vi "Telemetry2022.vi"() -> ()   [LabVIEW 2017]
uses:
  <vilib>/xnet/xnet.llb/XNET Frame CAN.ctl
  <vilib>/xnet/xnet.llb/XNET Frame Type CAN.ctl
  <vilib>/Instr/_visa.llb/VISA Configure Serial Port (Instr).vi
  <vilib>/xnet/xnet.llb/XNET Read (Frame CAN).vi
  <resource>/objmgr/xnet.rc
panel:
  out "x-y":u8
  out "serial in 2":u8[][](array[numeric]) format="%x"
  out "deleted portion 2":u8[](array[numeric]) format="%x"
  out "buffer":string
  out "Car orient":dbl
  out "Car pos":dbl[](array[numeric])
  out "Temp inv FL":dbl
  in  "ID":i32
  in  "Volt id":i32
  out "HV Volt Alert":bool
  out "HV Temp Alert":bool
  in  "Temp":dbl=45.0
  in  "Voltage [mV]":dbl=4200.0
  in  "Temp Id":i32
  out "Temp inv RR":dbl
  out "Temp inv RL":dbl
  out "Temp inv FR":dbl
  out "signal names":string[](array[string])
  in  "Signal indexes":T1
  in  "?":T2(tab)
  in  "Start Telemetry":bool
  in  "Data source":u16(ring) items=["WiFi-UDP", "XNET-USB", "CAN-USB", "Log Replay", "Serial"]
  in  "Main timestep":u32=2
  out "Is running":bool
  out "CAN2 Frame to signal":errorcluster
  out "CAN1 Frame to signal":errorcluster
  out "XNET error (Intf 2)":errorcluster
  out "XNET error (Intf 1)":errorcluster
  out "NI-CAN1 error":errorcluster {"code" format="%.0x"}
  out "NI-CAN0 error":errorcluster {"code" format="%.0x"}
  out "UDP Read error":errorcluster
  in  "Port":u16=8998
  out "Discarding":bool
  out "Discard count":i32
  out "Key Navigation error":errorcluster
  in  "Reset Keyboard":bool
  out "Key":T3(ring)
  out "Actual Timestep":u32(graph)
  out "Frames read":i32(graph)
  out "serial error":errorcluster
  in  "timeout ms":u32=1000
  in  "baud":u32=230400
  in  "Port":refnum<visa-resource-name>
  in  "Enable Termination\nChar":bool
  in  "termination char\n(0xA = '\\n' = LF)":u8=10 format="%.0x"
  in  "stop bits":u16(ring)=10 items=["1.0"=10, "1.5"=15, "2.0"=20]
  in  "data bits":u16=8 min=5 max=8 step=1
  in  "max buffer size":u32=200
  in  "parity":u16(ring) items=["None", "Odd", "Even", "Mark", "Space"]
  in  "flow control":T4(ring)
  out "RSSI [dBm]":i16
  out "Intf2":refnum<k21>
  out "Intf1":refnum<k21>
  out "Active intfs":i32
  out "APPS 1":dbl
  out "APPS 2":dbl
  out "BPS Rear":dbl
  out "BPS Front":dbl
  out "STA 2":dbl
  out "STA 1":dbl
  out "PPS 2":dbl
  out "PPS 1":dbl
  out "Dial4":i8(knob) scale=1.0..12.0
  out "Dial3":i8(knob) scale=1.0..12.0
  out "Dial2":i8(knob) scale=1.0..12.0
  out "Dial1":i8(knob) scale=1.0..12.0
  out "Dial5":i8(knob) scale=1.0..12.0
  out "Steering display":string
  out "Boolean 4":bool
  out "Boolean 3":bool
  out "Boolean 2":bool
  out "Boolean":bool
  out "Drv Torque Mult":dbl
  out "Brk Torque Mult":dbl
  out "Yaw Ctrl P":dbl
  out "Power Max":dbl
  out "Yaw Ctrl Balance":dbl
  out "Torque Demand":dbl
  out "FL Torque Limit":dbl
  out "FR Torque Limit":dbl
  out "RL Torque Limit":dbl
  out "RR Torque Limit":dbl
  out "FlashSubzoneError":bool=TRUE
  out "CSR2OtpError":bool=TRUE
  out "CSR1OtpError":bool=TRUE
  out "Output2OvpError":bool=TRUE
  out "Output1OvpError":bool=TRUE
  out "LVUvpInError":bool=TRUE
  out "LVUvpAlimAuxError":bool=TRUE
  out "LVOvpInError":bool=TRUE
  out "HVOcpError":bool=TRUE
  out "HVError":bool=TRUE
  out "CANError":bool=TRUE
  out "BB3OtpError":bool=TRUE
  out "BB2OtpError":bool=TRUE
  out "BB1OtpError":bool=TRUE
  out "STA2_OV":u8(slide) scale=0.0..180.0
  out "STA1_OV":u8(slide) scale=0.0..180.0
  out "PPS2_OV":u8(slide) scale=0.0..10.0
  out "PPS1_OV":u8(slide) scale=0.0..10.0
  out "APPS2_OV":u8(slide) scale=0.0..100.0
  out "APPS1_OV":u8(slide) scale=0.0..100.0
  out "BPS_rear_OV":u8(slide) scale=0.0..700.0
  out "BPS_front_OV":u8(slide) scale=0.0..700.0
  out "SC ENDLINE":dbl
  out "BFS [N]":dbl
  out "Place Opened":string
  out "BPSR_bool_OV":bool
  out "BPSF_bool_OV":bool
  out "BFS_bool_OV":bool
  out "STA_plaus":bool
  out "APPS_plaus":bool
  out "APPS1_bool":bool
  out "APPS2_bool":bool
  out "STA1_bool":bool
  out "STA2_bool":bool
  out "Speed [km/h]":dbl(knob) scale=0.0..110.0
  out "ASMS":bool
  out "RES GO":bool
  out "ASSI State":string
  out "AS State":string
  out "Car State":string
  out "RR":dbl[](array[numeric])
  out "FL":dbl[](array[numeric])
  out "FR":dbl[](array[numeric])
  out "RL":dbl[](array[numeric])
  out "Actual_vel_FL_OV":dbl
  out "Actual_vel_FR_OV":dbl
  out "Actual_vel_RL_OV":dbl
  out "Actual_vel_RR_OV":dbl
  out "Accel X":dbl
  out "Accel Y":dbl
  out "Yaw rate":dbl
  out "g-g Graph":cluster{dbl[], dbl[]}[](graph)
  out "HV":u32(colorbox)=9868950
  out "IMD":u32(colorbox)=9868950
  out "AMS":u32(colorbox)=9868950
  out "ASB":u32(colorbox)=9868950
  out "MCU1":u32(colorbox)=9868950
  out "MCU3":u32(colorbox)=9868950
  out "MCU4":u32(colorbox)=9868950
  out "MCU2":u32(colorbox)=9868950
  out "TCU":u32(colorbox)=9868950
  out "TS OFF":u32(colorbox)=9868950
  out "SoC":dbl
  out "HV Power out":dbl
  out "Max Temp":dbl
  out "Min Voltage":dbl
  out "VDC DV mode":bool
  out "RSSI [dBm]":i16
  out "EPOS Status":dbl
  out "EPOS Torque":dbl
  out "EPOS Position":dbl
  out "MCU State":string
  out "EPOS State":string
  out "RR Target Velocity":dbl
  out "FR Target Velocity":dbl
  out "RL Target Velocity":dbl
  out "FL Target Velocity":dbl
  out "Slip Ctrl I":dbl
  out "Optimal Slip":dbl
  out "Slip Ctrl D":dbl
  out "Slip Ctrl P":dbl
  out "Track Length":dbl
  out "Laps":dbl
  out "Target Soc":dbl
  out "Velocity X [km/h]":dbl
  out "Powlim Efficiency":bool
  out "Powlim Torque":bool
  out "Powlim Throttle":bool
  out "Powlim Hardcore":bool
  out "Traction Ctrl On":bool
  out "Slip Ctrl On":bool
  out "RR Torque Limit -":dbl
  out "RR Torque Limit +":dbl
  out "RL Torque Limit -":dbl
  out "RL Torque Limit +":dbl
  out "FR Torque Limit +":dbl
  out "FR Torque Limit -":dbl
  out "FL Torque Limit -":dbl
  out "FL Torque Limit +":dbl
  out "Target Steer":dbl(graph)
  out "Torque":T5(graph)
  out "Torque Demand":dbl(graph)
  out "Fz FL":dbl
  out "Fz FR":dbl
  out "Fz RL":dbl
  out "Fz RR":dbl
  out "Safety mode":bool
  out "M Yaw Limit":dbl
  out "M Yaw":dbl
  out "Yaw Ctrl Weight":dbl
  out "Drv Torque Mult":dbl
  out "Brk Torque Mult":dbl
  out "Yaw Ctrl P":dbl
  out "Yaw Ctrl Balance":dbl
  out "Efficiency Tune":dbl
  out "Launch Ctrl Mu":dbl
  out "Drop Param":dbl
  out "Drop Param New":dbl
  out "TC Threshold":dbl
  out "Powlim Approx":dbl
  out "Power Max":dbl
  out "RPM Max":dbl
  out "Max Motor Torque":dbl
  out "Lateral Balance":dbl
  out "Brake Force Max":dbl
  out "Throttle Breakpoint":dbl
  out "Static Weight Dist":dbl
  out "TCU CPU Usage":dbl
  out "Temp Inv RR":dbl
  out "Temp Inv RL":dbl
  out "Temp Inv FR":dbl
  out "Temp Inv FL":dbl
  out "Temp Motor RR":dbl
  out "Temp IGBT RR":dbl
  out "Error info RR":dbl
  out "Im RR":dbl
  out "It RR":dbl
  out "Temp Motor RL":dbl
  out "Temp IGBT RL":dbl
  out "Error info RL":dbl
  out "Im RL":dbl
  out "It RL":dbl
  out "Temp Motor FR":dbl
  out "Temp IGBT FR":dbl
  out "Error info FR":dbl
  out "Im FR":dbl
  out "It FR":dbl
  out "Temp Motor FL":dbl
  out "Temp IGBT FL":dbl
  out "Error info FL":dbl
  out "Im FL":dbl
  out "It FL":dbl
  out "RR Status":bool[](array[boolean])
  out "RR Inverter On":bool
  out "RR Error Reset":bool
  out "RR Enable":bool
  out "RR DC On":bool
  out "RL Status":bool[](array[boolean])
  out "RL Inverter On":bool
  out "RL Error Reset":bool
  out "RL Enable":bool
  out "RL DC On":bool
  out "FR Status":bool[](array[boolean])
  out "FR Inverter On":bool
  out "FR Error Reset":bool
  out "FR Enable":bool
  out "FR DC On":bool
  out "FL Status":bool[](array[boolean])
  out "FL Inverter On":bool
  out "FL Error Reset":bool
  out "FL Enable":bool
  out "FL DC On":bool
  out "Temp Inverter °C":T5(graph)
  out "MCU Actual Velocity 1/min":T5(graph)
  out "SC ENDLINE":dbl
  out "BSPD Actual":bool=TRUE
  out "DV Actual":bool=TRUE
  out "DV RELAY Actual":bool=TRUE
  out "EBS Actual":bool=TRUE
  out "FRONT Actual":bool=TRUE
  out "HOOP Actual":bool=TRUE
  out "MCU Actual":bool=TRUE
  out "BSPD Stored":bool
  in  "Ack BPSD":bool
  out "DV Stored":bool
  in  "Ack DV":bool
  out "DV RELAY Stored":bool
  in  "Ack DV RELAY":bool
  out "EBS Stored":bool
  in  "Ack EBS":bool
  out "FRONT Stored":bool
  in  "Ack FRONT":bool
  out "HOOP Stored":bool
  in  "Ack HOOP":bool
  out "MCU Stored":bool
  in  "Ack MCU":bool
  out "Temp SR2":dbl
  out "Temp SR1":dbl
  out "Temp BB3":dbl
  out "Temp BB2":dbl
  out "Temp BB1":dbl
  out "LV mAh":dbl
  out "Current IO Unbalance":dbl
  out "Output Overload Count":dbl
  out "HV Current In":dbl
  out "HV Voltage In":dbl
  out "CH1 Requested":bool
  out "CH2 Requested":bool
  out "Regen On":bool
  out "Umbilical On":bool
  out "CH1 Current Limit":dbl
  out "CH2 Current Limit":dbl
  out "HV Current Limit":dbl
  out "HV Voltage Setpoint":dbl
  out "CH2 Voltage Setpoint":dbl
  out "CH1 Voltage Setpoint":dbl
  out "Current Out Min 1":dbl
  out "Current Out Max 1":dbl
  out "Voltage Out Min 1":dbl
  out "Voltage Out Max 1":dbl
  out "Current Out Min 2":dbl
  out "Current Out Max 2":dbl
  out "Voltage Out Min 2":dbl
  out "Voltage Out Max 2":dbl
  out "Channel powers":cluster{dbl, dbl}(graph)={-0.16021728515625, 0.50628662109375}
  out "Channel voltages":cluster{dbl, dbl}(graph)={-0.16021728515625, 0.50628662109375}
  out "Channel currents":cluster{dbl, dbl}(graph)={-0.16021728515625, 0.50628662109375}
  out "HVDET2":bool
  out "PC Error":bool=TRUE
  out "TS-OV":bool
  out "IMD Relay":bool
  out "AMS Relay":bool
  out "AIR-":bool
  out "TSAL":bool
  out "TS-OC":bool
  out "AIR+":bool
  out "HVDET":bool
  out "AMS Error":bool=TRUE
  out "IMD Error":bool=TRUE
  out "TSAL Error":bool=TRUE
  out "OT":bool
  out "UV":bool
  out "OV":bool
  in  "HV T Alert":bool
  in  "Alert Max [xC]":dbl=450.0
  in  "HV V Alert":bool
  in  "Alert Max [xV]":dbl=4200.0
  in  "Alert Min [xV]":dbl
  out "Temp 8":dbl[](array[numeric])
  out "Temp 7":dbl[](array[numeric])
  out "Cell 6":cluster{"V-Value":dbl, dbl}[](array[cluster]) {"V-Slide" scale=0.0..6000.0}
  out "Temp 6":dbl[](array[numeric])
  out "Cell 5":cluster{"V-Value":dbl, dbl}[](array[cluster]) {"V-Slide" scale=0.0..6000.0}
  out "Temp 5":dbl[](array[numeric])
  out "Cell 4":cluster{"V-Value":dbl, dbl}[](array[cluster]) {"V-Slide" scale=0.0..6000.0}
  out "Temp 4":dbl[](array[numeric])
  out "Temp 3":dbl[](array[numeric])
  out "Cell 3":cluster{"V-Value":dbl, dbl}[](array[cluster]) {"V-Slide" scale=0.0..6000.0}
  out "Temp 2":dbl[](array[numeric])
  out "Cell 2":cluster{"V-Value":dbl, dbl}[](array[cluster]) {"V-Slide" scale=0.0..6000.0}
  out "Temp":dbl[](array[numeric])
  out "Cell":cluster{"V-Value":dbl, dbl}[](array[cluster]) {"V-Slide" scale=0.0..6000.0}
  out "Min Voltage Calc":dbl
  out "Max Temp Calc":dbl
  out "Min Voltage":dbl
  out "Max Temp":dbl
  out "Max Voltage":dbl
  out "SoC [mAh]":dbl
  out "Before":dbl
  out "After":dbl
  out "HV Current":dbl
  out "Charging State":string
  out "Heatmap":u32[][](array[colorbox])
  in  "Colors":u32[](array[colorbox])=[16448250, 16860, 711680, 16776960, 16025344, 16711680, 16189919, 0]
  in  "Ranges":i32[](array[numeric])=[1, 20, 30, 35, 40, 45, 50]
  in  "OK Button":bool
  out "Yaw Rear Vectornav":dbl
  out "AccY Rear":dbl
  out "AccX Rear":dbl
  out "BPS_Graph":cluster{dbl, dbl}(graph)={-0.16021728515625, 0.50628662109375}
  out "Target vs Actual steer\nSteer":cluster{dbl, dbl}(graph)={-0.16021728515625, 0.50628662109375}
  out "Target vs Actual Velocity":cluster{dbl, dbl}(graph)={-0.16021728515625, 0.50628662109375}
  out "HV Power out [W]":dbl(graph)
  out "Plausability":bool
  out "Validity":bool=TRUE
  out "APPS Avg":u8(slide) scale=0.0..100.0
  out "BFS_graph [N]":dbl(graph)
  out "STA Avg":u8(slide) scale=0.0..210.0
  out "Plausability":bool
  out "Validity":bool=TRUE
  out "g-g Graph 3":cluster{dbl[], dbl[]}[](graph)
  out "AccX Front":dbl
  out "AccY Front":dbl
  out "Roll Front":dbl
  out "Yaw Front":dbl
  out "Yaw Rear":dbl
  out "HV Current graph":dbl(graph)
  out "BFS Offset":dbl
  out "BPS Rear":dbl
  out "STA2":dbl
  out "APPS2":dbl
  out "PPS2":dbl
  out "BPS Front":dbl
  out "STA1":dbl
  out "APPS1":dbl
  out "PPS1":dbl
  out "STA2 Validity":bool
  out "APPS1 Validity":bool
  out "APPS2 Validity":bool
  out "STA1 Validity":bool
  out "BFS Validity":bool
  out "BPS Front Validity":bool
  out "BPS Rear Validity":bool
  out "XLAT":bool
  out "MODE":bool
  out "BLANK":bool
  out "START":bool
  out "ON":bool
  out "OFF":bool
  out "MCU Rear":bool
  out "MCU Front":bool
  out "MCU RF":bool
  out "MCU EF":bool
  out "TCU Heartbeat Error":bool=TRUE
  out "Steering Heartbeat Error":bool=TRUE
  out "Pedal Node Heartbeat Error":bool=TRUE
  out "MCU Heartbeat Error":bool=TRUE
  out "HVECU Heartbeat Error":bool=TRUE
  out "Dash Heartbeat Error":bool=TRUE
  out "HV":u32(colorbox)=9868950
  out "IMD":u32(colorbox)=9868950
  out "AMS":u32(colorbox)=9868950
  out "ASB":u32(colorbox)=9868950
  out "MCU1":u32(colorbox)=9868950
  out "MCU3":u32(colorbox)=9868950
  out "MCU4":u32(colorbox)=9868950
  out "MCU2":u32(colorbox)=9868950
  out "TCU":u32(colorbox)=9868950
  out "TS OFF":u32(colorbox)=9868950
  out "Brake Light":bool
  out "STA1 Max":dbl
  out "STA1 Min":dbl
  out "STA2 Max":dbl
  out "STA2 Min":dbl
  out "APPS1 Max":dbl
  out "APPS1 Min":dbl
  out "APPS2 Max":dbl
  out "APPS2 Min":dbl
  out "SC ENDLINE":dbl
  out "Rotary5 Timeout":bool=TRUE
  out "Rotary4 Timeout":bool=TRUE
  out "Rotary1 Timeout":bool=TRUE
  out "Rotary2 Timeout":bool=TRUE
  out "Rotary3 Timeout":bool=TRUE
  out "Rotary5 Validity":bool=TRUE
  out "Rotary4 Validity":bool=TRUE
  out "Rotary3 Validity":bool=TRUE
  out "Rotary2 Validity":bool=TRUE
  out "Rotary1 Validity":bool=TRUE
  out "Button4 Validity":bool=TRUE
  out "Button3 Validity":bool=TRUE
  out "Button2 Validity":bool=TRUE
  out "Button1 Validity":bool=TRUE
  out "BFS Timeout":bool=TRUE
  out "APPS2 Timeout":bool=TRUE
  out "APPS1 Timeout":bool=TRUE
  out "BPS Rear Timeout":bool=TRUE
  out "AccY Rear Timeout":bool=TRUE
  out "AccY FrontTimeout":bool=TRUE
  out "BPS Front Timeout":bool=TRUE
  out "AccX Rear Timeout":bool=TRUE
  out "AccX Front Timeout":bool=TRUE
  out "SC Endline Timeout":bool=TRUE
  out "ASB Error":bool=TRUE
  out "SC Endline Validity":bool=TRUE
  out "HV Current Timeout":bool=TRUE
  out "HV Cell Temp Timeout":bool=TRUE
  out "SC Endline":bool=TRUE
  out "OT":bool=TRUE
  out "OV":bool=TRUE
  out "UV":bool=TRUE
  out "HV Cell Temp Validity":bool=TRUE
  out "HV Cell Voltage Validity":bool=TRUE
  out "IMD Error":bool=TRUE
  out "AMS Error":bool=TRUE
  out "PC Error":bool=TRUE
  out "TSAL Error":bool=TRUE
  out "HV Current Validity":bool=TRUE
  out "HV Voltage Validity":bool=TRUE
  out "AccY Rear Validity":bool=TRUE
  out "Accy Front Validity":bool=TRUE
  out "APPS1 Validity":bool=TRUE
  out "STA1 Validity":bool=TRUE
  out "BPS Front Validity":bool=TRUE
  out "AccX Rear Validity":bool=TRUE
  out "AccX Front Validity":bool=TRUE
  out "STA Plausability":bool
  out "APPS Plausability":bool
  out "BFS Validity":bool=TRUE
  out "APPS2 Validity":bool=TRUE
  out "STA2 Validity":bool=TRUE
  out "Yaw Front Validity":bool=TRUE
  out "Yaw Rear Validity":bool=TRUE
  out "BPS Rear Validity":bool=TRUE
  out "FL Error info":dbl
  out "FR Error info":dbl
  out "RL Error info":dbl
  out "RR Error info":dbl
  out "FlashSubzoneError":bool=TRUE
  out "CSR2OtpError":bool=TRUE
  out "CSR1OtpError":bool=TRUE
  out "Output2OvpError":bool=TRUE
  out "Output1OvpError":bool=TRUE
  out "LVUvpInError":bool=TRUE
  out "LVUvpAlimAuxError":bool=TRUE
  out "LVOvpInError":bool=TRUE
  out "HVOcpError":bool=TRUE
  out "HVError":bool=TRUE
  out "CANError":bool=TRUE
  out "BB3OtpError":bool=TRUE
  out "BB2OtpError":bool=TRUE
  out "BB1OtpError":bool=TRUE
  out "DV Target Angle Validity":bool=TRUE
  out "SSG Status1 Timeout":bool=TRUE
  out "DV Target Speed Validity":bool=TRUE
  out "Xavier Timeout":bool=TRUE
  out "Bag Start":bool
  out "Loop Closed":bool
  out "Mission Finished":bool
  out "Eff n Particles":dbl
  out "Updates last resample":dbl
  out "Runtime":dbl
  out "HeadingSS-Yaw":cluster{"Data":dbl, "Data":dbl}(graph)
  out "Heading-Steering-Crosstrack":cluster{"Data":dbl, "Data":dbl, "Data":dbl}(graph)
  out "Target laps":dbl
  out "Current laps":dbl
  out "Xavier Power [W]":dbl
  out "Xavier Max Temp [°C]":dbl
  out "CPU8":u8(slide) scale=0.0..100.0
  out "CPU7":u8(slide) scale=0.0..100.0
  out "CPU6":u8(slide) scale=0.0..100.0
  out "CPU5":u8(slide) scale=0.0..100.0
  out "CPU4":u8(slide) scale=0.0..100.0
  out "CPU3":u8(slide) scale=0.0..100.0
  out "CPU2":u8(slide) scale=0.0..100.0
  out "CPU1":u8(slide) scale=0.0..100.0
  out "RAM":u8(slide) scale=0.0..31.0
  out "Initial Checkup":string
  out "Mission selected":string
  out "Car State":string
  out "ASSI State":string
  out "AS State":string
  out "Driving State Active":bool
  out "nEBS Acitve":bool
  out "EBS Active":bool
  out "Finish State":bool
  out "Target Steer 2":dbl(graph)
  out "Target Speed":dbl(graph)
  out "ASMS":bool
  out "ASB":u32(colorbox)=9868950
  out "Inspection":u32(colorbox)=9868950
  out "Skidpad":u32(colorbox)=9868950
  out "Trackdrive":u32(colorbox)=9868950
  out "Red count":dbl
  out "Orange count":dbl
  out "Blue count":dbl
  out "Yellow count":dbl
  out "Current landmarks":dbl
  out "All landmarks":dbl
  out "Map":cluster{dbl[], dbl[]}[](graph)
  in  "Arrow thickness":dbl=0.15 format="%#_13g"
  in  "Arrow size":dbl=5.0 format="%#_13g"
  in  "Export":bool
  out "Lap                    Laptime                        SoC                 Current Avg |                             Motor Temperatures                            |                            Inverter Temperatures":T6(array[cluster]) {"Laptime" format="%<%M:%S%2u>T"}
  in  "Laptrigger":bool
  in  "Reset":bool
  in  "Lapdata disp":bool=TRUE
  out "Inverter Temp":cluster{i32[], dbl[]}[](graph)
  out "Motor Temp":cluster{i32[], dbl[]}[](graph)
  # "STA1"
  # "STA2"
  # "PPS\n1      2"
  # "APPS\n1      2"
  # "BPS\nF      R"
  # "APPS1"
  # "APPS2"
  # "STA1"
  # "STA2"
  # "BFS"
  # "BPS F"
  # "BPS R"
  # "Error Info"
  # "Temp IGBT °C"
  # "Temp Inverter °C"
  # "Temp Motor °C"
  # "Actual Velocity [rpm]"
  # "SysReady"
  # "Error"
  # "Warn"
  # "QuitDcOn"
  # "DcOn"
  # "QuitInvOn"
  # "InverterOn"
  # "Derating"
  # "SysReady"
  # "Error"
  # "Warn"
  # "QuitDcOn"
  # "DcOn"
  # "QuitInvOn"
  # "InverterOn"
  # "Derating"
  # "SysReady"
  # "Error"
  # "Warn"
  # "QuitDcOn"
  # "DcOn"
  # "QuitInvOn"
  # "InverterOn"
  # "Derating"
  # "SysReady"
  # "Error"
  # "Warn"
  # "QuitDcOn"
  # "DcOn"
  # "QuitInvOn"
  # "InverterOn"
  # "Derating"
  # "-inf"
  # "inf"
  # "-"
  # "+"
  # "-"
  # "-"
  # "+"
  # "+"
  # "-"
  # "-"
  # "+"
  # "+"
  # "-"
  # "-"
  # "+"
  # "+"
  # "-"
  # "-"
  # "+"
  # "+"
  # "-"
  # "-"
  # "+"
  # "+"
  # "-"
  # "-"
  # "+"
  # "ADCs"
  # "Sensors"
  # "Dashboard"
  # "MCU"
  # "Heartbeats"
  # "System"
  # "EEPROMS"
  # "Brightloop"
  # "Sensor validity"
  # "HV Errors"
  # "Steering wheel"
  # "Sensor Timeout"
  # "System"
  # "AMK Errors"
  # "1         CPU Usage         8"
  # "RAM"
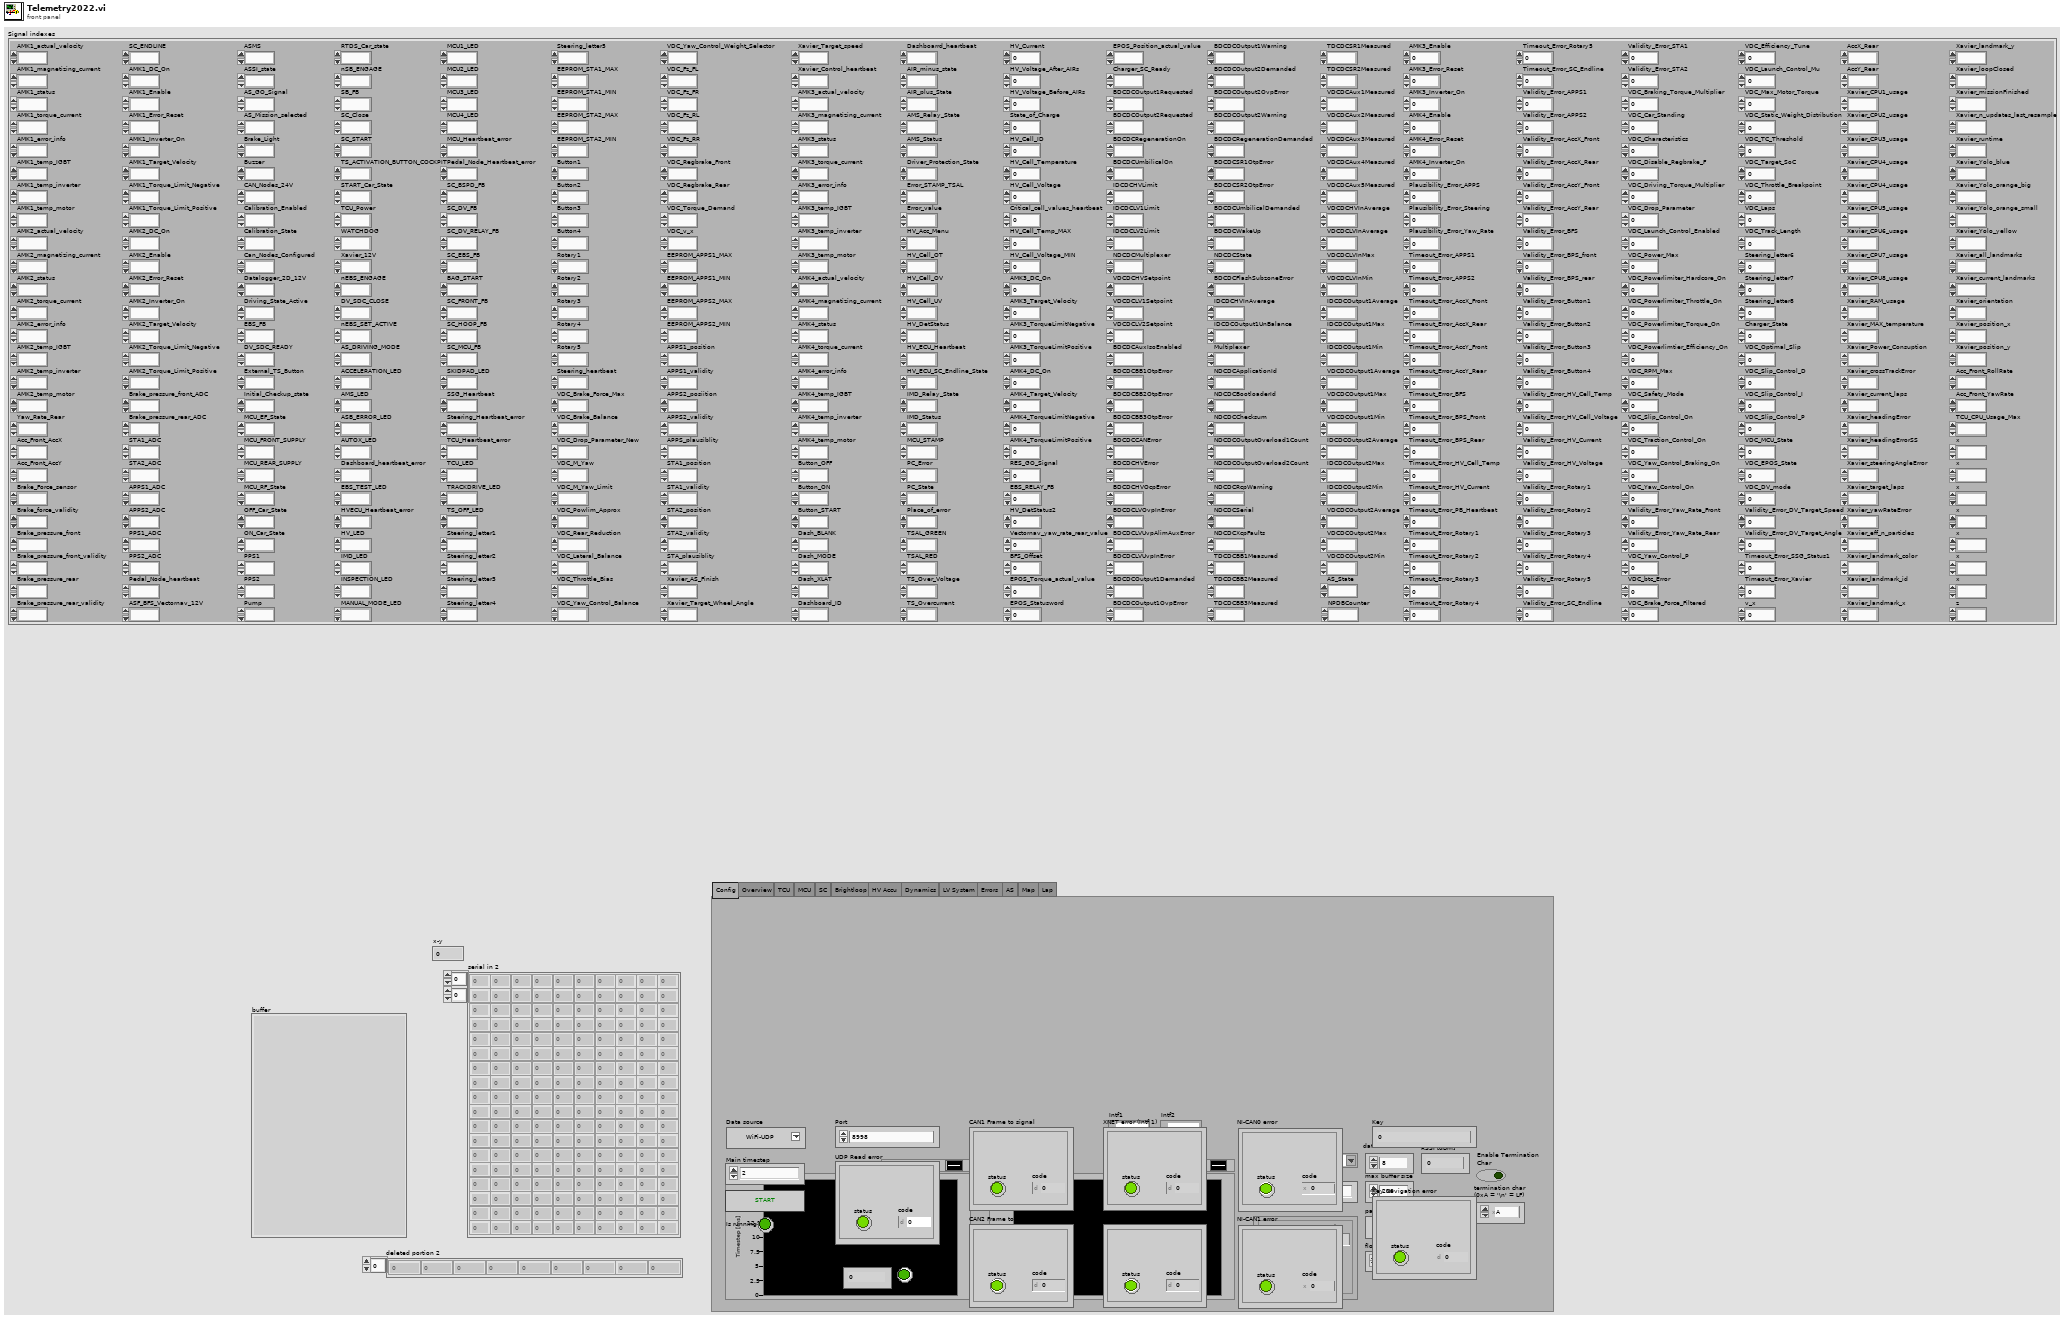
[diagram p1: front panel]
types:
  T1 = cluster{"AMK1_actual_velocity":dbl, "AMK1_magnetizing_current":dbl, "AMK1_status":dbl, "AMK1_torque_current":dbl, "AMK1_error_info":dbl, "AMK1_temp_IGBT":dbl, "AMK1_temp_inverter":dbl, "AMK1_temp_motor":dbl, "AMK2_temp_motor":dbl, "AMK2_actual_velocity":dbl, "AMK2_magnetizing_current":dbl, "AMK2_status":dbl, "AMK2_torque_current":dbl, "AMK2_error_info":dbl, "AMK2_temp_IGBT":dbl, "AMK2_temp_inverter":dbl, "Yaw_Rate_Rear":dbl, "Brake_pressure_rear_validity":dbl, "Acc_Front_AccX":dbl, "Acc_Front_AccY":dbl, "Brake_Force_sensor":dbl, "Brake_force_validity":dbl, "Brake_pressure_front":dbl, "Brake_pressure_front_validity":dbl, "Brake_pressure_rear":dbl, "SC_ENDLINE":dbl, "AMK1_DC_On":dbl, "AMK1_Enable":dbl, "AMK1_Error_Reset":dbl, "AMK1_Inverter_On":dbl, "AMK1_Target_Velocity":dbl, "AMK1_Torque_Limit_Negative":dbl, "AMK1_Torque_Limit_Positive":dbl, "Brake_pressure_front_ADC":dbl, "AMK2_DC_On":dbl, "AMK2_Enable":dbl, "AMK2_Error_Reset":dbl, "AMK2_Inverter_On":dbl, "AMK2_Target_Velocity":dbl, "AMK2_Torque_Limit_Negative":dbl, "AMK2_Torque_Limit_Positive":dbl, "Brake_pressure_rear_ADC":dbl, "ASF_BFS_Vectornav_12V":dbl, "STA1_ADC":dbl, "STA2_ADC":dbl, "APPS1_ADC":dbl, "APPS2_ADC":dbl, "PPS1_ADC":dbl, "PPS2_ADC":dbl, "Pedal_Node_heartbeat":dbl, "PPS2":dbl, "PPS1":dbl, "ON_Car_State":dbl, "OFF_Car_State":dbl, "MCU_RF_State":dbl, "MCU_REAR_SUPPLY":dbl, "MCU_FRONT_SUPPLY":dbl, "Pump":dbl, "MCU_EF_State":dbl, "External_TS_Button":dbl, "DV_SDC_READY":dbl, "EBS_FB":dbl, "Driving_State_Active":dbl, "Datalogger_2D_12V":dbl, "Can_Nodes_Configured":dbl, "Calibration_State":dbl, "Initial_Checkup_state":dbl, "Calibration_Enabled":dbl, "CAN_Nodes_24V":dbl, "Buzzer":dbl, "Brake_Light":dbl, "AS_Mission_selected":dbl, "AS_GO_Signal":dbl, "ASSI_state":dbl, "ASMS":dbl, "Dash_XLAT":dbl, "Dash_MODE":dbl, "Dash_BLANK":dbl, "Button_START":dbl, "Button_ON":dbl, "Button_OFF":dbl, "AMK4_temp_motor":dbl, "Dashboard_ID":dbl, "AMK4_temp_inverter":dbl, "AMK4_error_info":dbl, "AMK4_torque_current":dbl, "AMK4_status":dbl, "AMK4_magnetizing_current":dbl, "AMK4_actual_velocity":dbl, "AMK3_temp_motor":dbl, "AMK3_temp_inverter":dbl, "AMK4_temp_IGBT":dbl, "AMK3_temp_IGBT":dbl, "AMK3_error_info":dbl, "AMK3_torque_current":dbl, "AMK3_status":dbl, "AMK3_magnetizing_current":dbl, "AMK3_actual_velocity":dbl, "Xavier_Control_heartbeat":dbl, "Xavier_Target_speed":dbl, "INSPECTION_LED":dbl, "IMD_LED":dbl, "HV_LED":dbl, "HVECU_Heartbeat_error":dbl, "EBS_TEST_LED":dbl, "Dashboard_heartbeat_error":dbl, "AUTOX_LED":dbl, "MANUAL_MODE_LED":dbl, "ASB_ERROR_LED":dbl, "ACCELERATION_LED":dbl, "AS_DRIVING_MODE":dbl, "nEBS_SET_ACTIVE":dbl, "DV_SDC_CLOSE":dbl, "nEBS_ENGAGE":dbl, "Xavier_12V":dbl, "WATCHDOG":dbl, "AMS_LED":dbl, "TCU_Power":dbl, "START_Car_State":dbl, "TS_ACTIVATION_BUTTON_COCKPIT":dbl, "SC_START":dbl, "SC_Close":dbl, "SB_FB":dbl, "nSB_ENGAGE":dbl, "RTDS_Car_state":dbl, "Steering_letter3":dbl, "Steering_letter2":dbl, "Steering_letter1":dbl, "TS_OFF_LED":dbl, "TRACKDRIVE_LED":dbl, "TCU_LED":dbl, "TCU_Heartbeat_error":dbl, "Steering_letter4":dbl, "Steering_Heartbeat_error":dbl, "SKIDPAD_LED":dbl, "SC_MCU_FB":dbl, "SC_HOOP_FB":dbl, "SC_FRONT_FB":dbl, "BAG_START":dbl, "SC_EBS_FB":dbl, "SC_DV_RELAY_FB":dbl, "SSG_Heartbeat":dbl, "SC_DV_FB":dbl, "SC_BSPD_FB":dbl, "Pedal_Node_Heartbeat_error":dbl, "MCU_Heartbeat_error":dbl, "MCU4_LED":dbl, "MCU3_LED":dbl, "MCU2_LED":dbl, "MCU1_LED":dbl, "VDC_Throttle_Bias":dbl, "VDC_Lateral_Balance":dbl, "VDC_Rear_Reduction":dbl, "VDC_Powlim_Approx":dbl, "VDC_M_Yaw_Limit":dbl, "VDC_M_Yaw":dbl, "VDC_Drop_Parameter_New":dbl, "VDC_Yaw_Control_Balance":dbl, "VDC_Brake_Balance":dbl, "Steering_heartbeat":dbl, "Rotary5":dbl, "Rotary4":dbl, "Rotary3":dbl, "Rotary2":dbl, "Rotary1":dbl, "Button4":dbl, "VDC_Brake_Force_Max":dbl, "Button3":dbl, "Button2":dbl, "Button1":dbl, "EEPROM_STA2_MIN":dbl, "EEPROM_STA2_MAX":dbl, "EEPROM_STA1_MIN":dbl, "EEPROM_STA1_MAX":dbl, "Steering_letter5":dbl, "Xavier_AS_Finish":dbl, "STA_plausiblity":dbl, "STA2_validity":dbl, "STA2_position":dbl, "STA1_validity":dbl, "STA1_position":dbl, "APPS_plausiblity":dbl, "Xavier_Target_Wheel_Angle":dbl, "APPS2_validity":dbl, "APPS1_validity":dbl, "APPS1_position":dbl, "EEPROM_APPS2_MIN":dbl, "EEPROM_APPS2_MAX":dbl, "EEPROM_APPS1_MIN":dbl, "EEPROM_APPS1_MAX":dbl, "VDC_v_x":dbl, "APPS2_posiition":dbl, "VDC_Torque_Demand":dbl, "VDC_Regbrake_Rear":dbl, "VDC_Regbrake_Front":dbl, "VDC_Fz_RR":dbl, "VDC_Fz_RL":dbl, "VDC_Fz_FR":dbl, "VDC_Fz_FL":dbl, "VDC_Yaw_Control_Weight_Selector":dbl, "RES_GO_Signal":dbl, "AMK4_TorqueLimitPositive":dbl, "AMK4_TorqueLimitNegative":dbl, "AMK4_DC_On":dbl, "AMK3_TorqueLimitPositive":dbl, "AMK3_TorqueLimitNegative":dbl, "AMK3_Target_Velocity":dbl, "AMK3_DC_On":dbl, "HV_Cell_Voltage_MIN":dbl, "HV_Cell_Temp_MAX":dbl, "AMK4_Target_Velocity":dbl, "Critical_cell_values_heartbeat":dbl, "HV_Cell_Voltage":dbl, "HV_Cell_Temperature":dbl, "HV_Cell_ID":dbl, "State_of_Charge":dbl, "HV_Voltage_Before_AIRs":dbl, "HV_Voltage_After_AIRs":dbl, "HV_Current":dbl, "TS_Over_Voltage":dbl, "TSAL_RED":dbl, "TSAL_GREEN":dbl, "Place_of_error":dbl, "PC_State":dbl, "PC_Error":dbl, "MCU_STAMP":dbl, "TS_Overcurrent":dbl, "IMD_Status":dbl, "HV_ECU_SC_Endline_State":dbl, "HV_ECU_Heartbeat":dbl, "HV_DetStatus":dbl, "HV_Cell_UV":dbl, "HV_Cell_OV":dbl, "HV_Cell_OT":dbl, "HV_Acc_Menu":dbl, "IMD_Relay_State":dbl, "Error_value":dbl, "Error_STAMP_TSAL":dbl, "Driver_Protection_State":dbl, "AMS_Status":dbl, "AMS_Relay_State":dbl, "AIR_plus_State":dbl, "AIR_minus_state":dbl, "Dashboarrd_heartbeat":dbl, "BDCDCOutput1Demanded":dbl, "BDCDCLVUvpInError":dbl, "BDCDCLVUvpAlimAuxError":dbl, "BDCDCLVOvpInError":dbl, "BDCDCHVOcpError":dbl, "BDCDCHVError":dbl, "BDCDCCANError":dbl, "BDCDCOutput1OvpError":dbl, "BDCDCBB3OtpError":dbl, "BDCDCBB1OtpError":dbl, "BDCDCAuxIsoEnabled":dbl, "VDCDCLV2Setpoint":dbl, "VDCDCLV1Setpoint":dbl, "VDCDCHVSetpoint":dbl, "NDCDCMultiplexer":dbl, "IDCDCLV2Limit":dbl, "BDCDCBB2OtpError":dbl, "IDCDCLV1Limit":dbl, "IDCDCHVLimit":dbl, "BDCDCUmbilicalOn":dbl, "BDCDCRegenerationOn":dbl, "BDCDCOutput2Requested":dbl, "BDCDCOutput1Requested":dbl, "Charger_SC_Ready":dbl, "EPOS_Position_actual_value":dbl, "Vectornav_yaw_rate_rear_value":dbl, "EBS_RELAY_FB":dbl, "HV_DetStatus2":dbl, "BFS_Offset":dbl, "EPOS_Torque_actual_value":dbl, "EPOS_Statusword":dbl, "TDCDCBB2Measured":dbl, "TDCDCBB1Measured":dbl, "NDCDCXcpFaults":dbl, "NDCDCSerial":dbl, "NDCDCRcpWarning":dbl, "NDCDCOutputOverload2Count":dbl, "NDCDCOutputOverload1Count":dbl, "TDCDCBB3Measured":dbl, "NDCDCChecksum":dbl, "NDCDCApplicationId":dbl, "Multiplexer":dbl, "IDCDCOutput1UnBalance":dbl, "IDCDCHVInAverage":dbl, "BDCDCFlashSubzoneError":dbl, "NDCDCState":dbl, "BDCDCWakeUp":dbl, "NDCDCBootloaderId":dbl, "BDCDCUmbilicalDemanded":dbl, "BDCDCSR2OtpError":dbl, "BDCDCSR1OtpError":dbl, "BDCDCRegenerationDemanded":dbl, "BDCDCOutput2Warning":dbl, "BDCDCOutput2OvpError":dbl, "BDCDCOutput2Demanded":dbl, "BDCDCOutput1Warning":dbl, "VDCDCOutput2Min":dbl, "VDCDCOutput2Max":dbl, "VDCDCOutput2Average":dbl, "IDCDCOutput2Min":dbl, "IDCDCOutput2Max":dbl, "IDCDCOutput2Average":dbl, "VDCDCOutput1Min":dbl, "VDCDCOutput1Average":dbl, "IDCDCOutput1Min":dbl, "IDCDCOutput1Max":dbl, "IDCDCOutput1Average":dbl, "VDCDCLVInMin":dbl, "VDCDCLVInMax":dbl, "VDCDCLVInAverage":dbl, "VDCDCOutput1Max":dbl, "VDCDCHVInAverage":dbl, "VDCDCAux5Measured":dbl, "VDCDCAux4Measured":dbl, "VDCDCAux3Measured":dbl, "VDCDCAux2Measured":dbl, "VDCDCAux1Measured":dbl, "TDCDCSR2Measured":dbl, "TDCDCSR1Measured":dbl, "AS_State":dbl, "NPDBCounter":dbl, "Timeout_Error_Rotary3":dbl, "Timeout_Error_Rotary2":dbl, "Timeout_Error_Rotary1":dbl, "Timeout_Error_PB_Heartbeat":dbl, "Timeout_Error_HV_Current":dbl, "Timeout_Error_HV_Cell_Temp":dbl, "Timeout_Error_BPS_Rear":dbl, "Timeout_Error_Rotary4":dbl, "Timeout_Error_BPS_Front":dbl, "Timeout_Error_AccY_Rear":dbl, "Timeout_Error_AccY_Front":dbl, "Timeout_Error_AccX_Rear":dbl, "Timeout_Error_AccX_Front":dbl, "Timeout_Error_APPS2":dbl, "Timeout_Error_APPS1":dbl, "Plausibility_Error_Yaw_Rate":dbl, "Timeout_Error_BFS":dbl, "Plausibility_Error_Steering":dbl, "Plausibility_Error_APPS":dbl, "AMK4_Inverter_On":dbl, "AMK4_Error_Reset":dbl, "AMK4_Enable":dbl, "AMK3_Inverter_On":dbl, "AMK3_Error_Reset":dbl, "AMK3_Enable":dbl, "Timeout_Error_Rotary5":dbl, "Timeout_Error_SC_Endline":dbl, "Validity_Error_APPS1":dbl, "Validity_Error_APPS2":dbl, "Validity_Error_AccX_Front":dbl, "Validity_Error_AccX_Rear":dbl, "Validity_Error_AccY_Front":dbl, "Validity_Error_AccY_Rear":dbl, "Validity_Error_HV_Cell_Temp":dbl, "Validity_Error_BFS":dbl, "Validity_Error_BPS_front":dbl, "Validity_Error_BPS_rear":dbl, "Validity_Error_Button1":dbl, "Validity_Error_Button2":dbl, "Validity_Error_Button3":dbl, "Validity_Error_Button4":dbl, "Validity_Error_HV_Cell_Voltage":dbl, "Validity_Error_SC_Endline":dbl, "Validity_Error_HV_Current":dbl, "Validity_Error_HV_Voltage":dbl, "Validity_Error_Rotary1":dbl, "Validity_Error_Rotary2":dbl, "Validity_Error_Rotary3":dbl, "Validity_Error_Rotary4":dbl, "Validity_Error_Rotary5":dbl, "Validity_Error_STA1":dbl, "Validity_Error_STA2":dbl, "VDC_Braking_Torque_Multiplier":dbl, "VDC_Car_Standing":dbl, "VDC_Characteristics":dbl, "VDC_Disable_Regbrake_F":dbl, "VDC_Driving_Torque_Multiplier":dbl, "VDC_Drop_Parameter":dbl, "VDC_Safety_Mode":dbl, "VDC_Launch_Control_Enabled":dbl, "VDC_Power_Max":dbl, "VDC_Powerlimiter_Hardcore_On":dbl, "VDC_Powerlimiter_Throttle_On":dbl, "VDC_Powerlimiter_Torque_On":dbl, "VDC_Powerlimtier_Efficiency_On":dbl, "VDC_RPM_Max":dbl, "VDC_Slip_Control_On":dbl, "VDC_Brake_Force_Filtered":dbl, "VDC_Traction_Control_On":dbl, "VDC_Yaw_Control_Braking_On":dbl, "VDC_Yaw_Control_On":dbl, "Validity_Error_Yaw_Rate_Front":dbl, "Validity_Error_Yaw_Rate_Rear":dbl, "VDC_Yaw_Control_P":dbl, "VDC_btc_Error":dbl, "VDC_Efficiency_Tune":dbl, "VDC_Launch_Control_Mu":dbl, "VDC_Max_Motor_Torque":dbl, "VDC_Static_Weight_Distribution":dbl, "VDC_TC_Threshold":dbl, "VDC_Target_SoC":dbl, "VDC_Throttle_Breakpoint":dbl, "VDC_Laps":dbl, "VDC_Slip_Control_I":dbl, "VDC_Track_Length":dbl, "Steering_letter6":dbl, "Steering_letter7":dbl, "Steering_letter8":dbl, "Charger_State":dbl, "VDC_Optimal_Slip":dbl, "VDC_Slip_Control_D":dbl, "VDC_Slip_Control_P":dbl, "v_x":dbl, "VDC_MCU_State":dbl, "VDC_EPOS_State":dbl, "VDC_DV_mode":dbl, "Validity_Error_DV_Target_Speed":dbl, "Validity_Error_DV_Target_Angle":dbl, "Timeout_Error_SSG_Status1":dbl, "Timeout_Error_Xavier":dbl, "AccX_Rear":dbl, "AccY_Rear":dbl, "Xavier_CPU1_usage":dbl, "Xavier_CPU2_usage":dbl, "Xavier_CPU3_usage":dbl, "Xavier_CPU4_usage":dbl, "Xavier_CPU4_usage":dbl, "Xavier_CPU5_usage":dbl, "Xavier_current_laps":dbl, "Xavier_CPU6_usage":dbl, "Xavier_CPU7_usage":dbl, "Xavier_CPU8_usage":dbl, "Xavier_RAM_usage":dbl, "Xavier_MAX_temperature":dbl, "Xavier_Power_Consuption":dbl, "Xavier_crossTrackError":dbl, "Xavier_headingError":dbl, "Xavier_landmark_x":dbl, "Xavier_headingErrorSS":dbl, "Xavier_steeringAngleError":dbl, "Xavier_target_laps":dbl, "Xavier_yawRateError":dbl, "Xavier_eff_n_particles":dbl, "Xavier_landmark_color":dbl, "Xavier_landmark_id":dbl, "x":dbl, "x":dbl, "x":dbl, "x":dbl, "x":dbl, "x":dbl, "x":dbl, "z":dbl, "TCU_CPU_Usage_Max":dbl, "Acc_Front_RollRate":dbl, "Xavier_position_y":dbl, "Xavier_position_x":dbl, "Xavier_orientation":dbl, "Xavier_current_landmarks":dbl, "Xavier_all_landmarks":dbl, "Xavier_Yolo_yellow":dbl, "Acc_Front_YawRate":dbl, "Xavier_Yolo_orange_small":dbl, "Xavier_Yolo_orange_big":dbl, "Xavier_Yolo_blue":dbl, "Xavier_runtime":dbl, "Xavier_n_updates_last_resample":dbl, "Xavier_missionFinished":dbl, "Xavier_loopClosed":dbl, "Xavier_landmark_y":dbl}
  T2 = enum32{"Config", "Overview", "TCU", "MCU", "SC", "Brightloop", "HV Accu", "Dynamics", "LV System", "Errors", "AS", "Map", "Lap"}
  T3 = enum16{"0", "1", "2", "3", "4", "5", "6", "7", "8", "9", "A", "B", "C", "D", "E", "F", "G", "H", "I", "J", "K", "L", "M", "N", "O", "P", "Q", "R", "S", "T", "U", "V", "W", "X", "Y", "Z", "F1", "F2", "F3", "F4", "F5", "F6", "F7", "F8", "F9", "F10", "F11", "F12", "F13", "F14", "F15", "ADD", "BACK", "BACKSLASH", "CAPITAL", "COMMA", "DECIMAL", "DELETE", "DIVIDE", "DOWN", "END", "EQUALS", "ESCAPE", "GRAVE (`)", "HOME", "INSERT", "LBRACKET", "LCONTROL", "LEFT", "L ALT", "LSHIFT", "LWIN", "MINUS", "MULTIPLY", "NEXT", "NUMLOCK", "NUMPAD_0", "NUMPAD_1", "NUMPAD_2", "NUMPAD_3", "NUMPAD_4", "NUMPAD_5", "NUMPAD_6", "NUMPAD_7", "NUMPAD_8", "NUMPAD_9", "PAUSE", "PERIOD", "PRIOR (PG UP)", "RBRACKET", "RCONTROL", "RETURN", "RIGHT", "R ALT", "RSHIFT", "RWIN", "SCROLL", "SEMICOLON", "SLASH", "SPACE", "SUBTRACT", "TAB", "UP", "ENTER (num pad)", "' (quote)"}
  T4 = enum16{"None", "XON/XOFF", "RTS/CTS", "XON/XOFF & RTS/CTS", "DTR/DSR", "XON/XOFF & DTR/DSR"}
  T5 = cluster{"Data":dbl, "Actual_vel_FR_OV":dbl, "Actual_vel_RL_OV":dbl, "Actual_vel_RR_OV":dbl}
  T6 = cluster{"SoC":i32, "MotorTemp_FL":dbl, "MotorTemp_FR":dbl, "MotorTemp_RL":dbl, "MotorTemp_RR":dbl, "InverterTemp_FL":dbl, "InverterTemp_FR":dbl, "InverterTemp_RL":dbl, "InverterTemp_RR":dbl, "Laptime":timestamp, "Lap":i32, "Curr Abs Avg":dbl}[]
  T7 = typedef "XNET Frame CAN.ctl" = cluster{"timestamp":timestamp, "payload":u8[], "identifier":u32, "type":T8, "extended?":bool, "echo?":bool}
  T8 = typedef "XNET Frame Type CAN.ctl" = u8
  T9 = cluster{"Signal count":i32, "Conversion session":refnum<k21>, "Conversion error":errorcluster}
  T10 = cluster{"XNET session A":refnum<k21>, "Error out A ":errorcluster, "XNET session B":refnum<k21>, "Error out B":errorcluster}
  T11 = typedef "xobjhandle.ctl" = u32
  T12 = cluster{"ObjHandle A":T11, "Error out A":errorcluster, "ObjHandle B":T11, "Error out B":errorcluster}
  T13 = cluster{"Data":dbl, "Temp inv FR":dbl, "Temp inv RL":dbl, "Temp inv RR":dbl}
  T14 = cluster{"Data":dbl, "FR Torque Limit":dbl, "RL Torque Limit":dbl, "RR Torque Limit":dbl}
  T15 = cluster{"Color":i32, "Id":i32, "PosX":dbl, "PosY":dbl}
  T16 = cluster{"Color":i32, "Id":i32, "PosX":dbl, "PosY":dbl}[]
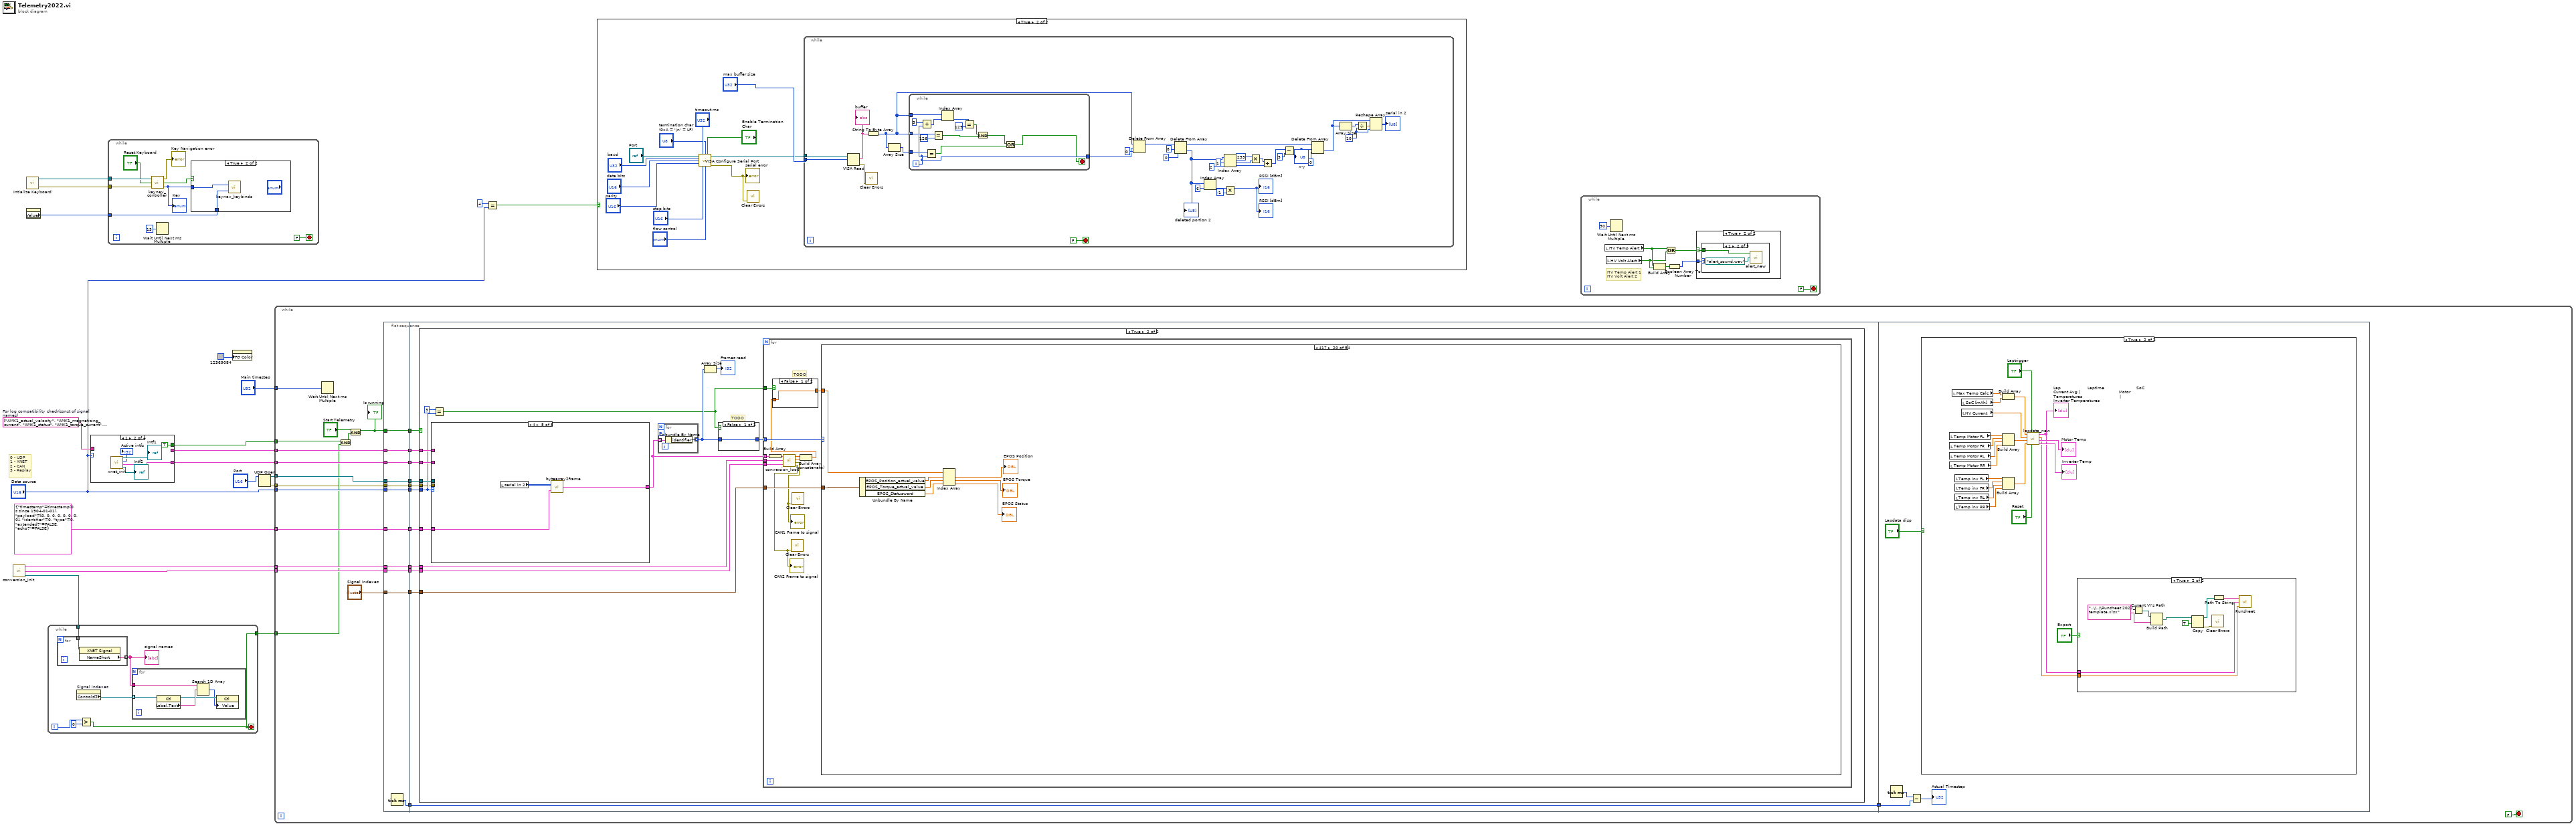
[diagram p0: block diagram]
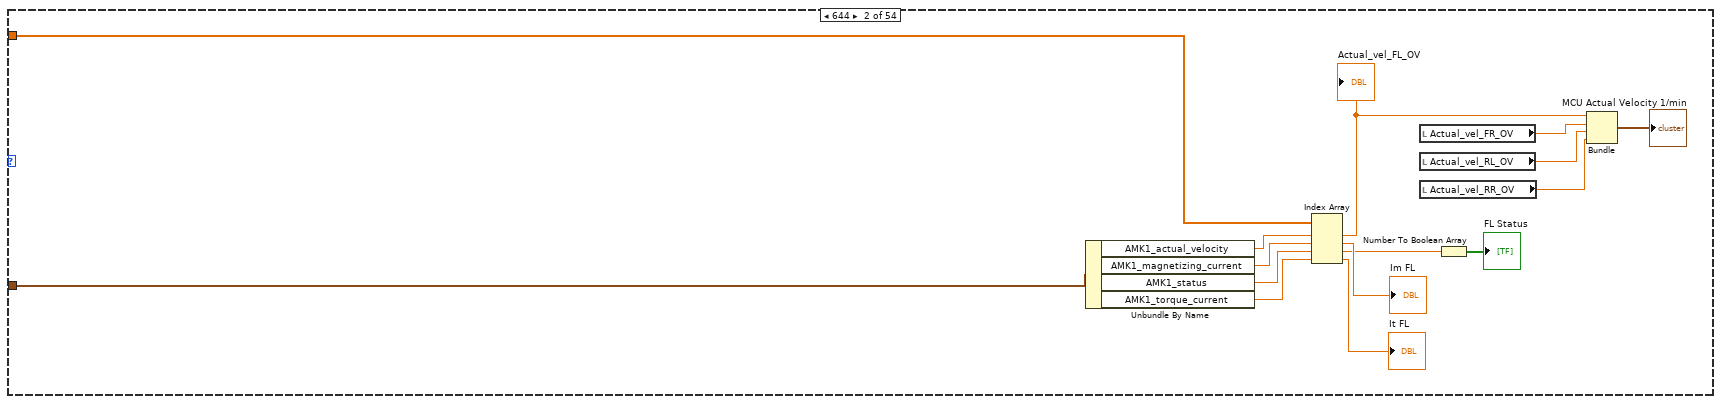
[diagram p7: hidden frame]
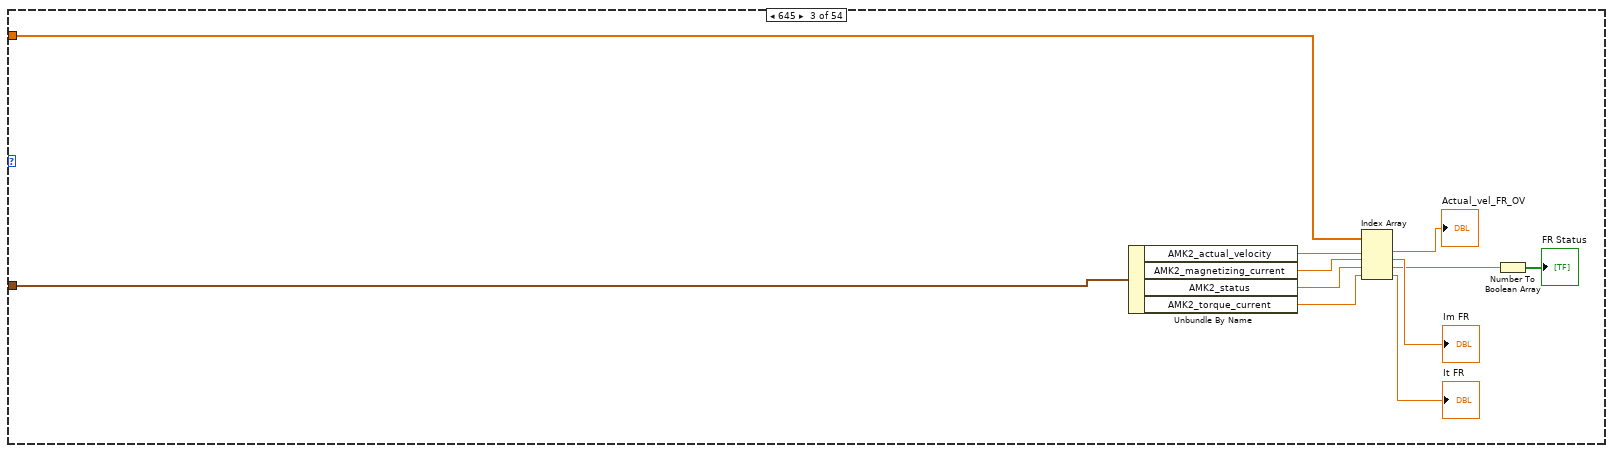
[diagram p8: hidden frame]
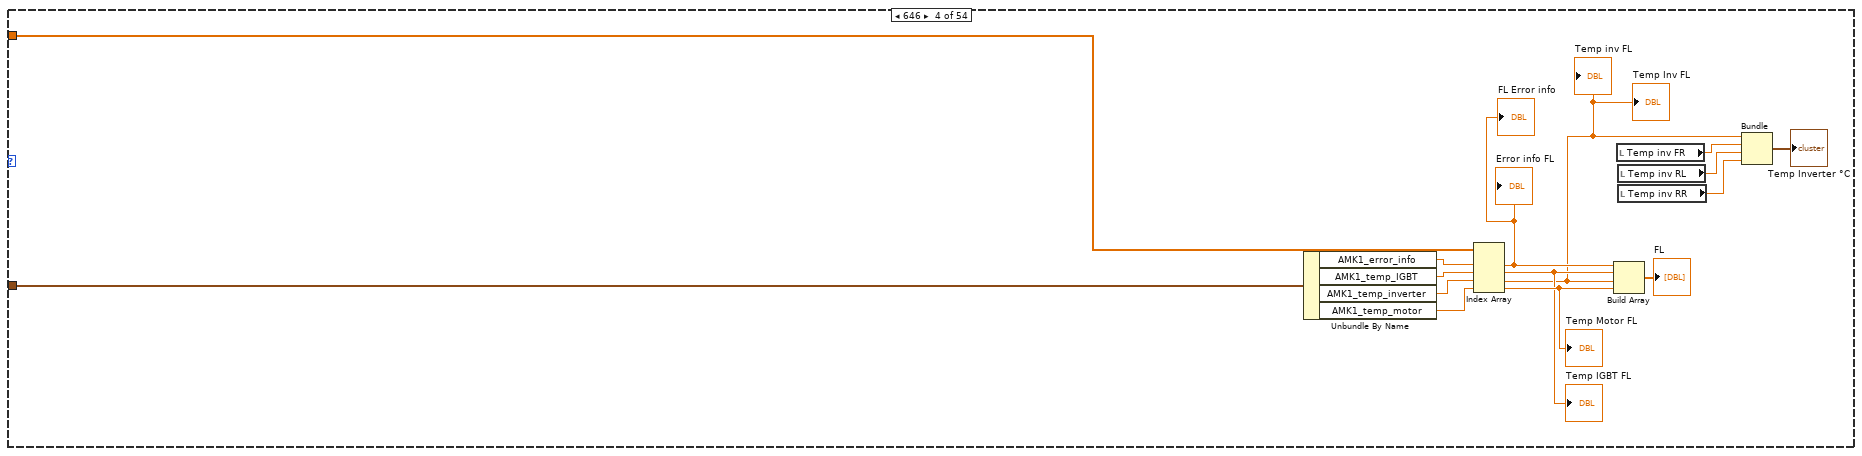
[diagram p9: hidden frame]
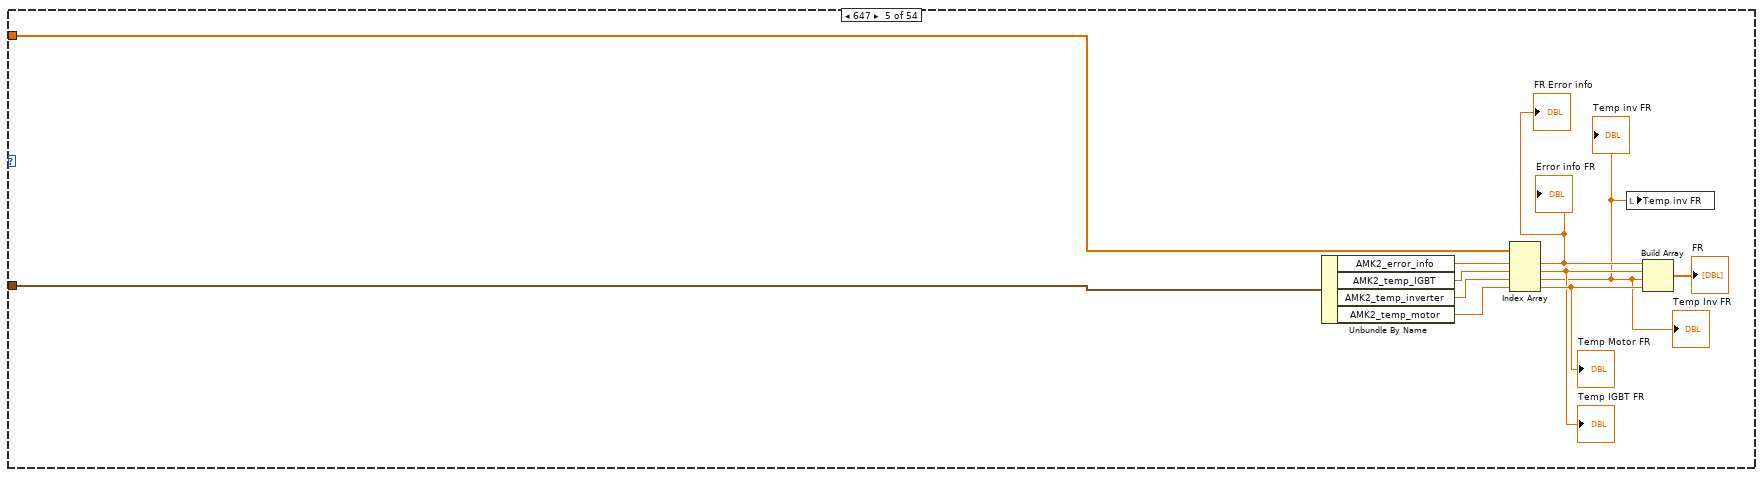
[diagram p10: hidden frame]
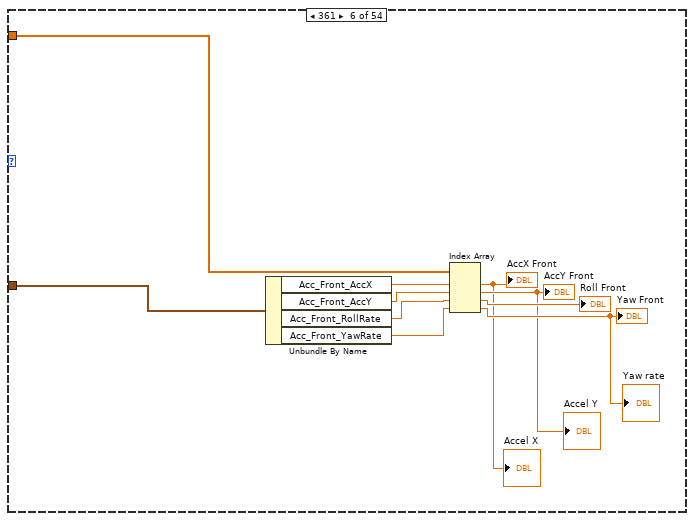
[diagram p11: hidden frame]
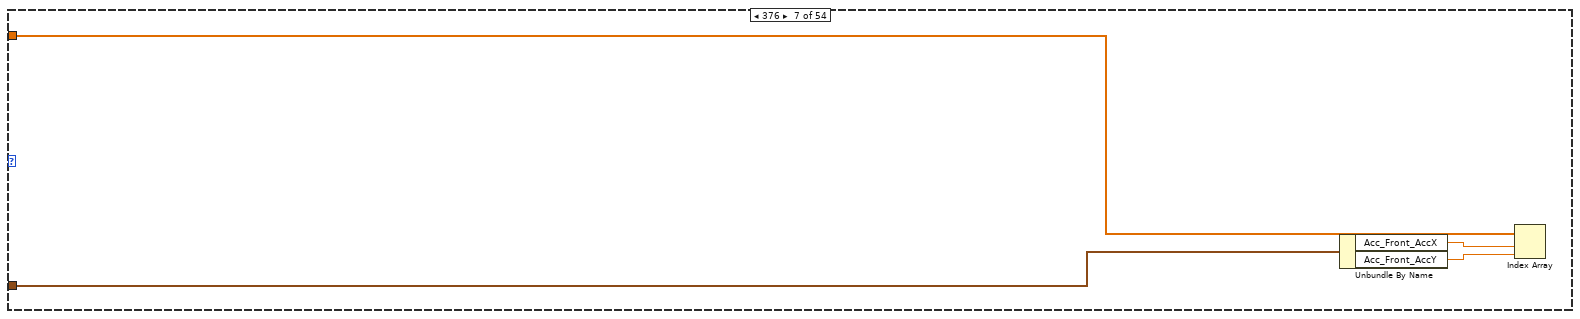
[diagram p12: hidden frame]
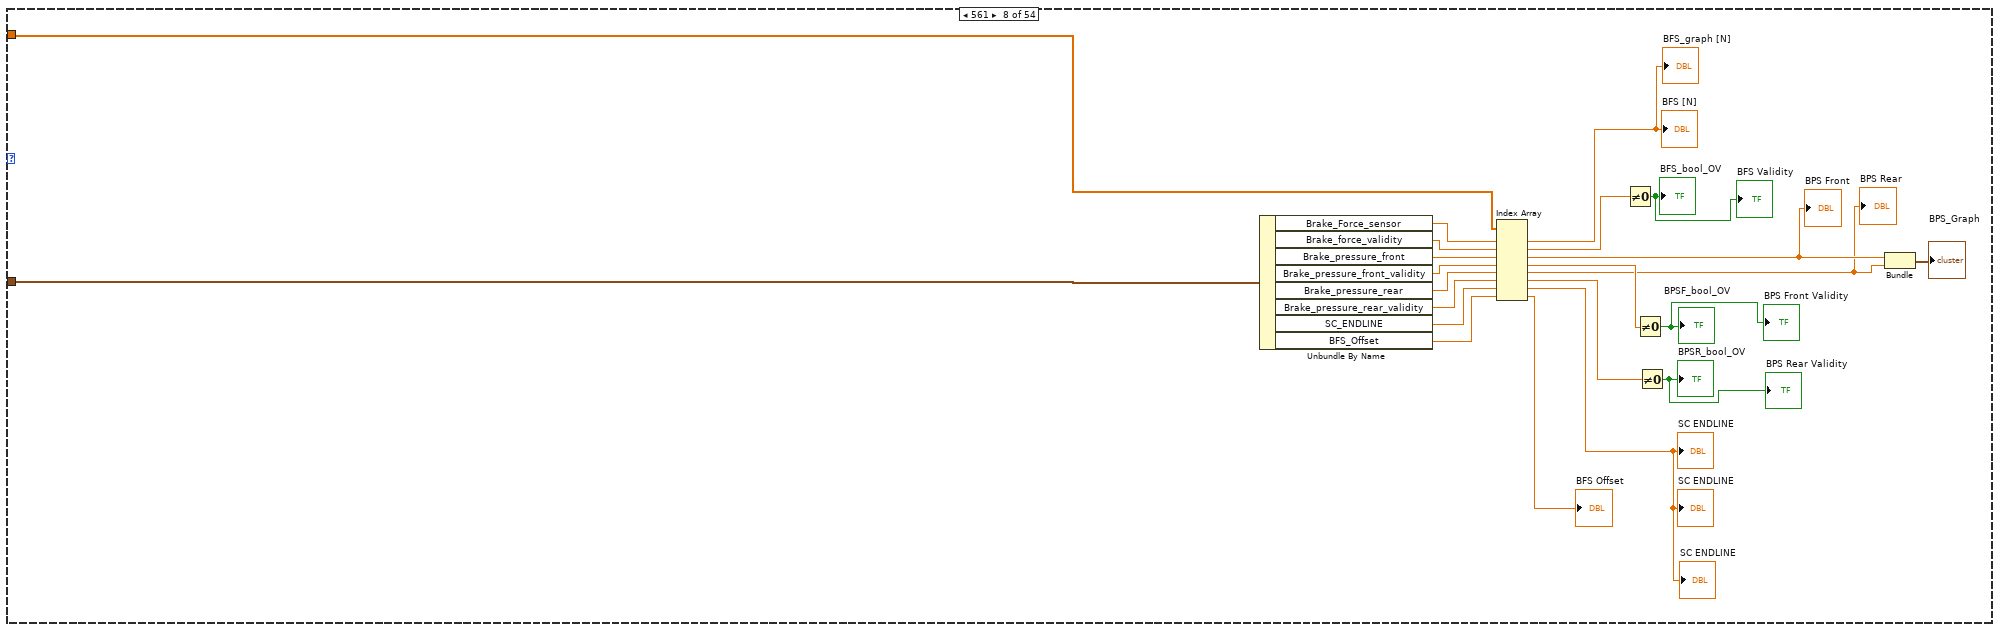
[diagram p13: hidden frame]
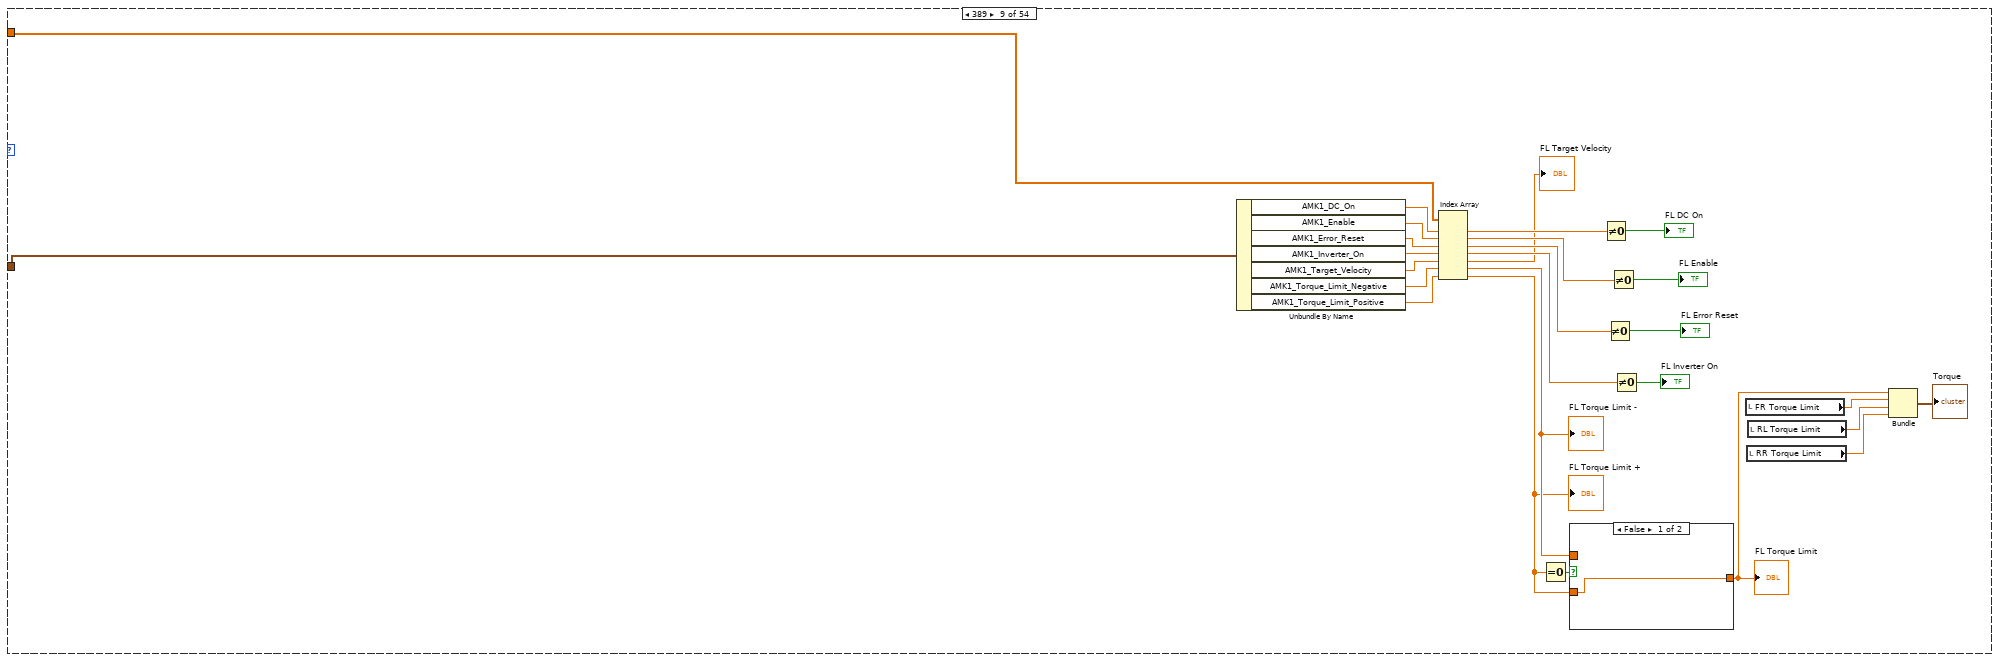
[diagram p14: hidden frame]
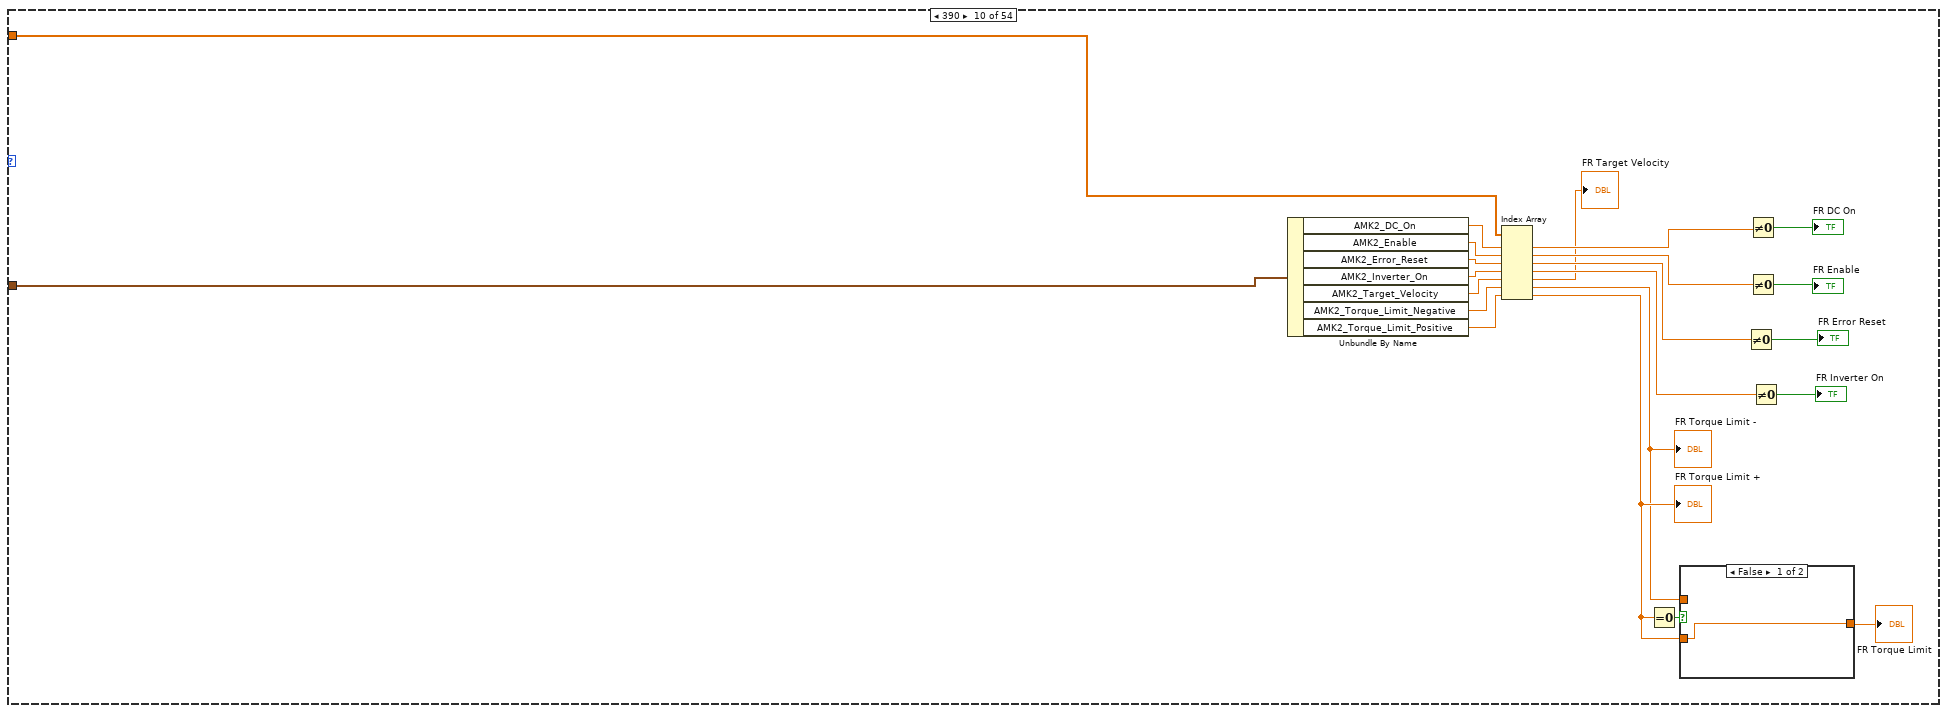
[diagram p16: hidden frame]
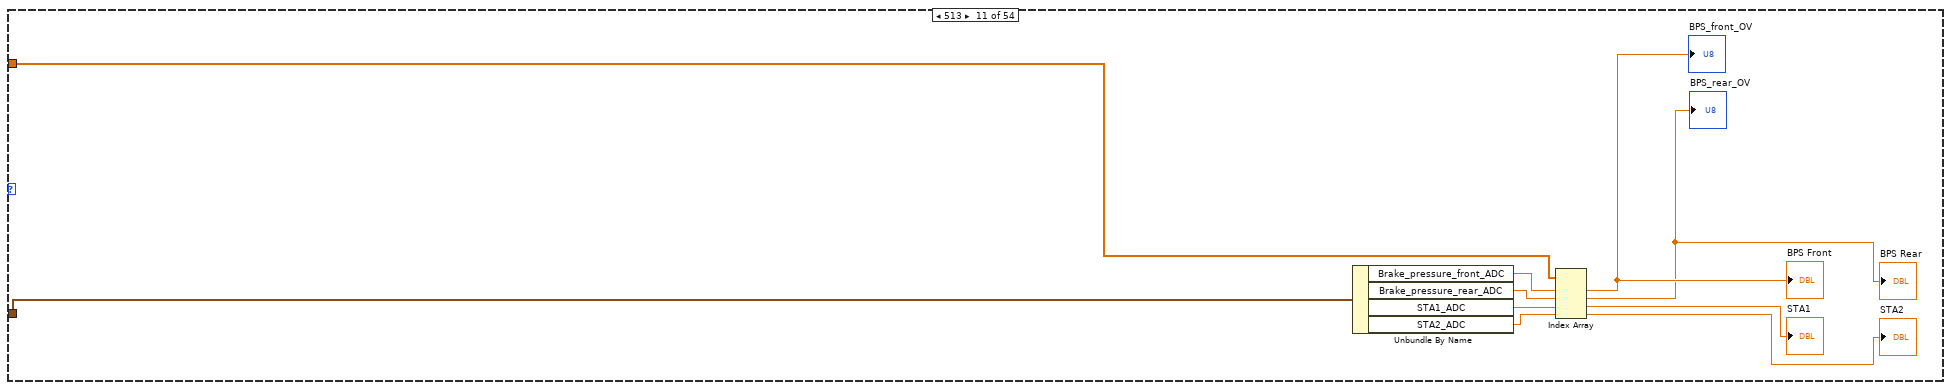
[diagram p18: hidden frame]
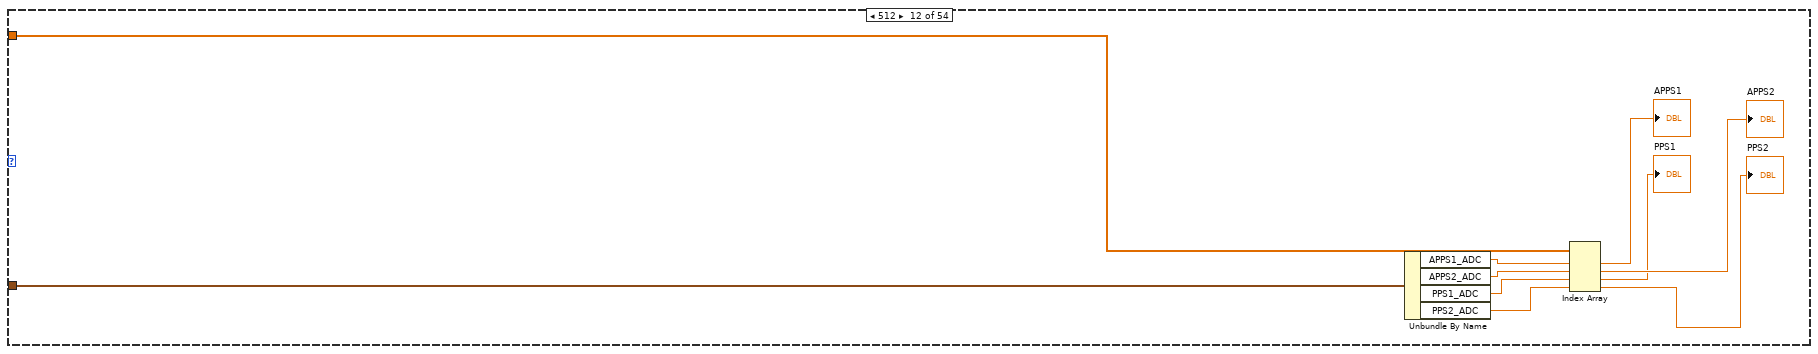
[diagram p19: hidden frame]
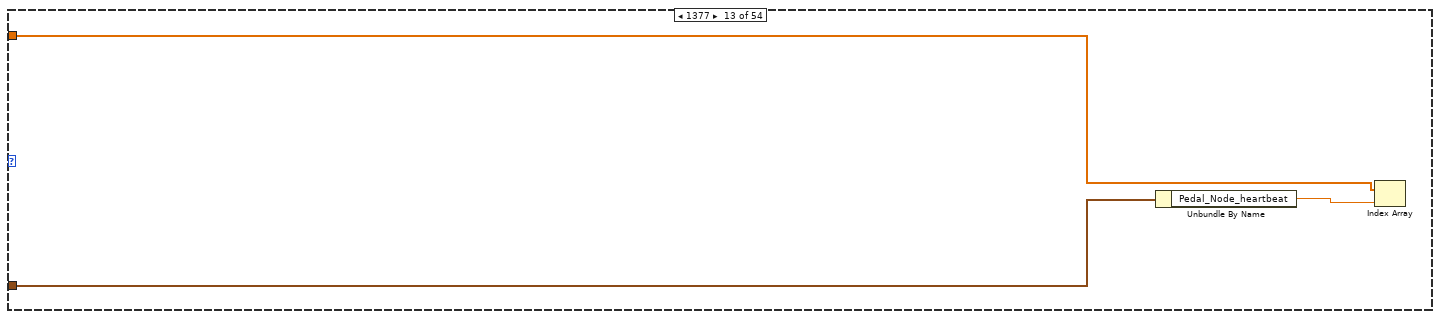
[diagram p20: hidden frame]
diagram:
  w7 = string[] ["AMK1_actual_velocity", "AMK1_magnetizing_current", "AMK1_status", "AMK1_torque_current", "AMK1_error_info", "AMK1_temp_IGBT", "AMK1_temp_inverter", "AMK1_temp_motor", "AMK2_actual_velocity", "AMK2_magnetizing_current", "AMK2_status", "AMK2_torque_current", "AMK2_error_info", "AMK2_temp_IGBT", "AMK2_temp_inverter", "AMK2_temp_motor", "ASF_X_Acceleration", "ASF_Y_Acceleration", "ASF_Yaw_rate", "Brake_Force_sensor", "Brake_force_validity", "Brake_pressure_front", "Brake_pressure_front_validity", "Brake_pressure_rear", "Brake_pressure_rear_validity", "SC_ENDLINE", "AMK1_DC_On", "AMK1_Enable", "AMK1_Error_Reset", "AMK1_Inverter_On", "AMK1_Target_Velocity", "AMK1_Torque_Limit_Negative", "AMK1_Torque_Limit_Positive", "AMK2_DC_On", "AMK2_Enable", "AMK2_Error_Reset", "AMK2_Inverter_On", "AMK2_Target_Velocity", "AMK2_Torque_Limit_Negative", "AMK2_Torque_Limit_Positive", "Brake_pressure_front_ADC", "Brake_pressure_rear_ADC", "STA1_ADC", "STA2_ADC", "APPS1_ADC", "APPS2_ADC", "PPS1_ADC", "PPS2_ADC", "Pedal_Node_heartbeat", "ASF_BFS_Vectornav_12V", "ASMS", "ASSI_state", "AS_GO_Signal", "AS_Mission_selected", "Brake_Light", "Buzzer", "CAN_Nodes_24V", "Calibration_Enabled", "Calibration_State", "Can_Nodes_Configured", "Datalogger_2D_12V", "Driving_State_Active", "EBS_FB", "EBS_IS_ACTIVE", "External_TS_Button", "Initial_Checkup_state", "MCU_EF_State", "MCU_FRONT_SUPPLY", "MCU_REAR_SUPPLY", "MCU_RF_State", "OFF_Car_State", "ON_Car_State", "PPS1", "PPS2", "Pump", "RTDS", "SB_ENGAGE", "SB_FB", "SC_Close", "SC_START", "SET_FINISH_STATE", "START_Car_State", "TCU_Power", "WATCHDOG", "Xavier_12V", "nEBS_ENGAGE", "nEBS_IS_TRIGGERED", "nEBS_SET_ACTIVE", "nSet_Driving_State", "ACCELERATION_LED", "AMS_LED", "ASB_ERROR_LED", "AUTOX_LED", "Dashboard_heartbeat_error", "EBS_TEST_LED", "HVECU_Heartbeat_error", "HV_LED", "IMD_LED", "INSPECTION_LED", "MANUAL_MODE_LED", "MCU1_LED", "MCU2_LED", "MCU3_LED", "MCU4_LED", "MCU_Heartbeat_error", "Pedal_Node_Heartbeat_error", "SC_BSPD_FB", "SC_DV_FB", "SC_DV_RELAY_FB", "SC_EBS_FB", "SC_ENDLINE_ADC", "SC_FRONT_FB", "SC_HOOP_FB", "SC_MCU_FB", "SKIDPAD_LED", "SSG_Heartbeat", "Steering_Heartbeat_error", "TCU_Heartbeat_error", "TCU_LED", "TRACKDRIVE_LED", "TS_OFF_LED", "Steering_letter1", "Steering_letter2", "Steering_letter3", "Steering_letter4", "Steering_number", "EEPROM_STA1_MAX", "EEPROM_STA1_MIN", "EEPROM_STA2_MAX", "EEPROM_STA2_MIN", "Button1", "Button2", "Button3", "Button4", "Rotary1", "Rotary2", "Rotary3", "Rotary4", "Rotary5", "Steering_heartbeat", "VDC_Brake_Force_Max", "VDC_Brake_Force_Threshold", "VDC_Drop_Parameter_New", "VDC_M_Yaw", "VDC_M_Yaw_Limit", "VDC_Powlim_Approx", "VDC_Rear_Reduction", "VDC_TC_Normalizer", "VDC_Throttle_Bias", "VDC_Yaw_Control_Balance", "VDC_Yaw_Control_Weight_Selector", "VDC_Fz_FL", "VDC_Fz_FR", "VDC_Fz_RL", "VDC_Fz_RR", "VDC_Regbrake_Front", "VDC_Regbrake_Rear", "VDC_Torque_Demand", "VDC_v_x", "EEPROM_APPS1_MAX", "EEPROM_APPS1_MIN", "EEPROM_APPS2_MAX", "EEPROM_APPS2_MIN", "APPS1_position", "APPS1_validity", "APPS2_posiition", "APPS2_validity", "APPS_plausiblity", "STA1_position", "STA1_validity", "STA2_position", "STA2_validity", "STA_plausiblity", "Xavier_AS_Finish", "Xavier_Target_Steering_Angle", "Xavier_Target_speed", "Xavier_heartbeat", "AMK3_actual_velocity", "AMK3_magnetizing_current", "AMK3_status", "AMK3_torque_current", "AMK3_error_info", "AMK3_temp_IGBT", "AMK3_temp_inverter", "AMK3_temp_motor", "AMK4_actual_velocity", "AMK4_magnetizing_current", "AMK4_status", "AMK4_torque_current", "AMK4_error_info", "AMK4_temp_IGBT", "AMK4_temp_inverter", "AMK4_temp_motor", "Button_OFF", "Button_ON", "Button_START", "Dash_BLANK", "Dash_MODE", "Dash_XLAT", "Dashboard_ID", "Dashboarrd_heartbeat", "AIR_minus_state", "AIR_plus_State", "AMS_Relay_State", "AMS_Status", "Driver_Protection_State", "Error_STAMP_TSAL", "Error_value", "HV_Acc_Menu", "HV_Cell_OT", "HV_Cell_OV", "HV_Cell_UV", "HV_DetStatus", "HV_ECU_Heartbeat", "HV_ECU_SC_Endline_State", "IMD_Relay_State", "IMD_Status", "MCU_STAMP", "PC_Error", "PC_State", "Place_of_error", "TSAL_GREEN", "TSAL_RED", "TS_Over_Voltage", "TS_Overcurrent", "HV_Current", "HV_Voltage_After_AIRs", "HV_Voltage_Before_AIRs", "State_of_Charge", "HV_Cell_ID", "HV_Cell_Temperature", "HV_Cell_Voltage", "Critical_cell_values_heartbeat", "HV_Cell_Temp_MAX", "HV_Cell_Voltage_MIN", "AMK3_Control", "AMK3_Target_Velocity", "AMK3_TorqueLimitNegative", "AMK3_TorqueLimitPositive", "AMK4_Control", "AMK4_Target_Velocity", "AMK4_TorqueLimitNegative", "AMK4_TorqueLimitPositive", "RES_GO_Signal"]  # For log compatibility check(const of signal names)
  # "0 - UDP\n1 - XNET\n2 - CAN\n3 - Replay"
  n1 = call "conversion_init.vi"() -> ("Signal list"=w8:refnum<k21>[], "CAN2 conversion session"=w12:T9, "CAN1 conversion session"=w11:T9)
  n2 = call <vilib>:"Intialize Keyboard.vi"() -> ("error out"=w19:errorcluster, "device ID"=w20:refnum<k1>)  [unwired: 10 in]
  n3 = property class="TabCtl (strict)"() -> ("Value"=w18:T2)  [unwired: 2 in, 2 out]
  n4 = while {
    tunnel: w8 -> [w25]
    tunnel: [w21] -> w10
    i -> [w24]
    stop <- w21 stop-if-true
    n5 = for {
      tunnel: [w28] -> w22 mode=indexing
      tunnel: w25 -> [w27] mode=indexing
      n6 = property class="XNET Signal"(reference=w27) -> ("NameShort"=w28:string)  [unwired: 1 in, 2 out]
    }
    "signal names" <- w22
    n7 = property on="Signal indexes" class="Clust (strict)"() -> ("Controls[]"=w26:refnum<vi>[])  [unwired: 2 in, 2 out]
    n8 = Greater?(x=w24, y=0) -> (0:w21:bool)
    n9 = for {
      tunnel: w26 -> [w33] mode=indexing
      tunnel: w22 -> [w32]
      n10 = property class="Ctl"(reference=w33) -> (reference out=w30:refnum<vi>, "Label.Text"=w31:string)  [unwired: 1 in, 1 out]
      n11 = Search 1D Array(1D array=w32, element=w31) -> (index of element=w29:i32)  [unwired: 1 in]
      n12 = property class="Ctl"(reference=w30, "Value"=w29) -> ()  [unwired: 1 in, 2 out]
    }
  }
  n13 = case shown="1" "Data source" {
    tunnel: [_ _ w41 _] -> w15
    tunnel: [_ w39 _ _] -> w14
    tunnel: [TRUE TRUE TRUE _] -> w13
    tunnel: w7 -> [_ _ _ _]
    frame 0, Default {
    }
    frame 1 {
      n14 = call "xnet_init.vi"() -> ("Intf2"=→"Intf2":refnum<k21>, "XNET Init"=w39:T10, "Active intfs"=→"Active intfs":i32, "Intf1"=→"Intf1":refnum<k21>)  [unwired: 5 in]
    }
    frame 2 {
      n15 = call "nican_init.vi"() -> ("CAN Init"=w41:T12)  [unwired: 2 in]
    }
    frame 3 {
      # "Tax: elsõ sorban beolvassa a log timestepet, ezzel felülírja a vi timestepjét, utólag vmi modifierrel lehet szabályozni, második sorban beolvassa a log signal listjét és összematcheli a mostanival, ha nem matchel, akkor felülírja a startot"
    }
  }
  n16 = while {
    tunnel: w20 -> [w49]
    tunnel: w19 -> [w48]
    tunnel: w18 -> [w42]
    stop <- FALSE stop-if-true
    n17 = call "keynav_controller.vi"("Error in"=w48, "Reset Keyboard"="Reset Keyboard", "Keyboard id"=w49) -> ("Key"=w43:T3, "Enable"=w46:bool, "Keynav error"=→"Key Navigation error":errorcluster)
    "Key" <- w43
    n18 = Wait Until Next ms Multiple(millisecond multiple=u32 15) -> ()  [unwired: 1 out]
    n19 = case shown="True" w46 {
      tunnel: w43 -> [_ w52]
      tunnel: w42 -> [_ w51]
      frame False {
      }
      frame True {
        n20 = call "keynav_keybinds.vi"("Tab at start"=w51, "Key"=w52) -> ()  [unwired: 1 out]
      }
    }
  }
  n21 = property class="TabCtl (strict)"("FG Color"=u32 12369084 ("Tab Color")) -> ()  [unwired: 2 in, 2 out]
  n22 = UDP Open(11:"Port") -> (port=w5:refnum<k16>, 0:w4:errorcluster)  [unwired: 4 in, 1 out]
  n23 = while {
    tunnel: w5 -> [w80]
    tunnel: "Data source" -> [w79]
    tunnel: T7 {"timestamp"=timestamp(0 s since 1904-01-01), "payload"=[0, 0, 0, 0, 0, 0, 0, 0], "identifier"=0, "type"=0, "extended?"=FALSE, "echo?"=FALSE} ("CAN frame") -> [w78]
    tunnel: "Main timestep" -> [w77]
    tunnel: w15 -> [w63]
    tunnel: w14 -> [w62]
    tunnel: w13 -> [w58]
    tunnel: w12 -> [w61]
    tunnel: w11 -> [w60]
    tunnel: w10 -> [w56]
    tunnel: w4 -> [w54]
    stop <- FALSE stop-if-true
    n24 = Wait Until Next ms Multiple(millisecond multiple=w77) -> ()  [unwired: 1 out]
    n25 = And(x=w58, y=w56) -> (x .and. y?=w57:bool)
    n26 = And(x="Start Telemetry", y=w57) -> (x .and. y?=w64:bool)
    "Is running" <- w64
    n27 = flat-sequence {
      tunnel: w64 -> [w88]
      tunnel: w78 -> [w89]
      tunnel: w79 -> [w90]
      tunnel: w80 -> [w91]
      tunnel: [w91] -> w75
      tunnel: [w90] -> w74
      tunnel: [w89] -> w73
      tunnel: [w88] -> w72
      tunnel: [w87] -> w71
      tunnel: w63 -> [w86]
      tunnel: [w86] -> w69
      tunnel: [w85] -> w68
      tunnel: w62 -> [w85]
      tunnel: [w84] -> w67
      tunnel: w61 -> [w84]
      tunnel: [w83] -> w66
      tunnel: w60 -> [w83]
      tunnel: [w82] -> w65
      tunnel: "Signal indexes" -> [w82]
      tunnel: w54 -> [w81]
      tunnel: [w81] -> w53
      tunnel: w75 -> [w102]
      tunnel: w74 -> [w101]
      tunnel: w73 -> [w100]
      tunnel: w72 -> [w99]
      tunnel: w71 -> [w98]
      tunnel: [w98] -> w70
      tunnel: w69 -> [w97]
      tunnel: w68 -> [w96]
      tunnel: w67 -> [w94]
      tunnel: w66 -> [w95]
      tunnel: w65 -> [w93]
      tunnel: w53 -> [w92]
      tunnel: w70 -> [w1673]
      frame #0 {
        n28 = Tick Count (ms)() -> (millisecond timer value=w87:u32)
      }
      frame #1 {
        n29 = case shown="True" w99 {
          tunnel: w102 -> [_ w117]
          tunnel: w101 -> [_ w108]
          tunnel: w100 -> [_ w116]
          tunnel: w97 -> [_ w115]
          tunnel: w96 -> [_ w114]
          tunnel: w95 -> [_ w111]
          tunnel: w94 -> [_ w110]
          tunnel: w93 -> [_ w113]
          tunnel: w92 -> [_ w106]
          frame False {
          }
          frame True {
            # "TODO"
            n30 = case shown="4" w108 {
              tunnel: w117 -> [w1639 _ _ _ _]
              tunnel: w116 -> [w1640 _ w1659 w1667 w1670]
              tunnel: [w1642 w1648 w1658 w1668 w1671] -> w112
              tunnel: w115 -> [_ _ w1664 _ _]
              tunnel: w114 -> [_ w1653 _ _ _]
              tunnel: w106 -> [w1638 _ _ _ _]
              frame 0, Default {
                n31 = call "ReadUDP.vi"("error in (no error)"=w1638, "connection ID"=w1639, "Message length"=u16 10) -> ("error out"=→"UDP Read error":errorcluster, "Discarding"=w1634:bool, "Array"=w1641:u8[][])
                "Discarding" <- w1634
                n32 = call "bytearray2frame.vi"("CAN template"=w1640, "2D Array"=w1641) -> ("CAN frame array"=w1642:T7[])
                n33 = feedback #1(0) -> (w1636:i32)
                n34 = case shown="True" w1634 {
                  tunnel: w1636 -> [w1645 w1647]
                  tunnel: [w1645 w1646] -> w1635
                  frame False {
                  }
                  frame True {
                    n35 = Increment(x=w1647) -> (x+1=w1646:i32)
                  }
                }
                "Discard count" <- w1635
                n36 = feedback-in #1(w1635) -> ()
              }
              frame 1 {
                n37 = Unbundle(w1653) -> ("XNET session A"=w1652:refnum<k21>, "Error out A"=w1651:errorcluster, "XNET session B"=w1650:refnum<k21>, "Error out B"=w1649:errorcluster)
                n38 = call-poly <vilib>:"XNET Read.vi"("session in"=w1650, "error in (no error)"=w1649) -> ("data"=w1655:T7[], "error out"=w1656:errorcluster)  [unwired: 10 in, 2 out]
                "XNET error (Intf 2)" <- w1656
                n39 = call-poly <vilib>:"XNET Read.vi"("session in"=w1652, "error in (no error)"=w1651) -> ("data"=w1654:T7[], "error out"=w1657:errorcluster)  [unwired: 10 in, 2 out]
                "XNET error (Intf 1)" <- w1657
                n40 = call <vilib>:"Clear Errors.vi"("error in (no error)"=w1656) -> ()  [unwired: 5 in, 2 out]
                n41 = Build Array (concatenate)(w1654, w1655) -> (w1648:T7[])
                n42 = call <vilib>:"Clear Errors.vi"("error in (no error)"=w1657) -> ()  [unwired: 5 in, 2 out]
              }
              frame 2 {
                n43 = Unbundle(w1664) -> ("ObjHandle A"=w1663:T11, "Error out A"=w1662:errorcluster, "ObjHandle B"=w1661:T11, "Error out B"=w1660:errorcluster)
                n44 = call "nican_loop.vi"("ObjHandle A"=w1663, "Error in A"=w1662, "ObjHandle B"=w1661, "CAN template"=w1659, "Error in B"=w1660) -> ("Error out A"=w1666:errorcluster, "Frames read"=w1658:T7[], "Error out B"=w1665:errorcluster)  [unwired: 1 in]
                "NI-CAN0 error" <- w1666
                "NI-CAN1 error" <- w1665
                n45 = call <vilib>:"Clear Errors.vi"("error in (no error)"=w1665) -> ()  [unwired: 5 in, 2 out]
                n46 = call <vilib>:"Clear Errors.vi"("error in (no error)"=w1666) -> ()  [unwired: 5 in, 2 out]
              }
              frame 3 {
                # "Tax: Timestepenként a frames to update és a signal data elmentõdik, ezeket kell visszaolvasni és felülírni"
                n47 = Build Array(w1667) -> (w1668:T7[])
              }
              frame 4 {
                n48 = local read "serial in 2"() -> (w1669:u8[][])
                n49 = call "bytearray2frame.vi"("CAN template"=w1670, "2D Array"=w1669) -> ("CAN frame array"=w1671:T7[])
              }
            }
            n50 = Equal?(x=u16 3, y=w108) -> (x = y?=w103:bool)
            n51 = for {
              tunnel: w112 -> [w1633] mode=indexing
              tunnel: [w1632] -> w105 mode=indexing
              workers-P: _ -> [_]
              n52 = Unbundle By Name(w1633) -> ("identifier"=w1632:u32)
            }
            n53 = Array Size(array=w105) -> (size(s)=→"Frames read":i32)
            n54 = case shown="False" w103 {
              tunnel: w105 -> [w118 _]
              tunnel: [w118 _] -> w109
              frame False {
              }
              frame True {
              }
            }
            n55 = for {
              tunnel: w109 -> [w131] mode=indexing
              tunnel: w113 -> [w130]
              tunnel: w112 -> [w127] mode=indexing
              tunnel: w111 -> [w125]
              tunnel: w110 -> [w122]
              tunnel: w103 -> [w119]
              # "TODO"
              n56 = Build Array(w127) -> (w126:T7[])
              n57 = call "conversion_loop.vi"("CAN frame array"=w126, "CAN1 conversion session"=w125, "CAN2 conversion session"=w122) -> ("CAN1 signal data"=w129:dbl[], "CAN2 signal data"=w128:dbl[], "CAN1 error out"=w124:errorcluster, "CAN2 error out"=w123:errorcluster)  [unwired: 2 in]
              "CAN1 Frame to signal" <- w124
              "CAN2 Frame to signal" <- w123
              n58 = call <vilib>:"Clear Errors.vi"("error in (no error)"=w123) -> ()  [unwired: 5 in, 2 out]
              n59 = call <vilib>:"Clear Errors.vi"("error in (no error)"=w124) -> ()  [unwired: 5 in, 2 out]
              n60 = Build Array (concatenate)(w129, w128) -> (w120:dbl[])
              n61 = case shown="False" w119 {
                tunnel: [w132 _] -> w121
                tunnel: w120 -> [w132 _]
                frame False {
                }
                frame True {
                }
              }
              n62 = case shown="417" w131 {
                tunnel: w121 -> [_ w146 w158 w169 w180 w192 w196 w212 w238 w262 w278 w288 w294 w377 w462 w523 w534 w563 w580 w597 w637 w651 w665 w675 w702 w850 w857 w893 w920 w952 w970 w1022 w1135 w1143 w1154 w1165 w1176 w1198 w1238 w1269 w1370 w1381 w1402 w1426 w1435 w1446 w1449 w1462 w1475 w1511 w1573 w1604 w1620 w1630]
                tunnel: w130 -> [_ w147 w153 w168 w179 w193 w195 w213 w239 w263 w277 w287 w293 w354 w461 w522 w533 w552 w579 w598 w636 w652 w666 w674 w703 w851 w856 w892 w919 w953 w971 w1023 w1136 w1142 w1153 w1164 w1175 w1197 w1237 w1268 w1369 w1380 w1401 w1425 w1436 w1447 w1451 w1468 w1483 w1533 w1574 w1611 w1627 w1631]
                frame 0, Default {
                }
                frame 644 {
                  n63 = Unbundle By Name(w147) -> ("AMK1_actual_velocity"=w145:dbl, "AMK1_magnetizing_current"=w144:dbl, "AMK1_status"=w143:dbl, "AMK1_torque_current"=w142:dbl)
                  n64 = Index Array(array=w146, index #1=w145, index #2=w144, index #3=w143, index #4=w142) -> (element #1=w135:dbl, element #2=→"Im FL":dbl, element #3=w134:dbl, element #4=→"It FL":dbl)
                  "Actual_vel_FL_OV" <- w135
                  n65 = local read "Actual_vel_FR_OV"() -> (w136:dbl)
                  n66 = local read "Actual_vel_RL_OV"() -> (w137:dbl)
                  n67 = local read "Actual_vel_RR_OV"() -> (w138:dbl)
                  n68 = Number To Boolean Array(number=w134) -> (Boolean array=→"FL Status":bool[])
                  n69 = Bundle("Data"=w135, "Actual_vel_FR_OV"=w136, "Actual_vel_RL_OV"=w137, "Actual_vel_RR_OV"=w138) -> (→"MCU Actual Velocity 1/min":T5)  [unwired: 1 in]
                }
                frame 645 {
                  n70 = Unbundle By Name(w153) -> ("AMK2_actual_velocity"=w157:dbl, "AMK2_magnetizing_current"=w156:dbl, "AMK2_status"=w155:dbl, "AMK2_torque_current"=w154:dbl)
                  n71 = Index Array(array=w158, index #1=w157, index #2=w156, index #3=w155, index #4=w154) -> (element #1=→"Actual_vel_FR_OV":dbl, element #2=→"Im FR":dbl, element #3=w148:dbl, element #4=→"It FR":dbl)
                  n72 = Number To Boolean Array(number=w148) -> (Boolean array=→"FR Status":bool[])
                }
                frame 646 {
                  n73 = Unbundle By Name(w168) -> ("AMK1_error_info"=w173:dbl, "AMK1_temp_IGBT"=w172:dbl, "AMK1_temp_inverter"=w171:dbl, "AMK1_temp_motor"=w170:dbl)
                  n74 = Index Array(array=w169, index #1=w173, index #2=w172, index #3=w171, index #4=w170) -> (element #1=w160:dbl, element #2=w165:dbl, element #3=w159:dbl, element #4=w166:dbl)
                  "Error info FL" <- w160
                  "Temp IGBT FL" <- w165
                  "Temp Motor FL" <- w166
                  "FL Error info" <- w160
                  "Temp inv FL" <- w159
                  "Temp Inv FL" <- w159
                  n75 = Build Array(w160, w165, w159, w166) -> (→"FL":dbl[])
                  n76 = local read "Temp inv FR"() -> (w163:dbl)
                  n77 = local read "Temp inv RL"() -> (w162:dbl)
                  n78 = local read "Temp inv RR"() -> (w161:dbl)
                  n79 = Bundle("Data"=w159, "Temp inv FR"=w163, "Temp inv RL"=w162, "Temp inv RR"=w161) -> (→"Temp Inverter °C":T13)  [unwired: 1 in]
                }
                frame 647 {
                  n80 = Unbundle By Name(w179) -> ("AMK2_error_info"=w184:dbl, "AMK2_temp_IGBT"=w183:dbl, "AMK2_temp_inverter"=w182:dbl, "AMK2_temp_motor"=w181:dbl)
                  n81 = Index Array(array=w180, index #1=w184, index #2=w183, index #3=w182, index #4=w181) -> (element #1=w175:dbl, element #2=w176:dbl, element #3=w174:dbl, element #4=w177:dbl)
                  "Error info FR" <- w175
                  "Temp IGBT FR" <- w176
                  "Temp Motor FR" <- w177
                  "Temp inv FR" <- w174
                  "FR Error info" <- w175
                  "Temp Inv FR" <- w174
                  n82 = local write "Temp inv FR"(w174) -> ()
                  n83 = Build Array(w175, w176, w174, w177) -> (→"FR":dbl[])
                }
                frame 361 {
                  n84 = Unbundle By Name(w193) -> ("Acc_Front_AccX"=w194:dbl, "Acc_Front_AccY"=w191:dbl, "Acc_Front_RollRate"=w190:dbl, "Acc_Front_YawRate"=w189:dbl)
                  n85 = Index Array(array=w192, index #1=w194, index #2=w191, index #3=w190, index #4=w189) -> (element #1=→"AccX Front" →"Accel X":dbl, element #2=→"AccY Front" →"Accel Y":dbl, element #3=→"Roll Front":dbl, element #4=→"Yaw Front" →"Yaw rate":dbl)
                }
                frame 376 {
                  n86 = Unbundle By Name(w195) -> ("Acc_Front_AccX"=w198:dbl, "Acc_Front_AccY"=w197:dbl)
                  n87 = Index Array(array=w196, index #1=w198, index #2=w197) -> ()  [unwired: 2 out]
                }
                frame 561 {
                  n88 = Unbundle By Name(w213) -> ("Brake_Force_sensor"=w220:dbl, "Brake_force_validity"=w219:dbl, "Brake_pressure_front"=w218:dbl, "Brake_pressure_front_validity"=w217:dbl, "Brake_pressure_rear"=w216:dbl, "Brake_pressure_rear_validity"=w215:dbl, "SC_ENDLINE"=w214:dbl, "BFS_Offset"=w200:dbl)
                  n89 = Index Array(array=w212, index #1=w220, index #2=w219, index #3=w218, index #4=w217, index #5=w216, index #6=w215, index #7=w214, index #8=w200) -> (element #1=→"BFS [N]" →"BFS_graph [N]":dbl, element #2=w209:dbl, element #3=w202:dbl, element #4=w210:dbl, element #5=w201:dbl, element #6=w211:dbl, element #7=→"SC ENDLINE" →"SC ENDLINE" →"SC ENDLINE":dbl, element #8=→"BFS Offset":dbl)
                  "BPS Rear" <- w201
                  "BPS Front" <- w202
                  n90 = Not Equal To 0?(x=w209) -> (x != 0?=→"BFS_bool_OV" →"BFS Validity":bool)
                  n91 = Not Equal To 0?(x=w210) -> (x != 0?=→"BPSF_bool_OV" →"BPS Front Validity":bool)
                  n92 = Not Equal To 0?(x=w211) -> (x != 0?=→"BPSR_bool_OV" →"BPS Rear Validity":bool)
                  n93 = Bundle("Data"=w202, "Data"=w201) -> (→"BPS_Graph":cluster{"Data":dbl, "Data":dbl})  [unwired: 1 in]
                }
                frame 389 {
                  n94 = Unbundle By Name(w239) -> ("AMK1_DC_On"=w246:dbl, "AMK1_Enable"=w245:dbl, "AMK1_Error_Reset"=w244:dbl, "AMK1_Inverter_On"=w243:dbl, "AMK1_Target_Velocity"=w242:dbl, "AMK1_Torque_Limit_Negative"=w240:dbl, "AMK1_Torque_Limit_Positive"=w241:dbl)
                  n95 = Index Array(array=w238, index #1=w246, index #2=w245, index #3=w244, index #4=w243, index #5=w242, index #6=w240, index #7=w241) -> (element #1=w237:dbl, element #2=w235:dbl, element #3=w234:dbl, element #4=w233:dbl, element #5=→"FL Target Velocity":dbl, element #6=w227:dbl, element #7=w226:dbl)
                  "FL Torque Limit +" <- w226
                  "FL Torque Limit -" <- w227
                  n96 = Equal To 0?(x=w226) -> (x = 0?=w228:bool)
                  n97 = case shown="False" w228 {
                    tunnel: w227 -> [_ w248]
                    tunnel: [w247 w248] -> w221
                    tunnel: w226 -> [w247 _]
                    frame False {
                    }
                    frame True {
                    }
                  }
                  "FL Torque Limit" <- w221
                  n98 = Not Equal To 0?(x=w237) -> (x != 0?=→"FL DC On":bool)
                  n99 = Not Equal To 0?(x=w234) -> (x != 0?=→"FL Error Reset":bool)
                  n100 = Not Equal To 0?(x=w235) -> (x != 0?=→"FL Enable":bool)
                  n101 = Not Equal To 0?(x=w233) -> (x != 0?=→"FL Inverter On":bool)
                  n102 = local read "FR Torque Limit"() -> (w222:dbl)
                  n103 = local read "RR Torque Limit"() -> (w224:dbl)
                  n104 = local read "RL Torque Limit"() -> (w225:dbl)
                  n105 = Bundle("Data"=w221, "FR Torque Limit"=w222, "RL Torque Limit"=w225, "RR Torque Limit"=w224) -> (→"Torque":T14)  [unwired: 1 in]
                }
                frame 390 {
                  n106 = Unbundle By Name(w263) -> ("AMK2_DC_On"=w270:dbl, "AMK2_Enable"=w269:dbl, "AMK2_Error_Reset"=w268:dbl, "AMK2_Inverter_On"=w267:dbl, "AMK2_Target_Velocity"=w266:dbl, "AMK2_Torque_Limit_Negative"=w265:dbl, "AMK2_Torque_Limit_Positive"=w264:dbl)
                  n107 = Index Array(array=w262, index #1=w270, index #2=w269, index #3=w268, index #4=w267, index #5=w266, index #6=w265, index #7=w264) -> (element #1=w254:dbl, element #2=w255:dbl, element #3=w256:dbl, element #4=w257:dbl, element #5=→"FR Target Velocity":dbl, element #6=w250:dbl, element #7=w251:dbl)
                  "FR Torque Limit +" <- w251
                  "FR Torque Limit -" <- w250
                  n108 = Equal To 0?(x=w251) -> (x = 0?=w252:bool)
                  n109 = case shown="False" w252 {
                    tunnel: w250 -> [_ w272]
                    tunnel: [w271 w272] -> w249
                    tunnel: w251 -> [w271 _]
                    frame False {
                    }
                    frame True {
                    }
                  }
                  "FR Torque Limit" <- w249
                  n110 = Not Equal To 0?(x=w256) -> (x != 0?=→"FR Error Reset":bool)
                  n111 = Not Equal To 0?(x=w254) -> (x != 0?=→"FR DC On":bool)
                  n112 = Not Equal To 0?(x=w255) -> (x != 0?=→"FR Enable":bool)
                  n113 = Not Equal To 0?(x=w257) -> (x != 0?=→"FR Inverter On":bool)
                }
                frame 513 {
                  n114 = Unbundle By Name(w277) -> ("Brake_pressure_front_ADC"=w282:dbl, "Brake_pressure_rear_ADC"=w281:dbl, "STA1_ADC"=w280:dbl, "STA2_ADC"=w279:dbl)
                  n115 = Index Array(array=w278, index #1=w282, index #2=w281, index #3=w280, index #4=w279) -> (element #1=→"BPS_front_OV" →"BPS Front":dbl, element #2=→"BPS_rear_OV" →"BPS Rear":dbl, element #3=→"STA1":dbl, element #4=→"STA2":dbl)
                }
                frame 512 {
                  n116 = Unbundle By Name(w287) -> ("APPS1_ADC"=w292:dbl, "APPS2_ADC"=w291:dbl, "PPS1_ADC"=w290:dbl, "PPS2_ADC"=w289:dbl)
                  n117 = Index Array(array=w288, index #1=w292, index #2=w291, index #3=w290, index #4=w289) -> (element #1=→"APPS1":dbl, element #2=→"APPS2":dbl, element #3=→"PPS1":dbl, element #4=→"PPS2":dbl)
                }
                frame 1377 {
                  n118 = Unbundle By Name(w293) -> ("Pedal_Node_heartbeat"=w295:dbl)
                  n119 = Index Array(array=w294, index=w295) -> ()  [unwired: 1 out]
                }
                frame 819 {
                  n120 = Unbundle By Name(w354) -> ("ASF_BFS_Vectornav_12V"=w393:dbl, "ASMS"=w392:dbl, "ASSI_state"=w391:dbl, "AS_GO_Signal"=w390:dbl, "AS_Mission_selected"=w389:dbl, "Brake_Light"=w388:dbl, "Buzzer"=w387:dbl, "CAN_Nodes_24V"=w386:dbl, "Calibration_Enabled"=w385:dbl, "Calibration_State"=w384:dbl, "Can_Nodes_Configured"=w383:dbl, "Datalogger_2D_12V"=w382:dbl, "Driving_State_Active"=w381:dbl, "EBS_FB"=w380:dbl, "DV_SDC_READY"=w379:dbl, "External_TS_Button"=w378:dbl, "Initial_Checkup_state"=w300:dbl, "MCU_EF_State"=w376:dbl, "MCU_FRONT_SUPPLY"=w375:dbl, "MCU_REAR_SUPPLY"=w374:dbl, "MCU_RF_State"=w373:dbl, "OFF_Car_State"=w372:dbl, "ON_Car_State"=w371:dbl, "PPS1"=w370:dbl, "PPS2"=w369:dbl, "Pump"=w368:dbl, "RTDS_Car_state"=w309:dbl, "nSB_ENGAGE"=w367:dbl, "SB_FB"=w366:dbl, "SC_Close"=w365:dbl, "SC_START"=w364:dbl, "TS_ACTIVATION_BUTTON_COCKPIT"=w363:dbl, "START_Car_State"=w362:dbl, "TCU_Power"=w361:dbl, "WATCHDOG"=w360:dbl, "Xavier_12V"=w359:dbl, "nEBS_ENGAGE"=w358:dbl, "DV_SDC_CLOSE"=w357:dbl, "nEBS_SET_ACTIVE"=w356:dbl, "AS_DRIVING_MODE"=w355:dbl, "AS_State"=w353:dbl, "Dashboard_heartbeat_error"=w335:dbl, "HVECU_Heartbeat_error"=w334:dbl, "MCU_Heartbeat_error"=w333:dbl, "Pedal_Node_Heartbeat_error"=w332:dbl, "Steering_Heartbeat_error"=w331:dbl, "TCU_Heartbeat_error"=w330:dbl, "BAG_START"=w298:dbl)
                  n121 = Index Array(array=w377, index #1=w393, index #2=w392, index #3=w391, index #4=w390, index #5=w389, index #6=w388, index #7=w387, index #8=w386, index #9=w385, index #10=w384, index #11=w383, index #12=w382, index #13=w381, index #14=w380, index #15=w379, index #16=w378, index #17=w300, index #18=w376, index #19=w375, index #20=w374, index #21=w373, index #22=w372, index #23=w371, index #24=w370, index #25=w369, index #26=w368, index #27=w309, index #28=w367, index #29=w366, index #30=w365, index #31=w364, index #32=w363, index #33=w362, index #34=w361, index #35=w360, index #36=w359, index #37=w358, index #38=w357, index #39=w356, index #40=w355, index #41=w353, index #42=w335, index #43=w334, index #44=w333, index #45=w332, index #46=w331, index #47=w330, index #48=w298) -> (element #2=w350:dbl, element #3=w351:dbl, element #5=w304:dbl, element #6=w344:dbl, element #13=w313:dbl, element #15=w311:dbl, element #17=w301:dbl, element #18=w336:dbl, element #19=w337:dbl, element #20=w338:dbl, element #21=w339:dbl, element #22=w346:dbl, element #23=w349:dbl, element #24=→"PPS1_OV" →"PPS 1":dbl, element #27=w348:dbl, element #32=w307:dbl, element #33=w347:dbl, element #39=w306:dbl, element #41=w352:dbl, element #42=w318:dbl, element #43=w319:dbl, element #44=w320:dbl, element #45=w321:dbl, element #46=w322:dbl, element #47=w323:dbl, element #48=w296:dbl)  [unwired: 22 out]
                  n122 = Not Equal To 0?(x=w350) -> (x != 0?=→"ASMS" →"ASMS":bool)
                  n123 = call "assi_state_driver.vi"("ASSI Signal"=w351) -> ("ASSI State"=→"ASSI State" →"ASSI State":string)
                  n124 = call "mission_select.vi"("Data"=w304) -> ("String"=→"Mission selected":string)
                  n125 = Not Equal To 0?(x=w313) -> (x != 0?=→"Driving State Active":bool)
                  n126 = Not Equal To 0?(x=w311) -> (x != 0?=→"EBS Active":bool)
                  n127 = Not Equal To 0?(x=w306) -> (x != 0?=→"nEBS Acitve":bool)
                  n128 = Not Equal To 0?(x=w307) -> (x != 0?=→"Finish State":bool)
                  n129 = Not Equal To 0?(x=w318) -> (x != 0?=→"Dash Heartbeat Error":bool)
                  n130 = Not Equal To 0?(x=w319) -> (x != 0?=→"HVECU Heartbeat Error":bool)
                  n131 = Not Equal To 0?(x=w320) -> (x != 0?=→"MCU Heartbeat Error":bool)
                  n132 = Not Equal To 0?(x=w321) -> (x != 0?=→"Pedal Node Heartbeat Error":bool)
                  n133 = Not Equal To 0?(x=w322) -> (x != 0?=→"Steering Heartbeat Error":bool)
                  n134 = Not Equal To 0?(x=w323) -> (x != 0?=→"TCU Heartbeat Error":bool)
                  n135 = Not Equal To 0?(x=w296) -> (x != 0?=→"Bag Start":bool)
                  n136 = call "as_state_driver.vi"("AS_State"=w352) -> ("Name of state"=→"AS State" →"AS State":string)
                  n137 = Not Equal To 0?(x=w344) -> (x != 0?=→"Brake Light":bool)
                  n138 = Not Equal To 0?(x=w336) -> (x != 0?=→"MCU EF":bool)
                  n139 = Not Equal To 0?(x=w337) -> (x != 0?=→"MCU Front":bool)
                  n140 = Not Equal To 0?(x=w338) -> (x != 0?=→"MCU Rear":bool)
                  n141 = Not Equal To 0?(x=w339) -> (x != 0?=→"MCU RF":bool)
                  n142 = call "car_state_driver.vi"("START"=w347, "RTDS"=w348, "ON"=w349, "OFF"=w346) -> ("Car State"=→"Car State" →"Car State":string)
                  n143 = call "initial_check.vi"("Data"=w301) -> ("String"=→"Initial Checkup":string)
                }
                frame 820 {
                  n144 = Unbundle By Name(w461) -> ("ACCELERATION_LED"=w493:dbl, "AMS_LED"=w492:dbl, "ASB_ERROR_LED"=w491:dbl, "AUTOX_LED"=w490:dbl, "Dashboard_heartbeat_error"=w489:dbl, "EBS_TEST_LED"=w488:dbl, "HVECU_Heartbeat_error"=w487:dbl, "HV_LED"=w486:dbl, "IMD_LED"=w485:dbl, "INSPECTION_LED"=w484:dbl, "MANUAL_MODE_LED"=w483:dbl, "MCU1_LED"=w482:dbl, "MCU2_LED"=w481:dbl, "MCU3_LED"=w480:dbl, "MCU4_LED"=w479:dbl, "MCU_Heartbeat_error"=w478:dbl, "Pedal_Node_Heartbeat_error"=w477:dbl, "SC_BSPD_FB"=w476:dbl, "SC_DV_FB"=w475:dbl, "SC_DV_RELAY_FB"=w474:dbl, "SC_EBS_FB"=w473:dbl, "PPS2"=w395:dbl, "SC_FRONT_FB"=w472:dbl, "SC_HOOP_FB"=w471:dbl, "SC_MCU_FB"=w470:dbl, "SKIDPAD_LED"=w469:dbl, "SSG_Heartbeat"=w468:dbl, "Steering_Heartbeat_error"=w467:dbl, "TCU_Heartbeat_error"=w466:dbl, "TCU_LED"=w465:dbl, "TRACKDRIVE_LED"=w464:dbl, "TS_OFF_LED"=w463:dbl)
                  n145 = Index Array(array=w462, index #1=w493, index #2=w492, index #3=w491, index #4=w490, index #5=w489, index #6=w488, index #7=w487, index #8=w486, index #9=w485, index #10=w484, index #11=w483, index #12=w482, index #13=w481, index #14=w480, index #15=w479, index #16=w478, index #17=w477, index #18=w476, index #19=w475, index #20=w474, index #21=w473, index #22=w395, index #23=w472, index #24=w471, index #25=w470, index #26=w469, index #27=w468, index #28=w467, index #29=w466, index #30=w465, index #31=w464, index #32=w463) -> (element #2=w458:dbl, element #3=w405:dbl, element #8=w457:dbl, element #9=w456:dbl, element #10=w401:dbl, element #12=w455:dbl, element #13=w454:dbl, element #14=w453:dbl, element #15=w452:dbl, element #18=w415:dbl, element #19=w442:dbl, element #20=w441:dbl, element #21=w440:dbl, element #22=→"PPS2_OV" →"PPS 2":dbl, element #23=w439:dbl, element #24=w438:dbl, element #25=w437:dbl, element #26=w400:dbl, element #30=w451:dbl, element #31=w399:dbl, element #32=w450:dbl)  [unwired: 11 out]
                  n146 = Build Array(w415, w442, w441, w440, w439, w438, w437) -> (w460:dbl[])
                  n147 = Equal To 0?(x=w415) -> (x = 0?=→"BSPD Actual":bool)
                  n148 = Equal To 0?(x=w442) -> (x = 0?=→"DV Actual":bool)
                  n149 = Equal To 0?(x=w441) -> (x = 0?=→"DV RELAY Actual":bool)
                  n150 = Equal To 0?(x=w440) -> (x = 0?=→"EBS Actual":bool)
                  n151 = Equal To 0?(x=w439) -> (x = 0?=→"FRONT Actual":bool)
                  n152 = Equal To 0?(x=w438) -> (x = 0?=→"HOOP Actual":bool)
                  n153 = Equal To 0?(x=w437) -> (x = 0?=→"MCU Actual":bool)
                  n154 = call "sc_decode.vi"("SC_bits"=w460) -> ("Place opened"=→"Place Opened":string)
                  n155 = Equal?(x=1.0, y=w405) -> (x = y?=→"ASB Error":bool)
                  n156 = call "4led_driver.vi"("4led signal"=w458) -> ("colorbox"=→"AMS" →"AMS":u32)
                  n157 = call "4led_driver.vi"("4led signal"=w405) -> ("colorbox"=→"ASB" →"ASB" →"ASB":u32)
                  n158 = call "4led_driver.vi"("4led signal"=w457) -> ("colorbox"=→"HV" →"HV":u32)
                  n159 = call "4led_driver.vi"("4led signal"=w456) -> ("colorbox"=→"IMD" →"IMD":u32)
                  n160 = call "4led_driver.vi"("4led signal"=w455) -> ("colorbox"=→"MCU1" →"MCU1":u32)
                  n161 = call "4led_driver.vi"("4led signal"=w454) -> ("colorbox"=→"MCU2" →"MCU2":u32)
                  n162 = call "4led_driver.vi"("4led signal"=w453) -> ("colorbox"=→"MCU3" →"MCU3":u32)
                  n163 = call "4led_driver.vi"("4led signal"=w452) -> ("colorbox"=→"MCU4" →"MCU4":u32)
                  n164 = call "4led_driver.vi"("4led signal"=w451) -> ("colorbox"=→"TCU" →"TCU":u32)
                  n165 = call "4led_driver.vi"("4led signal"=w450) -> ("colorbox"=→"TS OFF" →"TS OFF":u32)
                  n166 = call "4led_driver.vi"("4led signal"=w401) -> ("colorbox"=→"Inspection":u32)
                  n167 = call "4led_driver.vi"("4led signal"=w400) -> ("colorbox"=→"Skidpad":u32)
                  n168 = call "4led_driver.vi"("4led signal"=w399) -> ("colorbox"=→"Trackdrive":u32)
                  n169 = feedback #2() -> (w420:bool)  [unwired: 1 in]
                  "FRONT Stored" <- w420
                  n170 = call "sc_store.vi"("Previous"=w420, "Data"=w439, "Ack"="Ack FRONT") -> ("Boolean"=w421:bool)
                  n171 = feedback-in #2(w421) -> ()
                  n172 = feedback #3() -> (w422:bool)  [unwired: 1 in]
                  "EBS Stored" <- w422
                  n173 = call "sc_store.vi"("Previous"=w422, "Data"=w440, "Ack"="Ack EBS") -> ("Boolean"=w423:bool)
                  n174 = feedback-in #3(w423) -> ()
                  n175 = feedback #4() -> (w418:bool)  [unwired: 1 in]
                  "HOOP Stored" <- w418
                  n176 = call "sc_store.vi"("Previous"=w418, "Data"=w438, "Ack"="Ack HOOP") -> ("Boolean"=w419:bool)
                  n177 = feedback-in #4(w419) -> ()
                  n178 = feedback #5() -> (w426:bool)  [unwired: 1 in]
                  "DV Stored" <- w426
                  n179 = call "sc_store.vi"("Previous"=w426, "Data"=w442, "Ack"="Ack DV") -> ("Boolean"=w427:bool)
                  n180 = feedback-in #5(w427) -> ()
                  n181 = feedback #6() -> (w424:bool)  [unwired: 1 in]
                  "DV RELAY Stored" <- w424
                  n182 = call "sc_store.vi"("Previous"=w424, "Data"=w441, "Ack"="Ack DV RELAY") -> ("Boolean"=w425:bool)
                  n183 = feedback-in #6(w425) -> ()
                  n184 = feedback #7() -> (w428:bool)  [unwired: 1 in]
                  "BSPD Stored" <- w428
                  n185 = call "sc_store.vi"("Previous"=w428, "Data"=w415, "Ack"="Ack BPSD") -> ("Boolean"=w429:bool)
                  n186 = feedback-in #7(w429) -> ()
                  n187 = feedback #8() -> (w416:bool)  [unwired: 1 in]
                  "MCU Stored" <- w416
                  n188 = call "sc_store.vi"("Previous"=w416, "Data"=w437, "Ack"="Ack MCU") -> ("Boolean"=w417:bool)
                  n189 = feedback-in #8(w417) -> ()
                }
                frame 873 {
                  n190 = Unbundle By Name(w522) -> ("Steering_letter1"=w528:dbl, "Steering_letter2"=w527:dbl, "Steering_letter3"=w526:dbl, "Steering_letter4"=w525:dbl, "Steering_letter5"=w524:dbl, "Steering_letter6"=w521:dbl, "Steering_letter7"=w520:dbl, "Steering_letter8"=w519:dbl)
                  n191 = Index Array(array=w523, index #1=w528, index #2=w527, index #3=w526, index #4=w525, index #5=w524, index #6=w521, index #7=w520, index #8=w519) -> (element #1=w508:dbl, element #2=w507:dbl, element #3=w506:dbl, element #4=w505:dbl, element #5=w504:dbl, element #6=w503:dbl, element #7=w502:dbl, element #8=w501:dbl)
                  n192 = Build Array(w506) -> (w514:dbl[])
                  n193 = Build Array(w505) -> (w513:dbl[])
                  n194 = Build Array(w508) -> (w518:dbl[])
                  n195 = Build Array(w507) -> (w517:dbl[])
                  n196 = Build Array(w504) -> (w512:dbl[])
                  n197 = Build Array(w503) -> (w511:dbl[])
                  n198 = Build Array(w502) -> (w510:dbl[])
                  n199 = Build Array(w501) -> (w509:dbl[])
                  n200 = Byte Array To String(unsigned byte array=w514) -> (string=w500:string)
                  n201 = Byte Array To String(unsigned byte array=w518) -> (string=w516:string)
                  n202 = Byte Array To String(unsigned byte array=w513) -> (string=w499:string)
                  n203 = Byte Array To String(unsigned byte array=w512) -> (string=w498:string)
                  n204 = Byte Array To String(unsigned byte array=w510) -> (string=w496:string)
                  n205 = Byte Array To String(unsigned byte array=w517) -> (string=w515:string)
                  n206 = Byte Array To String(unsigned byte array=w511) -> (string=w497:string)
                  n207 = Byte Array To String(unsigned byte array=w509) -> (string=w495:string)
                  n208 = Concatenate Strings(w516, w515, w500, w499, w498, w497, w496, w495) -> (→"Steering display":string)
                }
                frame 1030 {
                  n209 = Unbundle By Name(w533) -> ("EEPROM_STA1_MAX"=w538:dbl, "EEPROM_STA1_MIN"=w537:dbl, "EEPROM_STA2_MAX"=w536:dbl, "EEPROM_STA2_MIN"=w535:dbl)
                  n210 = Index Array(array=w534, index #1=w538, index #2=w537, index #3=w536, index #4=w535) -> (element #1=→"STA1 Max":dbl, element #2=→"STA1 Min":dbl, element #3=→"STA2 Max":dbl, element #4=→"STA2 Min":dbl)
                }
                frame 656 {
                  n211 = Unbundle By Name(w552) -> ("Button1"=w562:dbl, "Button2"=w561:dbl, "Button3"=w560:dbl, "Button4"=w559:dbl, "Rotary1"=w558:dbl, "Rotary2"=w557:dbl, "Rotary3"=w556:dbl, "Rotary4"=w555:dbl, "Rotary5"=w554:dbl, "Steering_heartbeat"=w553:dbl)
                  n212 = Index Array(array=w563, index #1=w562, index #2=w561, index #3=w560, index #4=w559, index #5=w558, index #6=w557, index #7=w556, index #8=w555, index #9=w554, index #10=w553) -> (element #1=w548:dbl, element #2=w549:dbl, element #3=w550:dbl, element #4=w551:dbl, element #5=→"Dial1":dbl, element #6=→"Dial2":dbl, element #7=→"Dial3":dbl, element #8=→"Dial4":dbl, element #9=→"Dial5":dbl)  [unwired: 1 out]
                  n213 = Not Equal To 0?(x=w548) -> (x != 0?=→"Boolean":bool)
                  n214 = Not Equal To 0?(x=w549) -> (x != 0?=→"Boolean 2":bool)
                  n215 = Not Equal To 0?(x=w550) -> (x != 0?=→"Boolean 3":bool)
                  n216 = Not Equal To 0?(x=w551) -> (x != 0?=→"Boolean 4":bool)
                }
                frame 1153 {
                  n217 = Unbundle By Name(w579) -> ("VDC_Brake_Force_Max"=w590:dbl, "VDC_Brake_Balance"=w589:dbl, "VDC_Drop_Parameter_New"=w588:dbl, "VDC_M_Yaw"=w587:dbl, "VDC_M_Yaw_Limit"=w586:dbl, "VDC_Powlim_Approx"=w585:dbl, "VDC_Rear_Reduction"=w584:dbl, "VDC_Lateral_Balance"=w583:dbl, "VDC_Throttle_Bias"=w582:dbl, "VDC_Yaw_Control_Balance"=w581:dbl, "VDC_Yaw_Control_Weight_Selector"=w572:dbl, "VDC_MCU_State"=w569:dbl, "VDC_EPOS_State"=w568:dbl)
                  n218 = Index Array(array=w580, index #1=w590, index #2=w589, index #3=w588, index #4=w587, index #5=w586, index #6=w585, index #7=w584, index #8=w583, index #9=w582, index #10=w581, index #11=w572, index #12=w569, index #13=w568) -> (element #1=→"Brake Force Max":dbl, element #3=→"Drop Param New":dbl, element #4=→"M Yaw":dbl, element #5=→"M Yaw Limit":dbl, element #6=→"Powlim Approx":dbl, element #8=→"Lateral Balance":dbl, element #10=→"Yaw Ctrl Balance" →"Yaw Ctrl Balance":dbl, element #11=→"Yaw Ctrl Weight":dbl, element #12=w565:dbl, element #13=w564:dbl)  [unwired: 3 out]
                  n219 = call "vdc_state_driver.vi"("State Signal"=w565) -> ("VDC State"=→"MCU State":string)
                  n220 = call "vdc_state_driver.vi"("State Signal"=w564) -> ("VDC State"=→"EPOS State":string)
                }
                frame 417 {
                  n221 = Unbundle By Name(w598) -> ("EPOS_Position_actual_value"=w596:dbl, "EPOS_Torque_actual_value"=w595:dbl, "EPOS_Statusword"=w594:dbl)
                  n222 = Index Array(array=w597, index #1=w596, index #2=w595, index #3=w594) -> (element #1=→"EPOS Position":dbl, element #2=→"EPOS Torque":dbl, element #3=→"EPOS Status":dbl)
                }
                frame 896 {
                  n223 = Unbundle By Name(w636) -> ("VDC_Power_Max"=w635:dbl, "VDC_Yaw_Control_P"=w634:dbl, "VDC_Driving_Torque_Multiplier"=w633:dbl, "VDC_Braking_Torque_Multiplier"=w632:dbl, "VDC_RPM_Max"=w627:dbl, "VDC_Powerlimiter_Hardcore_On"=w621:dbl, "VDC_Powerlimiter_Throttle_On"=w620:dbl, "VDC_Powerlimiter_Torque_On"=w619:dbl, "VDC_Powerlimtier_Efficiency_On"=w618:dbl, "VDC_Slip_Control_On"=w611:dbl, "VDC_Traction_Control_On"=w610:dbl, "VDC_Drop_Parameter"=w607:dbl, "VDC_Characteristics"=w605:dbl, "VDC_DV_mode"=w602:dbl, "VDC_Safety_Mode"=w601:dbl)
                  n224 = Index Array(array=w637, index #1=w635, index #2=w634, index #3=w633, index #4=w632, index #5=w627, index #6=w621, index #7=w620, index #8=w619, index #9=w618, index #10=w611, index #11=w610, index #12=w607, index #13=w605, index #14=w602, index #15=w601) -> (element #1=→"Power Max" →"Power Max":dbl, element #2=→"Yaw Ctrl P" →"Yaw Ctrl P":dbl, element #3=→"Drv Torque Mult" →"Drv Torque Mult":dbl, element #4=→"Brk Torque Mult" →"Brk Torque Mult":dbl, element #5=→"RPM Max":dbl, element #6=w617:dbl, element #7=w616:dbl, element #8=w615:dbl, element #9=w614:dbl, element #10=w609:dbl, element #11=w608:dbl, element #12=→"Drop Param":dbl, element #14=w603:dbl, element #15=w599:dbl)  [unwired: 1 out]
                  n225 = Not Equal To 0?(x=w603) -> (x != 0?=→"VDC DV mode":bool)
                  n226 = Not Equal To 0?(x=w599) -> (x != 0?=→"Safety mode":bool)
                  n227 = Not Equal To 0?(x=w614) -> (x != 0?=→"Powlim Efficiency":bool)
                  n228 = Not Equal To 0?(x=w608) -> (x != 0?=→"Traction Ctrl On":bool)
                  n229 = Not Equal To 0?(x=w617) -> (x != 0?=→"Powlim Hardcore":bool)
                  n230 = Not Equal To 0?(x=w616) -> (x != 0?=→"Powlim Throttle":bool)
                  n231 = Not Equal To 0?(x=w615) -> (x != 0?=→"Powlim Torque":bool)
                  n232 = Not Equal To 0?(x=w609) -> (x != 0?=→"Slip Ctrl On":bool)
                }
                frame 1158 {
                  n233 = Unbundle By Name(w652) -> ("VDC_Max_Motor_Torque"=w650:dbl, "VDC_Efficiency_Tune"=w649:dbl, "VDC_Throttle_Breakpoint"=w648:dbl, "VDC_Static_Weight_Distribution"=w647:dbl, "VDC_Launch_Control_Mu"=w646:dbl, "VDC_Target_SoC"=w645:dbl, "VDC_TC_Threshold"=w638:dbl)
                  n234 = Index Array(array=w651, index #1=w650, index #2=w649, index #3=w648, index #4=w647, index #5=w646, index #6=w645, index #7=w638) -> (element #1=→"Max Motor Torque":dbl, element #2=→"Efficiency Tune":dbl, element #3=→"Throttle Breakpoint":dbl, element #4=→"Static Weight Dist":dbl, element #5=→"Launch Ctrl Mu":dbl, element #6=→"Target Soc":dbl)  [unwired: 1 out]
                }
                frame 1159 {
                  n235 = Unbundle By Name(w666) -> ("VDC_Laps"=w664:dbl, "VDC_Track_Length"=w663:dbl, "VDC_Optimal_Slip"=w660:dbl, "VDC_Slip_Control_D"=w659:dbl, "VDC_Slip_Control_P"=w658:dbl, "VDC_Slip_Control_I"=w657:dbl)
                  n236 = Index Array(array=w665, index #1=w664, index #2=w663, index #3=w660, index #4=w659, index #5=w658, index #6=w657) -> (element #1=→"Laps":dbl, element #2=→"Track Length":dbl, element #3=→"Optimal Slip":dbl, element #4=→"Slip Ctrl D":dbl, element #5=→"Slip Ctrl P":dbl, element #6=→"Slip Ctrl I":dbl)
                }
                frame 1157 {
                  n237 = Unbundle By Name(w674) -> ("VDC_Fz_FL"=w680:dbl, "VDC_Fz_FR"=w679:dbl, "VDC_Fz_RL"=w678:dbl, "VDC_Fz_RR"=w677:dbl, "VDC_Torque_Demand"=w676:dbl, "TCU_CPU_Usage_Max"=w668:dbl)
                  n238 = Index Array(array=w675, index #1=w680, index #2=w679, index #3=w678, index #4=w677, index #5=w676, index #6=w668) -> (element #1=→"Fz FL":dbl, element #2=→"Fz FR":dbl, element #3=→"Fz RL":dbl, element #4=→"Fz RR":dbl, element #5=→"Torque Demand" →"Torque Demand":dbl, element #6=→"TCU CPU Usage":dbl)
                }
                frame 617 {
                  n239 = Unbundle By Name(w703) -> ("v_x"=w701:dbl, "AccX_Rear"=w699:dbl, "AccY_Rear"=w698:dbl, "Yaw_Rate_Rear"=w691:dbl)
                  n240 = Index Array(array=w702, index #1=w701, index #2=w699, index #3=w698, index #4=w691) -> (element #1=w700:dbl, element #2=w693:dbl, element #3=w692:dbl, element #4=→"Yaw Rear":dbl)
                  "AccX Rear" <- w693
                  "AccY Rear" <- w692
                  n241 = Multiply(x=-1.0 ("y"), y=w693) -> (x*y=w694:dbl)
                  n242 = Multiply(x=w700, y=3.6) -> (x*y=→"Speed [km/h]" →"Velocity X [km/h]":dbl)
                  n243 = Build Array(w694) -> (w697:dbl[])
                  n244 = Build Array(w692) -> (w696:dbl[])
                  n245 = local read "AccX Front"() -> (w688:dbl)
                  n246 = local read "AccY Front"() -> (w684:dbl)
                  n247 = Bundle(w697, w696) -> (w682:cluster{dbl[], dbl[]})  [unwired: 1 in]
                  n248 = Multiply(x=-1.0 ("y"), y=w688) -> (x*y=w685:dbl)
                  n249 = Build Array(w685) -> (w687:dbl[])
                  n250 = Build Array(w684) -> (w686:dbl[])
                  n251 = Bundle(w687, w686) -> (w683:cluster{dbl[], dbl[]})  [unwired: 1 in]
                  n252 = Build Array(w683, w682) -> (→"g-g Graph" →"g-g Graph 3":cluster{dbl[], dbl[]}[])
                }
                frame 1155 {
                  n253 = Unbundle By Name(w851) -> ("Validity_Error_APPS1"=w849:dbl, "Validity_Error_APPS2"=w848:dbl, "Validity_Error_AccX_Front"=w847:dbl, "Validity_Error_AccX_Rear"=w846:dbl, "Validity_Error_AccY_Front"=w845:dbl, "Validity_Error_AccY_Rear"=w844:dbl, "Validity_Error_HV_Cell_Temp"=w843:dbl, "Validity_Error_BFS"=w842:dbl, "Validity_Error_BPS_front"=w841:dbl, "Validity_Error_BPS_rear"=w840:dbl, "Validity_Error_Button1"=w839:dbl, "Validity_Error_Button2"=w838:dbl, "Validity_Error_Button3"=w837:dbl, "Validity_Error_Button4"=w836:dbl, "Validity_Error_HV_Cell_Voltage"=w835:dbl, "Validity_Error_SC_Endline"=w834:dbl, "Validity_Error_HV_Current"=w833:dbl, "Validity_Error_HV_Voltage"=w832:dbl, "Validity_Error_Rotary1"=w831:dbl, "Validity_Error_Rotary2"=w830:dbl, "Validity_Error_Rotary3"=w829:dbl, "Validity_Error_Rotary4"=w828:dbl, "Validity_Error_Rotary5"=w827:dbl, "Validity_Error_STA1"=w826:dbl, "Validity_Error_STA2"=w825:dbl, "Validity_Error_Yaw_Rate_Front"=w824:dbl, "Validity_Error_Yaw_Rate_Rear"=w823:dbl)
                  n254 = Index Array(array=w850, index #1=w849, index #2=w848, index #3=w847, index #4=w846, index #5=w845, index #6=w844, index #7=w843, index #8=w842, index #9=w841, index #10=w840, index #11=w839, index #12=w838, index #13=w837, index #14=w836, index #15=w835, index #16=w834, index #17=w833, index #18=w832, index #19=w831, index #20=w830, index #21=w829, index #22=w828, index #23=w827, index #24=w826, index #25=w825, index #26=w824, index #27=w823) -> (element #1=w822:dbl, element #2=w821:dbl, element #3=w820:dbl, element #4=w819:dbl, element #5=w818:dbl, element #6=w817:dbl, element #7=w816:dbl, element #8=w815:dbl, element #9=w814:dbl, element #10=w813:dbl, element #11=w812:dbl, element #12=w811:dbl, element #13=w810:dbl, element #14=w809:dbl, element #15=w808:dbl, element #16=w807:dbl, element #17=w806:dbl, element #18=w805:dbl, element #19=w804:dbl, element #20=w803:dbl, element #21=w802:dbl, element #22=w801:dbl, element #23=w800:dbl, element #24=w799:dbl, element #25=w798:dbl, element #26=w797:dbl, element #27=w796:dbl)
                  n255 = Not Equal To 0?(x=w822) -> (x != 0?=→"APPS1 Validity":bool)
                  n256 = Not Equal To 0?(x=w821) -> (x != 0?=→"APPS2 Validity":bool)
                  n257 = Not Equal To 0?(x=w820) -> (x != 0?=→"AccX Front Validity":bool)
                  n258 = Not Equal To 0?(x=w819) -> (x != 0?=→"AccX Rear Validity":bool)
                  n259 = Not Equal To 0?(x=w818) -> (x != 0?=→"Accy Front Validity":bool)
                  n260 = Not Equal To 0?(x=w817) -> (x != 0?=→"AccY Rear Validity":bool)
                  n261 = Not Equal To 0?(x=w816) -> (x != 0?=→"HV Cell Temp Validity":bool)
                  n262 = Not Equal To 0?(x=w815) -> (x != 0?=→"BFS Validity":bool)
                  n263 = Not Equal To 0?(x=w814) -> (x != 0?=→"BPS Front Validity":bool)
                  n264 = Not Equal To 0?(x=w813) -> (x != 0?=→"BPS Rear Validity":bool)
                  n265 = Not Equal To 0?(x=w812) -> (x != 0?=→"Button1 Validity":bool)
                  n266 = Not Equal To 0?(x=w811) -> (x != 0?=→"Button2 Validity":bool)
                  n267 = Not Equal To 0?(x=w810) -> (x != 0?=→"Button3 Validity":bool)
                  n268 = Not Equal To 0?(x=w809) -> (x != 0?=→"Button4 Validity":bool)
                  n269 = Not Equal To 0?(x=w808) -> (x != 0?=→"HV Cell Voltage Validity":bool)
                  n270 = Not Equal To 0?(x=w807) -> (x != 0?=→"SC Endline Validity":bool)
                  n271 = Not Equal To 0?(x=w806) -> (x != 0?=→"HV Current Validity":bool)
                  n272 = Not Equal To 0?(x=w805) -> (x != 0?=→"HV Voltage Validity":bool)
                  n273 = Not Equal To 0?(x=w804) -> (x != 0?=→"Rotary1 Validity":bool)
                  n274 = Not Equal To 0?(x=w803) -> (x != 0?=→"Rotary2 Validity":bool)
                  n275 = Not Equal To 0?(x=w802) -> (x != 0?=→"Rotary3 Validity":bool)
                  n276 = Not Equal To 0?(x=w801) -> (x != 0?=→"Rotary4 Validity":bool)
                  n277 = Not Equal To 0?(x=w800) -> (x != 0?=→"Rotary5 Validity":bool)
                  n278 = Not Equal To 0?(x=w799) -> (x != 0?=→"STA1 Validity":bool)
                  n279 = Not Equal To 0?(x=w798) -> (x != 0?=→"STA2 Validity":bool)
                  n280 = Not Equal To 0?(x=w797) -> (x != 0?=→"Yaw Front Validity":bool)
                  n281 = Not Equal To 0?(x=w796) -> (x != 0?=→"Yaw Rear Validity":bool)
                  n282 = Unbundle By Name(w851) -> ("Timeout_Error_Rotary3"=w768:dbl, "Timeout_Error_Rotary2"=w767:dbl, "Timeout_Error_Rotary1"=w766:dbl, "Timeout_Error_BFS"=w765:dbl, "Timeout_Error_HV_Current"=w764:dbl, "Timeout_Error_HV_Cell_Temp"=w763:dbl, "Timeout_Error_BPS_Rear"=w762:dbl, "Timeout_Error_Rotary4"=w761:dbl, "Timeout_Error_BPS_Front"=w760:dbl, "Timeout_Error_AccY_Rear"=w759:dbl, "Timeout_Error_AccY_Front"=w758:dbl, "Timeout_Error_AccX_Rear"=w757:dbl, "Timeout_Error_AccX_Front"=w756:dbl, "Timeout_Error_APPS2"=w755:dbl, "Timeout_Error_APPS1"=w754:dbl, "Timeout_Error_Rotary5"=w753:dbl, "Timeout_Error_SC_Endline"=w752:dbl, "Validity_Error_DV_Target_Speed"=w717:dbl, "Validity_Error_DV_Target_Angle"=w716:dbl, "Timeout_Error_SSG_Status1"=w715:dbl, "Timeout_Error_Xavier"=w714:dbl)
                  n283 = Index Array(array=w850, index #1=w768, index #2=w767, index #3=w766, index #4=w765, index #5=w764, index #6=w763, index #7=w762, index #8=w761, index #9=w760, index #10=w759, index #11=w758, index #12=w757, index #13=w756, index #14=w755, index #15=w754, index #16=w753, index #17=w752, index #18=w717, index #19=w716, index #20=w715, index #21=w714) -> (element #1=w751:dbl, element #2=w750:dbl, element #3=w749:dbl, element #4=w735:dbl, element #5=w748:dbl, element #6=w747:dbl, element #7=w746:dbl, element #8=w745:dbl, element #9=w744:dbl, element #10=w743:dbl, element #11=w742:dbl, element #12=w741:dbl, element #13=w740:dbl, element #14=w739:dbl, element #15=w738:dbl, element #16=w737:dbl, element #17=w736:dbl, element #18=w709:dbl, element #19=w708:dbl, element #20=w707:dbl, element #21=w706:dbl)
                  n284 = Not Equal To 0?(x=w707) -> (x != 0?=→"SSG Status1 Timeout":bool)
                  n285 = Not Equal To 0?(x=w706) -> (x != 0?=→"Xavier Timeout":bool)
                  n286 = Not Equal To 0?(x=w709) -> (x != 0?=→"DV Target Angle Validity":bool)
                  n287 = Not Equal To 0?(x=w708) -> (x != 0?=→"DV Target Speed Validity":bool)
                  n288 = Not Equal To 0?(x=w751) -> (x != 0?=→"Rotary3 Timeout":bool)
                  n289 = Not Equal To 0?(x=w750) -> (x != 0?=→"Rotary2 Timeout":bool)
                  n290 = Not Equal To 0?(x=w749) -> (x != 0?=→"Rotary1 Timeout":bool)
                  n291 = Not Equal To 0?(x=w748) -> (x != 0?=→"HV Current Timeout":bool)
                  n292 = Not Equal To 0?(x=w747) -> (x != 0?=→"HV Cell Temp Timeout":bool)
                  n293 = Not Equal To 0?(x=w746) -> (x != 0?=→"BPS Rear Timeout":bool)
                  n294 = Not Equal To 0?(x=w745) -> (x != 0?=→"Rotary4 Timeout":bool)
                  n295 = Not Equal To 0?(x=w744) -> (x != 0?=→"BPS Front Timeout":bool)
                  n296 = Not Equal To 0?(x=w743) -> (x != 0?=→"AccY Rear Timeout":bool)
                  n297 = Not Equal To 0?(x=w742) -> (x != 0?=→"AccY FrontTimeout":bool)
                  n298 = Not Equal To 0?(x=w741) -> (x != 0?=→"AccX Rear Timeout":bool)
                  n299 = Not Equal To 0?(x=w740) -> (x != 0?=→"AccX Front Timeout":bool)
                  n300 = Not Equal To 0?(x=w739) -> (x != 0?=→"APPS2 Timeout":bool)
                  n301 = Not Equal To 0?(x=w738) -> (x != 0?=→"APPS1 Timeout":bool)
                  n302 = Not Equal To 0?(x=w737) -> (x != 0?=→"Rotary5 Timeout":bool)
                  n303 = Not Equal To 0?(x=w736) -> (x != 0?=→"SC Endline Timeout":bool)
                  n304 = Not Equal To 0?(x=w735) -> (x != 0?=→"BFS Timeout":bool)
                }
                frame 1029 {
                  n305 = Unbundle By Name(w856) -> ("EEPROM_APPS1_MAX"=w861:dbl, "EEPROM_APPS1_MIN"=w860:dbl, "EEPROM_APPS2_MAX"=w859:dbl, "EEPROM_APPS2_MIN"=w858:dbl)
                  n306 = Index Array(array=w857, index #1=w861, index #2=w860, index #3=w859, index #4=w858) -> (element #1=→"APPS1 Max":dbl, element #2=→"APPS1 Min":dbl, element #3=→"APPS2 Max":dbl, element #4=→"APPS2 Min":dbl)
                }
                frame 560 {
                  n307 = Unbundle By Name(w892) -> ("APPS1_position"=w903:dbl, "APPS1_validity"=w902:dbl, "APPS2_posiition"=w901:dbl, "APPS2_validity"=w900:dbl, "APPS_plausiblity"=w899:dbl, "STA1_position"=w898:dbl, "STA1_validity"=w897:dbl, "STA2_position"=w896:dbl, "STA2_validity"=w895:dbl, "STA_plausiblity"=w894:dbl)
                  n308 = Index Array(array=w893, index #1=w903, index #2=w902, index #3=w901, index #4=w900, index #5=w899, index #6=w898, index #7=w897, index #8=w896, index #9=w895, index #10=w894) -> (element #1=w865:dbl, element #2=w891:dbl, element #3=w864:dbl, element #4=w888:dbl, element #5=w881:dbl, element #6=w862:dbl, element #7=w887:dbl, element #8=w863:dbl, element #9=w885:dbl, element #10=w880:dbl)
                  "STA1_OV" <- w862
                  "STA2_OV" <- w863
                  "APPS1_OV" <- w865
                  "APPS2_OV" <- w864
                  "APPS 2" <- w864
                  "APPS 1" <- w865
                  "STA 2" <- w863
                  "STA 1" <- w862
                  n309 = Equal?(x=w881, y=1.0) -> (x = y?=→"APPS_plaus" →"Plausability" →"APPS Plausability":bool)
                  n310 = Equal?(x=w891, y=1.0) -> (x = y?=w871:bool)
                  "APPS1_bool" <- w871
                  "APPS1 Validity" <- w871
                  n311 = Equal?(x=w888, y=1.0) -> (x = y?=w870:bool)
                  "APPS2_bool" <- w870
                  "APPS2 Validity" <- w870
                  n312 = Equal?(x=w887, y=1.0) -> (x = y?=w869:bool)
                  "STA1_bool" <- w869
                  "STA1 Validity" <- w869
                  n313 = Equal?(x=w885, y=1.0) -> (x = y?=w868:bool)
                  "STA2_bool" <- w868
                  "STA2 Validity" <- w868
                  n314 = Equal?(x=w880, y=1.0) -> (x = y?=→"STA_plaus" →"Plausability" →"STA Plausability":bool)
                  n315 = Add(x=w865, y=w864) -> (x+y=w879:dbl)
                  n316 = Add(x=w862, y=w863) -> (x+y=w875:dbl)
                  n317 = Divide(x=w879, y=2.0) -> (x/y=→"APPS Avg":dbl)
                  n318 = Divide(x=w875, y=2.0) -> (x/y=→"STA Avg":dbl)
                  n319 = And(x=w869, y=w868) -> (x .and. y?=→"Validity":bool)
                  n320 = And(x=w871, y=w870) -> (x .and. y?=→"Validity":bool)
                }
                frame 105 {
                  n321 = Unbundle By Name(w919) -> ("Xavier_AS_Finish"=w924:dbl, "Xavier_Target_Wheel_Angle"=w923:dbl, "Xavier_Target_speed"=w922:dbl, "Xavier_Control_heartbeat"=w921:dbl)
                  n322 = local read "STA2_OV"() -> (w912:u8)
                  n323 = local read "STA1_OV"() -> (w913:u8)
                  n324 = Add(x=w913, y=w912) -> (x+y=w911:u8)
                  n325 = Divide(x=w911, y=u8 2) -> (x/y=w909:dbl)
                  n326 = Index Array(array=w920, index #1=w924, index #2=w923, index #3=w922, index #4=w921) -> (element #2=w918:dbl, element #3=w905:dbl)  [unwired: 2 out]
                  n327 = Subtract(x=w909, y=105.0) -> (x-y=w907:dbl)
                  n328 = expression code="(x/pi)*180.0" ("radians to degrees")(w918) -> (w906:dbl)
                  "Target Steer" <- w906
                  "Target Steer 2" <- w906
                  n329 = local read "Velocity X [km/h]"() -> (w915:dbl)
                  n330 = Multiply(x=w905, y=3.6) -> (x*y=w904:dbl)
                  "Target Speed" <- w904
                  n331 = Bundle(w904, "Velocity X [km/h]"=w915) -> (→"Target vs Actual Velocity":cluster{dbl, "Velocity X [km/h]":dbl})  [unwired: 1 in]
                  n332 = Bundle("Data"=w906, w907) -> (→"Target vs Actual steer\nSteer":cluster{"Data":dbl, dbl})  [unwired: 1 in]
                }
                frame 848 {
                  n333 = Unbundle By Name(w953) -> ("Xavier_CPU1_usage"=w951:dbl, "Xavier_CPU2_usage"=w950:dbl, "Xavier_CPU3_usage"=w949:dbl, "Xavier_CPU4_usage"=w948:dbl, "Xavier_CPU5_usage"=w947:dbl, "Xavier_CPU6_usage"=w946:dbl, "Xavier_CPU7_usage"=w945:dbl, "Xavier_CPU8_usage"=w944:dbl, "Xavier_RAM_usage"=w932:dbl, "Xavier_MAX_temperature"=w943:dbl, "Xavier_Power_Consuption"=w942:dbl)
                  n334 = Index Array(array=w952, index #1=w951, index #2=w950, index #3=w949, index #4=w948, index #5=w947, index #6=w946, index #7=w945, index #8=w944, index #9=w932, index #10=w943, index #11=w942) -> (element #1=→"CPU1":dbl, element #2=→"CPU2":dbl, element #3=→"CPU3":dbl, element #4=→"CPU4":dbl, element #5=→"CPU5":dbl, element #6=→"CPU6":dbl, element #7=→"CPU7":dbl, element #8=→"CPU8":dbl, element #9=→"RAM":dbl, element #10=→"Xavier Max Temp [°C]":dbl, element #11=w926:dbl)
                  n335 = Divide(x=w926, y=10.0) -> (x/y=w930:dbl)
                  n336 = Round To Nearest(number=w930) -> (nearest integer value=w929:dbl)
                  n337 = Divide(x=w929, y=100.0) -> (x/y=→"Xavier Power [W]":dbl)
                }
                frame 849 {
                  n338 = Unbundle By Name(w971) -> ("Xavier_crossTrackError"=w969:dbl, "Xavier_headingError"=w968:dbl, "Xavier_current_laps"=w967:dbl, "Xavier_headingErrorSS"=w966:dbl, "Xavier_steeringAngleError"=w965:dbl, "Xavier_target_laps"=w964:dbl, "Xavier_yawRateError"=w963:dbl)
                  n339 = Index Array(array=w970, index #1=w969, index #2=w968, index #3=w967, index #4=w966, index #5=w965, index #6=w964, index #7=w963) -> (element #1=w957:dbl, element #2=w959:dbl, element #3=→"Current laps":dbl, element #4=w955:dbl, element #5=w958:dbl, element #6=→"Target laps":dbl, element #7=w954:dbl)
                  n340 = Bundle("Data"=w959, "Data"=w958, "Data"=w957) -> (→"Heading-Steering-Crosstrack":cluster{"Data":dbl, "Data":dbl, "Data":dbl})  [unwired: 1 in]
                  n341 = Bundle("Data"=w955, "Data"=w954) -> (→"HeadingSS-Yaw":cluster{"Data":dbl, "Data":dbl})  [unwired: 1 in]
                }
                frame 850 {
                  w988 = T15 {"Color"=0, "Id"=0, "PosX"=0.0, "PosY"=0.0}  # Landmark_format
                  n342 = Unbundle By Name(w1023) -> ("Xavier_eff_n_particles"=w1021:dbl, "Xavier_landmark_color"=w1020:dbl, "Xavier_landmark_id"=w1019:dbl, "Xavier_landmark_x"=w1018:dbl, "Xavier_landmark_y"=w1017:dbl, "Xavier_loopClosed"=w1016:dbl, "Xavier_missionFinished"=w1015:dbl, "Xavier_n_updates_last_resample"=w1014:dbl, "Xavier_runtime"=w1013:dbl)
                  n343 = Build Array(w988) -> (w986:T16)
                  n344 = local read "Car orient"() -> (w998:dbl)
                  n345 = feedback #9(w986) -> (w985:T16)
                  n346 = Cosine(x=w998) -> (cos(x)=w999:dbl)
                  n347 = Sine(x=w998) -> (sin(x)=w1000:dbl)
                  n348 = Index Array(array=w1022, index #1=w1021, index #2=w1020, index #3=w1019, index #4=w1018, index #5=w1017, index #6=w1016, index #7=w1015, index #8=w1014, index #9=w1013) -> (element #1=→"Eff n Particles":dbl, element #2=w973:dbl, element #3=w974:dbl, element #4=w975:dbl, element #5=w976:dbl, element #6=w1006:dbl, element #7=w1007:dbl, element #8=→"Updates last resample":dbl, element #9=→"Runtime":dbl)
                  n349 = Equal To 0?(x=w974) -> (x = 0?=w989:bool)
                  n350 = Equal To 0?(x=w973) -> (x = 0?=w995:bool)
                  n351 = Equal To 0?(x=w975) -> (x = 0?=w990:bool)
                  n352 = Equal To 0?(x=w976) -> (x = 0?=w991:bool)
                  n353 = And(x=w990, y=w991) -> (x .and. y?=w992:bool)
                  n354 = And(x=w989, y=w995) -> (x .and. y?=w993:bool)
                  n355 = And(x=w993, y=w992) -> (x .and. y?=w994:bool)
                  n356 = Not(x=w994) -> (.not. x?=w972:bool)
                  n357 = case shown="True" w972 {
                    tunnel: w974 -> [_ w1069]
                    tunnel: w973 -> [_ w1068]
                    tunnel: w975 -> [_ w1067]
                    tunnel: w976 -> [_ w1066]
                    tunnel: w988 -> [_ w1070]
                    tunnel: [w1031 w1062] -> w977
                    tunnel: [w1030 w1061] -> w978
                    tunnel: [w1028 w1059] -> w980
                    tunnel: [w1029 w1060] -> w979
                    tunnel: [w1027 w1058] -> w984
                    tunnel: [w1026 w1057] -> w983
                    tunnel: [w1025 w1056] -> w982
                    tunnel: [w1024 w1055] -> w981
                    tunnel: [w1032 w1063] -> w987
                    tunnel: w985 -> [w1032 w1064]
                    frame False {
                      n358 = for {
                        tunnel: w1032 -> [w1034] mode=indexing
                        tunnel: [w1042] -> w1031 mode=indexing
                        tunnel: [w1041] -> w1030 mode=indexing
                        tunnel: [w1040] -> w1029 mode=indexing
                        tunnel: [w1039] -> w1028 mode=indexing
                        tunnel: [w1038] -> w1027 mode=indexing
                        tunnel: [w1037] -> w1026 mode=indexing
                        tunnel: [w1036] -> w1025 mode=indexing
                        tunnel: [w1035] -> w1024 mode=indexing
                        n359 = Unbundle By Name(w1034) -> ("Color"=w1033:i32)
                        n360 = case shown="3" w1033 {
                          tunnel: w1034 -> [w1045 w1048 w1051 w1054 _]
                          tunnel: [_ _ w1050 _ _] -> w1042
                          tunnel: [_ _ w1049 _ _] -> w1041
                          tunnel: [_ w1047 _ _ _] -> w1040
                          tunnel: [_ w1046 _ _ _] -> w1039
                          tunnel: [_ _ _ w1052 _] -> w1038
                          tunnel: [_ _ _ w1053 _] -> w1037
                          tunnel: [w1044 _ _ _ _] -> w1036
                          tunnel: [w1043 _ _ _ _] -> w1035
                          frame 0 {
                            n361 = Unbundle By Name(w1045) -> ("PosY"=w1044:dbl, "PosX"=w1043:dbl)
                          }
                          frame 1 {
                            n362 = Unbundle By Name(w1048) -> ("PosY"=w1047:dbl, "PosX"=w1046:dbl)
                          }
                          frame 2 {
                            n363 = Unbundle By Name(w1051) -> ("PosY"=w1050:dbl, "PosX"=w1049:dbl)
                          }
                          frame 3 {
                            n364 = Unbundle By Name(w1054) -> ("PosY"=w1052:dbl, "PosX"=w1053:dbl)
                          }
                          frame 4, Default {
                          }
                        }
                      }
                    }
                    frame True {
                      n365 = for {
                        tunnel: w1064 -> [w1115] mode=indexing
                        tunnel: [w1114] -> w1073 mode=indexing
                        n366 = Unbundle By Name(w1115) -> ("Id"=w1114:i32)
                      }
                      n367 = Search 1D Array(1D array=w1073, element=w1069) -> (index of element=w1065:i32)  [unwired: 1 in]
                      n368 = Equal?(x=w1065, y=-1) -> (x = y?=w1072:bool)
                      n369 = case shown="False" w1072 {
                        tunnel: w1064 -> [w1100 w1112]
                        tunnel: w1070 -> [w1096 w1110]
                        tunnel: w1069 -> [w1104 w1109]
                        tunnel: w1068 -> [w1103 w1108]
                        tunnel: w1067 -> [w1102 w1107]
                        tunnel: w1066 -> [w1101 w1106]
                        tunnel: [w1099 w1105] -> w1063
                        tunnel: w1065 -> [w1098 _]
                        frame False {
                          n370 = Bundle By Name(cluster=w1096, "Id"=w1104, "Color"=w1103, "PosX"=w1102, "PosY"=w1101) -> (w1097:T15)
                          n371 = Replace Array Subset(array=w1100, new element=w1097, index=w1098) -> (w1099:T16)
                        }
                        frame True {
                          n372 = Bundle By Name(cluster=w1110, "Id"=w1109, "Color"=w1108, "PosX"=w1107, "PosY"=w1106) -> (w1111:T15)
                          n373 = Array Size(array=w1112) -> (size(s)=w1113:i32)
                          n374 = Insert Into Array(array=w1112, index=w1113, new element=w1111) -> (w1105:T16)
                        }
                      }
                      n375 = for {
                        tunnel: w1063 -> [w1075] mode=indexing
                        tunnel: [w1083] -> w1062 mode=indexing
                        tunnel: [w1082] -> w1061 mode=indexing
                        tunnel: [w1081] -> w1060 mode=indexing
                        tunnel: [w1080] -> w1059 mode=indexing
                        tunnel: [w1079] -> w1058 mode=indexing
                        tunnel: [w1078] -> w1057 mode=indexing
                        tunnel: [w1077] -> w1056 mode=indexing
                        tunnel: [w1076] -> w1055 mode=indexing
                        n376 = Unbundle By Name(w1075) -> ("Color"=w1074:i32)
                        n377 = case shown="0" w1074 {
                          tunnel: w1075 -> [w1086 w1089 w1092 w1095 _]
                          tunnel: [_ _ w1091 _ _] -> w1083
                          tunnel: [_ _ w1090 _ _] -> w1082
                          tunnel: [_ w1088 _ _ _] -> w1081
                          tunnel: [_ w1087 _ _ _] -> w1080
                          tunnel: [_ _ _ w1093 _] -> w1079
                          tunnel: [_ _ _ w1094 _] -> w1078
                          tunnel: [w1085 _ _ _ _] -> w1077
                          tunnel: [w1084 _ _ _ _] -> w1076
                          frame 0 {
                            n378 = Unbundle By Name(w1086) -> ("PosY"=w1085:dbl, "PosX"=w1084:dbl)
                          }
                          frame 1 {
                            n379 = Unbundle By Name(w1089) -> ("PosY"=w1088:dbl, "PosX"=w1087:dbl)
                          }
                          frame 2 {
                            n380 = Unbundle By Name(w1092) -> ("PosY"=w1091:dbl, "PosX"=w1090:dbl)
                          }
                          frame 3 {
                            n381 = Unbundle By Name(w1095) -> ("PosY"=w1093:dbl, "PosX"=w1094:dbl)
                          }
                          frame 4, Default {
                          }
                        }
                      }
                    }
                  }
                  n382 = feedback-in #9(w987) -> ()
                  n383 = Multiply(x=w999, y="Arrow size") -> (x*y=w1003:dbl)
                  n384 = Multiply(x="Arrow size", y=w1000) -> (x*y=w1002:dbl)
                  n385 = local read "Car pos"() -> (w997:dbl[])
                  n386 = Build Array(w1003, w1002) -> (w996:dbl[])
                  n387 = Not Equal To 0?(x=w1006) -> (x != 0?=→"Loop Closed":bool)
                  n388 = Not Equal To 0?(x=w1007) -> (x != 0?=→"Mission Finished":bool)
                  n389 = call "map_controller.vi"("eps"="Arrow thickness", "redy"=w977, "redx"=w978, "bluex"=w981, "yellowx"=w980, "bluey"=w982, "yellowy"=w979, "pos"=w997, "vec"=w996, "orangey"=w984, "orangex"=w983) -> ("Map object out"=→"Map":cluster{"orangex":dbl[], "orangey":dbl[]}[])
                }
                frame 851 {
                  n390 = Unbundle By Name(w1136) -> ("Xavier_position_x"=w1134:dbl, "Xavier_position_y"=w1133:dbl, "Xavier_orientation"=w1132:dbl, "Xavier_all_landmarks"=w1131:dbl, "Xavier_Yolo_yellow"=w1130:dbl, "Xavier_current_landmarks"=w1129:dbl, "Xavier_Yolo_orange_small"=w1128:dbl, "Xavier_Yolo_orange_big"=w1127:dbl, "Xavier_Yolo_blue"=w1126:dbl)
                  n391 = Index Array(array=w1135, index #1=w1134, index #2=w1133, index #3=w1132, index #4=w1131, index #5=w1130, index #6=w1129, index #7=w1128, index #8=w1127, index #9=w1126) -> (element #1=w1118:dbl, element #2=w1117:dbl, element #3=→"Car orient":dbl, element #4=→"All landmarks":dbl, element #5=→"Yellow count":dbl, element #6=→"Current landmarks":dbl, element #7=→"Orange count":dbl, element #8=→"Red count":dbl, element #9=→"Blue count":dbl)
                  n392 = Build Array(w1118, w1117) -> (→"Car pos":dbl[])
                }
                frame 648 {
                  n393 = Unbundle By Name(w1142) -> ("AMK3_actual_velocity"=w1144:dbl, "AMK3_magnetizing_current"=w1147:dbl, "AMK3_status"=w1146:dbl, "AMK3_torque_current"=w1145:dbl)
                  n394 = Index Array(array=w1143, index #1=w1144, index #2=w1147, index #3=w1146, index #4=w1145) -> (element #1=→"Actual_vel_RL_OV":dbl, element #2=→"Im RL":dbl, element #3=w1137:dbl, element #4=→"It RL":dbl)
                  n395 = Number To Boolean Array(number=w1137) -> (Boolean array=→"RL Status":bool[])
                }
                frame 649 {
                  n396 = Unbundle By Name(w1153) -> ("AMK4_actual_velocity"=w1155:dbl, "AMK4_magnetizing_current"=w1158:dbl, "AMK4_status"=w1157:dbl, "AMK4_torque_current"=w1156:dbl)
                  n397 = Index Array(array=w1154, index #1=w1155, index #2=w1158, index #3=w1157, index #4=w1156) -> (element #1=→"Actual_vel_RR_OV":dbl, element #2=→"Im RR":dbl, element #3=w1148:dbl, element #4=→"It RR":dbl)
                  n398 = Number To Boolean Array(number=w1148) -> (Boolean array=→"RR Status":bool[])
                }
                frame 650 {
                  n399 = Unbundle By Name(w1164) -> ("AMK3_error_info"=w1166:dbl, "AMK3_temp_IGBT"=w1169:dbl, "AMK3_temp_inverter"=w1168:dbl, "AMK3_temp_motor"=w1167:dbl)
                  n400 = Index Array(array=w1165, index #1=w1166, index #2=w1169, index #3=w1168, index #4=w1167) -> (element #1=w1160:dbl, element #2=w1161:dbl, element #3=w1159:dbl, element #4=w1162:dbl)
                  "Error info RL" <- w1160
                  "Temp IGBT RL" <- w1161
                  "Temp Motor RL" <- w1162
                  "Temp inv RL" <- w1159
                  "RL Error info" <- w1160
                  "Temp Inv RL" <- w1159
                  n401 = local write "Temp inv RL"(w1159) -> ()
                  n402 = Build Array(w1160, w1161, w1159, w1162) -> (→"RL":dbl[])
                }
                frame 651 {
                  n403 = Unbundle By Name(w1175) -> ("AMK4_error_info"=w1177:dbl, "AMK4_temp_IGBT"=w1180:dbl, "AMK4_temp_inverter"=w1179:dbl, "AMK4_temp_motor"=w1178:dbl)
                  n404 = Index Array(array=w1176, index #1=w1177, index #2=w1180, index #3=w1179, index #4=w1178) -> (element #1=w1171:dbl, element #2=w1172:dbl, element #3=w1170:dbl, element #4=w1173:dbl)
                  "Error info RR" <- w1171
                  "Temp IGBT RR" <- w1172
                  "Temp Motor RR" <- w1173
                  "Temp inv RR" <- w1170
                  "RR Error info" <- w1171
                  "Temp Inv RR" <- w1170
                  n405 = local write "Temp inv RR"(w1170) -> ()
                  n406 = Build Array(w1171, w1172, w1170, w1173) -> (→"RR":dbl[])
                }
                frame 1378 {
                  n407 = Unbundle By Name(w1197) -> ("Button_OFF"=w1199:dbl, "Button_ON"=w1202:dbl, "Button_START"=w1201:dbl, "Dash_BLANK"=w1200:dbl, "Dash_MODE"=w1196:dbl, "Dash_XLAT"=w1195:dbl, "Dashboard_ID"=w1194:dbl, "Dashboarrd_heartbeat"=w1193:dbl)
                  n408 = Index Array(array=w1198, index #1=w1199, index #2=w1202, index #3=w1201, index #4=w1200, index #5=w1196, index #6=w1195, index #7=w1194, index #8=w1193) -> (element #1=w1187:dbl, element #2=w1188:dbl, element #3=w1189:dbl, element #4=w1190:dbl, element #5=w1191:dbl, element #6=w1192:dbl)  [unwired: 2 out]
                  n409 = Not Equal To 0?(x=w1187) -> (x != 0?=→"OFF":bool)
                  n410 = Not Equal To 0?(x=w1188) -> (x != 0?=→"ON":bool)
                  n411 = Not Equal To 0?(x=w1189) -> (x != 0?=→"START":bool)
                  n412 = Not Equal To 0?(x=w1190) -> (x != 0?=→"BLANK":bool)
                  n413 = Not Equal To 0?(x=w1191) -> (x != 0?=→"MODE":bool)
                  n414 = Not Equal To 0?(x=w1192) -> (x != 0?=→"XLAT":bool)
                }
                frame 530 {
                  n415 = Unbundle By Name(w1237) -> ("AIR_minus_state"=w1262:dbl, "AIR_plus_State"=w1261:dbl, "AMS_Relay_State"=w1260:dbl, "AMS_Status"=w1259:dbl, "Driver_Protection_State"=w1258:dbl, "Error_STAMP_TSAL"=w1257:dbl, "Error_value"=w1256:dbl, "HV_Acc_Menu"=w1255:dbl, "HV_Cell_OT"=w1254:dbl, "HV_Cell_OV"=w1253:dbl, "HV_Cell_UV"=w1252:dbl, "HV_DetStatus"=w1251:dbl, "HV_ECU_Heartbeat"=w1250:dbl, "HV_ECU_SC_Endline_State"=w1249:dbl, "IMD_Relay_State"=w1248:dbl, "IMD_Status"=w1247:dbl, "MCU_STAMP"=w1246:dbl, "PC_Error"=w1245:dbl, "PC_State"=w1244:dbl, "Place_of_error"=w1243:dbl, "TSAL_GREEN"=w1242:dbl, "TSAL_RED"=w1241:dbl, "TS_Over_Voltage"=w1240:dbl, "TS_Overcurrent"=w1239:dbl, "HV_DetStatus2"=w1204:dbl)
                  n416 = Index Array(array=w1238, index #1=w1262, index #2=w1261, index #3=w1260, index #4=w1259, index #5=w1258, index #6=w1257, index #7=w1256, index #8=w1255, index #9=w1254, index #10=w1253, index #11=w1252, index #12=w1251, index #13=w1250, index #14=w1249, index #15=w1248, index #16=w1247, index #17=w1246, index #18=w1245, index #19=w1244, index #20=w1243, index #21=w1242, index #22=w1241, index #23=w1240, index #24=w1239, index #25=w1204) -> (element #1=w1229:dbl, element #2=w1226:dbl, element #3=w1224:dbl, element #4=w1236:dbl, element #6=w1232:dbl, element #9=w1221:dbl, element #10=w1220:dbl, element #11=w1219:dbl, element #12=w1231:dbl, element #14=w1205:dbl, element #15=w1222:dbl, element #16=w1235:dbl, element #18=w1218:dbl, element #21=w1233:dbl, element #23=w1215:dbl, element #24=w1214:dbl, element #25=w1203:dbl)  [unwired: 8 out]
                  n417 = Equal To 0?(x=w1203) -> ()  [unwired: 1 out]
                  n418 = Not Equal To 0?(x=w1229) -> (x != 0?=→"AIR-":bool)
                  n419 = Not Equal To 0?(x=w1226) -> (x != 0?=→"AIR+":bool)
                  n420 = Not Equal To 0?(x=w1224) -> (x != 0?=→"AMS Relay":bool)
                  n421 = Equal To 0?(x=w1236) -> (x = 0?=→"AMS Error" →"AMS Error":bool)
                  n422 = Not Equal To 0?(x=w1232) -> (x != 0?=→"TSAL Error" →"TSAL Error":bool)
                  n423 = Not Equal To 0?(x=w1221) -> (x != 0?=→"OT" →"OT":bool)
                  n424 = Not Equal To 0?(x=w1220) -> (x != 0?=→"OV" →"OV":bool)
                  n425 = Not Equal To 0?(x=w1219) -> (x != 0?=→"UV" →"UV":bool)
                  n426 = Not Equal To 0?(x=w1231) -> (x != 0?=→"HVDET":bool)
                  n427 = Equal To 0?(x=w1222) -> (x = 0?=→"IMD Relay":bool)
                  n428 = Not Equal To 0?(x=w1235) -> (x != 0?=→"IMD Error" →"IMD Error":bool)
                  n429 = Not Equal To 0?(x=w1218) -> (x != 0?=→"PC Error" →"PC Error":bool)
                  n430 = Not Equal To 0?(x=w1233) -> (x != 0?=→"TSAL":bool)
                  n431 = Not Equal To 0?(x=w1215) -> (x != 0?=→"TS-OV":bool)
                  n432 = Not Equal To 0?(x=w1214) -> (x != 0?=→"TS-OC":bool)
                  n433 = Not Equal To 0?(x=w1205) -> (x != 0?=→"SC Endline":bool)
                }
                frame 532 {
                  n434 = Unbundle By Name(w1268) -> ("HV_Current"=w1270:dbl, "HV_Voltage_After_AIRs"=w1273:dbl, "HV_Voltage_Before_AIRs"=w1272:dbl, "State_of_Charge"=w1271:dbl)
                  n435 = Index Array(array=w1269, index #1=w1270, index #2=w1273, index #3=w1272, index #4=w1271) -> (element #1=w1263:dbl, element #2=w1267:dbl, element #3=→"Before":dbl, element #4=→"SoC" →"SoC [mAh]":dbl)
                  "After" <- w1267
                  "HV Current" <- w1263
                  "HV Current graph" <- w1263
                  n436 = Multiply(x=w1263, y=w1267) -> (x*y=→"HV Power out" →"HV Power out [W]":dbl)
                }
                frame 528 {
                  n437 = Unbundle By Name(w1369) -> ("HV_Cell_ID"=w1371:dbl, "HV_Cell_Temperature"=w1373:dbl, "HV_Cell_Voltage"=w1372:dbl)
                  n438 = Index Array(array=w1370, index #1=w1371, index #2=w1373, index #3=w1372) -> (element #1=w1276:dbl, element #2=w1275:dbl, element #3=w1274:dbl)
                  n439 = call "hvaccuid.vi"("ID"=w1276) -> ("Temp id"=w1278:i32, "Volt id"=w1277:i32)  [unwired: 2 in]
                  n440 = feedback #10(dbl[] [0.0, 0.0, 0.0, 0.0, 0.0, 0.0, 0.0, 0.0, 0.0, 0.0, 0.0, 0.0, 0.0, 0.0, 0.0, 0.0, 0.0, 0.0, 0.0, 0.0, 0.0, 0.0, 0.0, 0.0]) -> (w1344:dbl[])
                  "Temp 4" <- w1344
                  n441 = call "cell_temp_values.vi"("Temp In"=w1344, "lower limit"=72, "Temp"=w1275, "Temp Id"=w1278, "upper limit"=96) -> ("Temp Out"=w1345:dbl[])  [unwired: 1 in]
                  n442 = feedback-in #10(w1345) -> ()
                  n443 = feedback #11(dbl[] [0.0, 0.0, 0.0, 0.0, 0.0, 0.0, 0.0, 0.0, 0.0, 0.0, 0.0, 0.0, 0.0, 0.0, 0.0, 0.0, 0.0, 0.0, 0.0, 0.0, 0.0, 0.0, 0.0, 0.0]) -> (w1320:dbl[])
                  "Temp" <- w1320
                  n444 = call "cell_temp_values.vi"("Temp In"=w1320, "lower limit"=0, "Temp"=w1275, "Temp Id"=w1278, "upper limit"=24) -> ("Temp Out"=w1321:dbl[])  [unwired: 1 in]
                  n445 = feedback-in #11(w1321) -> ()
                  n446 = feedback #12(dbl[] [0.0, 0.0, 0.0, 0.0, 0.0, 0.0, 0.0, 0.0, 0.0, 0.0, 0.0, 0.0, 0.0, 0.0, 0.0, 0.0, 0.0, 0.0, 0.0, 0.0, 0.0, 0.0, 0.0, 0.0]) -> (w1328:dbl[])
                  "Temp 2" <- w1328
                  n447 = call "cell_temp_values.vi"("Temp In"=w1328, "lower limit"=24, "Temp"=w1275, "Temp Id"=w1278, "upper limit"=48) -> ("Temp Out"=w1329:dbl[])  [unwired: 1 in]
                  n448 = feedback-in #12(w1329) -> ()
                  n449 = feedback #13(dbl[] [0.0, 0.0, 0.0, 0.0, 0.0, 0.0, 0.0, 0.0, 0.0, 0.0, 0.0, 0.0, 0.0, 0.0, 0.0, 0.0, 0.0, 0.0, 0.0, 0.0, 0.0, 0.0, 0.0, 0.0]) -> (w1336:dbl[])
                  "Temp 3" <- w1336
                  n450 = call "cell_temp_values.vi"("Temp In"=w1336, "lower limit"=48, "Temp"=w1275, "Temp Id"=w1278, "upper limit"=72) -> ("Temp Out"=w1337:dbl[])  [unwired: 1 in]
                  n451 = feedback-in #13(w1337) -> ()
                  n452 = feedback #14(cluster{"Voltage":dbl, dbl}[] [{"Voltage"=0.0, 0.0}, {"Voltage"=0.0, 0.0}, {"Voltage"=0.0, 0.0}, {"Voltage"=0.0, 0.0}, {"Voltage"=0.0, 0.0}, {"Voltage"=0.0, 0.0}, {"Voltage"=0.0, 0.0}, {"Voltage"=0.0, 0.0}, {"Voltage"=0.0, 0.0}, {"Voltage"=0.0, 0.0}, {"Voltage"=0.0, 0.0}, {"Voltage"=0.0, 0.0}, {"Voltage"=0.0, 0.0}, {"Voltage"=0.0, 0.0}, {"Voltage"=0.0, 0.0}, {"Voltage"=0.0, 0.0}, {"Voltage"=0.0, 0.0}, {"Voltage"=0.0, 0.0}, {"Voltage"=0.0, 0.0}, {"Voltage"=0.0, 0.0}, {"Voltage"=0.0, 0.0}, {"Voltage"=0.0, 0.0}, {"Voltage"=0.0, 0.0}, {"Voltage"=0.0, 0.0}]) -> (w1340:cluster{"Voltage":dbl, dbl}[])
                  "Cell 3" <- w1340
                  n453 = call "cell_values.vi"("Voltage in"=w1340, "lower limit"=48, "Voltage"=w1274, "Voltage ID"=w1277, "upper limit"=72) -> ("Voltage Out"=w1341:cluster{"Voltage":dbl, dbl}[])  [unwired: 1 in]
                  n454 = feedback-in #14(w1341) -> ()
                  n455 = feedback #15(cluster{"Voltage":dbl, dbl}[] [{"Voltage"=0.0, 0.0}, {"Voltage"=0.0, 0.0}, {"Voltage"=0.0, 0.0}, {"Voltage"=0.0, 0.0}, {"Voltage"=0.0, 0.0}, {"Voltage"=0.0, 0.0}, {"Voltage"=0.0, 0.0}, {"Voltage"=0.0, 0.0}, {"Voltage"=0.0, 0.0}, {"Voltage"=0.0, 0.0}, {"Voltage"=0.0, 0.0}, {"Voltage"=0.0, 0.0}, {"Voltage"=0.0, 0.0}, {"Voltage"=0.0, 0.0}, {"Voltage"=0.0, 0.0}, {"Voltage"=0.0, 0.0}, {"Voltage"=0.0, 0.0}, {"Voltage"=0.0, 0.0}, {"Voltage"=0.0, 0.0}, {"Voltage"=0.0, 0.0}, {"Voltage"=0.0, 0.0}, {"Voltage"=0.0, 0.0}, {"Voltage"=0.0, 0.0}, {"Voltage"=0.0, 0.0}]) -> (w1324:cluster{"Voltage":dbl, dbl}[])
                  "Cell" <- w1324
                  n456 = call "cell_values.vi"("Voltage in"=w1324, "lower limit"=0, "Voltage"=w1274, "Voltage ID"=w1277, "upper limit"=24) -> ("Voltage Out"=w1325:cluster{"Voltage":dbl, dbl}[])  [unwired: 1 in]
                  n457 = feedback-in #15(w1325) -> ()
                  n458 = feedback #16(cluster{"Voltage":dbl, dbl}[] [{"Voltage"=0.0, 0.0}, {"Voltage"=0.0, 0.0}, {"Voltage"=0.0, 0.0}, {"Voltage"=0.0, 0.0}, {"Voltage"=0.0, 0.0}, {"Voltage"=0.0, 0.0}, {"Voltage"=0.0, 0.0}, {"Voltage"=0.0, 0.0}, {"Voltage"=0.0, 0.0}, {"Voltage"=0.0, 0.0}, {"Voltage"=0.0, 0.0}, {"Voltage"=0.0, 0.0}, {"Voltage"=0.0, 0.0}, {"Voltage"=0.0, 0.0}, {"Voltage"=0.0, 0.0}, {"Voltage"=0.0, 0.0}, {"Voltage"=0.0, 0.0}, {"Voltage"=0.0, 0.0}, {"Voltage"=0.0, 0.0}, {"Voltage"=0.0, 0.0}, {"Voltage"=0.0, 0.0}, {"Voltage"=0.0, 0.0}, {"Voltage"=0.0, 0.0}, {"Voltage"=0.0, 0.0}]) -> (w1332:cluster{"Voltage":dbl, dbl}[])
                  "Cell 2" <- w1332
                  n459 = call "cell_values.vi"("Voltage in"=w1332, "lower limit"=24, "Voltage"=w1274, "Voltage ID"=w1277, "upper limit"=48) -> ("Voltage Out"=w1333:cluster{"Voltage":dbl, dbl}[])  [unwired: 1 in]
                  n460 = feedback-in #16(w1333) -> ()
                  n461 = feedback #17(dbl[] [0.0, 0.0, 0.0, 0.0, 0.0, 0.0, 0.0, 0.0, 0.0, 0.0, 0.0, 0.0, 0.0, 0.0, 0.0, 0.0, 0.0, 0.0, 0.0, 0.0, 0.0, 0.0, 0.0, 0.0]) -> (w1285:dbl[])
                  "Temp 8" <- w1285
                  n462 = call "cell_temp_values.vi"("Temp In"=w1285, "lower limit"=168, "Temp"=w1275, "Temp Id"=w1278, "upper limit"=192) -> ("Temp Out"=w1310:dbl[])  [unwired: 1 in]
                  n463 = feedback-in #17(w1310) -> ()
                  n464 = feedback #18(dbl[] [0.0, 0.0, 0.0, 0.0, 0.0, 0.0, 0.0, 0.0, 0.0, 0.0, 0.0, 0.0, 0.0, 0.0, 0.0, 0.0, 0.0, 0.0, 0.0, 0.0, 0.0, 0.0, 0.0, 0.0]) -> (w1291:dbl[])
                  "Temp 5" <- w1291
                  n465 = call "cell_temp_values.vi"("Temp In"=w1291, "lower limit"=96, "Temp"=w1275, "Temp Id"=w1278, "upper limit"=120) -> ("Temp Out"=w1292:dbl[])  [unwired: 1 in]
                  n466 = feedback-in #18(w1292) -> ()
                  n467 = feedback #19(dbl[] [0.0, 0.0, 0.0, 0.0, 0.0, 0.0, 0.0, 0.0, 0.0, 0.0, 0.0, 0.0, 0.0, 0.0, 0.0, 0.0, 0.0, 0.0, 0.0, 0.0, 0.0, 0.0, 0.0, 0.0]) -> (w1289:dbl[])
                  "Temp 6" <- w1289
                  n468 = call "cell_temp_values.vi"("Temp In"=w1289, "lower limit"=120, "Temp"=w1275, "Temp Id"=w1278, "upper limit"=144) -> ("Temp Out"=w1298:dbl[])  [unwired: 1 in]
                  n469 = feedback-in #19(w1298) -> ()
                  n470 = feedback #20(dbl[] [0.0, 0.0, 0.0, 0.0, 0.0, 0.0, 0.0, 0.0, 0.0, 0.0, 0.0, 0.0, 0.0, 0.0, 0.0, 0.0, 0.0, 0.0, 0.0, 0.0, 0.0, 0.0, 0.0, 0.0]) -> (w1287:dbl[])
                  "Temp 7" <- w1287
                  n471 = call "cell_temp_values.vi"("Temp In"=w1287, "lower limit"=144, "Temp"=w1275, "Temp Id"=w1278, "upper limit"=168) -> ("Temp Out"=w1304:dbl[])  [unwired: 1 in]
                  n472 = feedback-in #20(w1304) -> ()
                  n473 = feedback #21(cluster{"Voltage":dbl, dbl}[] [{"Voltage"=0.0, 0.0}, {"Voltage"=0.0, 0.0}, {"Voltage"=0.0, 0.0}, {"Voltage"=0.0, 0.0}, {"Voltage"=0.0, 0.0}, {"Voltage"=0.0, 0.0}, {"Voltage"=0.0, 0.0}, {"Voltage"=0.0, 0.0}, {"Voltage"=0.0, 0.0}, {"Voltage"=0.0, 0.0}, {"Voltage"=0.0, 0.0}, {"Voltage"=0.0, 0.0}, {"Voltage"=0.0, 0.0}, {"Voltage"=0.0, 0.0}, {"Voltage"=0.0, 0.0}, {"Voltage"=0.0, 0.0}, {"Voltage"=0.0, 0.0}, {"Voltage"=0.0, 0.0}, {"Voltage"=0.0, 0.0}, {"Voltage"=0.0, 0.0}, {"Voltage"=0.0, 0.0}, {"Voltage"=0.0, 0.0}, {"Voltage"=0.0, 0.0}, {"Voltage"=0.0, 0.0}]) -> (w1286:cluster{"Voltage":dbl, dbl}[])
                  "Cell 6" <- w1286
                  n474 = call "cell_values.vi"("Voltage in"=w1286, "lower limit"=144, "Voltage"=w1274, "Voltage ID"=w1277, "upper limit"=168) -> ("Voltage Out"=w1307:cluster{"Voltage":dbl, dbl}[])  [unwired: 1 in]
                  n475 = feedback-in #21(w1307) -> ()
                  n476 = feedback #22(cluster{"Voltage":dbl, dbl}[] [{"Voltage"=0.0, 0.0}, {"Voltage"=0.0, 0.0}, {"Voltage"=0.0, 0.0}, {"Voltage"=0.0, 0.0}, {"Voltage"=0.0, 0.0}, {"Voltage"=0.0, 0.0}, {"Voltage"=0.0, 0.0}, {"Voltage"=0.0, 0.0}, {"Voltage"=0.0, 0.0}, {"Voltage"=0.0, 0.0}, {"Voltage"=0.0, 0.0}, {"Voltage"=0.0, 0.0}, {"Voltage"=0.0, 0.0}, {"Voltage"=0.0, 0.0}, {"Voltage"=0.0, 0.0}, {"Voltage"=0.0, 0.0}, {"Voltage"=0.0, 0.0}, {"Voltage"=0.0, 0.0}, {"Voltage"=0.0, 0.0}, {"Voltage"=0.0, 0.0}, {"Voltage"=0.0, 0.0}, {"Voltage"=0.0, 0.0}, {"Voltage"=0.0, 0.0}, {"Voltage"=0.0, 0.0}]) -> (w1290:cluster{"Voltage":dbl, dbl}[])
                  "Cell 4" <- w1290
                  n477 = call "cell_values.vi"("Voltage in"=w1290, "lower limit"=96, "Voltage"=w1274, "Voltage ID"=w1277, "upper limit"=120) -> ("Voltage Out"=w1295:cluster{"Voltage":dbl, dbl}[])  [unwired: 1 in]
                  n478 = feedback-in #22(w1295) -> ()
                  n479 = feedback #23(cluster{"Voltage":dbl, dbl}[] [{"Voltage"=0.0, 0.0}, {"Voltage"=0.0, 0.0}, {"Voltage"=0.0, 0.0}, {"Voltage"=0.0, 0.0}, {"Voltage"=0.0, 0.0}, {"Voltage"=0.0, 0.0}, {"Voltage"=0.0, 0.0}, {"Voltage"=0.0, 0.0}, {"Voltage"=0.0, 0.0}, {"Voltage"=0.0, 0.0}, {"Voltage"=0.0, 0.0}, {"Voltage"=0.0, 0.0}, {"Voltage"=0.0, 0.0}, {"Voltage"=0.0, 0.0}, {"Voltage"=0.0, 0.0}, {"Voltage"=0.0, 0.0}, {"Voltage"=0.0, 0.0}, {"Voltage"=0.0, 0.0}, {"Voltage"=0.0, 0.0}, {"Voltage"=0.0, 0.0}, {"Voltage"=0.0, 0.0}, {"Voltage"=0.0, 0.0}, {"Voltage"=0.0, 0.0}, {"Voltage"=0.0, 0.0}]) -> (w1288:cluster{"Voltage":dbl, dbl}[])
                  "Cell 5" <- w1288
                  n480 = call "cell_values.vi"("Voltage in"=w1288, "lower limit"=120, "Voltage"=w1274, "Voltage ID"=w1277, "upper limit"=144) -> ("Voltage Out"=w1301:cluster{"Voltage":dbl, dbl}[])  [unwired: 1 in]
                  n481 = feedback-in #23(w1301) -> ()
                  n482 = Build Array (concatenate)(w1324, w1332, w1340, w1290, w1288, w1286) -> (w1359:cluster{"Voltage":dbl, dbl}[])
                  n483 = Build Array (concatenate)(w1320, w1328, w1336, w1344, w1291, w1289, w1287, w1285) -> (w1279:dbl[])
                  n484 = Array Max & Min(array=w1359) -> (max value=w1358:cluster{"Voltage":dbl, dbl}, min value=w1357:cluster{"Voltage":dbl, dbl})  [unwired: 2 out]
                  n485 = Array Max & Min(array=w1279) -> (max value=w1282:dbl)  [unwired: 3 out]
                  "Max Temp Calc" <- w1282
                  n486 = Unbundle(w1358) -> ("Voltage"=w1280:dbl)  [unwired: 1 out]
                  "Max Voltage" <- w1280
                  n487 = Unbundle(w1357) -> ("Voltage"=w1281:dbl)  [unwired: 1 out]
                  "Min Voltage Calc" <- w1281
                  n488 = case shown="True" "OK Button" {
                    tunnel: w1279 -> [_ w1377]
                    tunnel: [_ w1374] -> w1284
                    frame False {
                    }
                    frame True {
                      n489 = call "heatmap.vi"("Ranges"="Ranges", "Colorset"="Colors", "Temp 1D"=w1377) -> ("2D Heatmap"=w1374:u32[][])
                    }
                  }
                  "Heatmap" <- w1284
                  n490 = Greater?(x=w1280, y="Alert Max [xV]") -> (0:w1353:bool)
                  n491 = Less?(x=w1281, y="Alert Min [xV]") -> (x < y?=w1354:bool)
                  n492 = Or(x=w1353, y=w1354) -> (x .or. y?=w1352:bool)
                  n493 = Greater?(x=w1282, y="Alert Max [xC]") -> (0:w1348:bool)
                  n494 = And(x=w1352, y="HV V Alert") -> (x .and. y?=→"HV Volt Alert":bool)
                  n495 = And(x=w1348, y="HV T Alert") -> (x .and. y?=→"HV Temp Alert":bool)
                }
                frame 787 {
                  n496 = Unbundle By Name(w1380) -> ("Critical_cell_values_heartbeat"=w1382:dbl, "HV_Cell_Temp_MAX"=w1384:dbl, "HV_Cell_Voltage_MIN"=w1383:dbl)
                  n497 = Index Array(array=w1381, index #1=w1382, index #2=w1384, index #3=w1383) -> (element #2=→"Max Temp" →"Max Temp":dbl, element #3=→"Min Voltage" →"Min Voltage":dbl)  [unwired: 1 out]
                }
                frame 393 {
                  n498 = Unbundle By Name(w1401) -> ("AMK3_DC_On"=w1403:dbl, "AMK3_Target_Velocity"=w1406:dbl, "AMK3_TorqueLimitNegative"=w1405:dbl, "AMK3_TorqueLimitPositive"=w1404:dbl, "AMK3_Enable"=w1400:dbl, "AMK3_Error_Reset"=w1399:dbl, "AMK3_Inverter_On"=w1398:dbl)
                  n499 = Index Array(array=w1402, index #1=w1403, index #2=w1406, index #3=w1405, index #4=w1404, index #5=w1400, index #6=w1399, index #7=w1398) -> (element #1=w1396:dbl, element #2=→"RL Target Velocity":dbl, element #3=w1386:dbl, element #4=w1387:dbl, element #5=w1392:dbl, element #6=w1391:dbl, element #7=w1390:dbl)
                  "RL Torque Limit +" <- w1387
                  "RL Torque Limit -" <- w1386
                  n500 = Not Equal To 0?(x=w1392) -> (x != 0?=→"RL Enable":bool)
                  n501 = Not Equal To 0?(x=w1390) -> (x != 0?=→"RL Inverter On":bool)
                  n502 = Not Equal To 0?(x=w1391) -> (x != 0?=→"RL Error Reset":bool)
                  n503 = Equal To 0?(x=w1387) -> (x = 0?=w1388:bool)
                  n504 = case shown="True" w1388 {
                    tunnel: w1386 -> [_ w1408]
                    tunnel: [w1407 w1408] -> w1385
                    tunnel: w1387 -> [w1407 _]
                    frame False {
                    }
                    frame True {
                    }
                  }
                  "RL Torque Limit" <- w1385
                  n505 = Not Equal To 0?(x=w1396) -> (x != 0?=→"RL DC On":bool)
                }
                frame 394 {
                  n506 = Unbundle By Name(w1425) -> ("AMK4_DC_On"=w1427:dbl, "AMK4_Target_Velocity"=w1430:dbl, "AMK4_TorqueLimitNegative"=w1429:dbl, "AMK4_TorqueLimitPositive"=w1428:dbl, "AMK4_Enable"=w1424:dbl, "AMK4_Error_Reset"=w1423:dbl, "AMK4_Inverter_On"=w1422:dbl)
                  n507 = Index Array(array=w1426, index #1=w1427, index #2=w1430, index #3=w1429, index #4=w1428, index #5=w1424, index #6=w1423, index #7=w1422) -> (element #1=w1414:dbl, element #2=→"RR Target Velocity":dbl, element #3=w1410:dbl, element #4=w1411:dbl, element #5=w1418:dbl, element #6=w1417:dbl, element #7=w1416:dbl)
                  "RR Torque Limit +" <- w1411
                  "RR Torque Limit -" <- w1410
                  n508 = Not Equal To 0?(x=w1418) -> (x != 0?=→"RR Enable":bool)
                  n509 = Not Equal To 0?(x=w1416) -> (x != 0?=→"RR Inverter On":bool)
                  n510 = Not Equal To 0?(x=w1417) -> (x != 0?=→"RR Error Reset":bool)
                  n511 = Equal To 0?(x=w1411) -> (x = 0?=w1412:bool)
                  n512 = Not Equal To 0?(x=w1414) -> (x != 0?=→"RR DC On":bool)
                  n513 = case shown="True" w1412 {
                    tunnel: w1410 -> [_ w1432]
                    tunnel: [w1431 w1432] -> w1409
                    tunnel: w1411 -> [w1431 _]
                    frame False {
                    }
                    frame True {
                    }
                  }
                  "RR Torque Limit" <- w1409
                }
                frame 401 {
                  n514 = Unbundle By Name(w1436) -> ("RES_GO_Signal"=w1437:dbl)
                  n515 = Index Array(array=w1435, index=w1437) -> (element=w1434:dbl)
                  n516 = Not Equal To 0?(x=w1434) -> (x != 0?=→"RES GO":bool)
                }
                frame 529 {
                  n517 = Unbundle By Name(w1447) -> ("Charger_SC_Ready"=w1445:dbl, "EPOS_Position_actual_value"=w1444:dbl, "Vectornav_yaw_rate_rear_value"=w1443:dbl, "EBS_RELAY_FB"=w1442:dbl, "HV_DetStatus2"=w1441:dbl, "BFS_Offset"=w1440:dbl, "EPOS_Torque_actual_value"=w1439:dbl, "EPOS_Statusword"=w1438:dbl)
                  n518 = Index Array(array=w1446, index #1=w1445, index #2=w1444, index #3=w1443, index #4=w1442, index #5=w1441, index #6=w1440, index #7=w1439, index #8=w1438) -> ()  [unwired: 8 out]
                }
                frame 1385 {
                  n519 = Unbundle By Name(w1451) -> ("Charger_State"=w1450:dbl)
                  n520 = Index Array(array=w1449, index=w1450) -> (element=w1448:dbl)
                  n521 = Index Array(array=string[] ["nothing", "Init", "Ready", "Manual", "Autocharge", "Comm. error", "Error"], index=w1448) -> (element=→"Charging State":string)
                }
                frame 912 {
                  n522 = Unbundle By Name(w1468) -> ("NPDBCounter"=w1463:dbl, "BDCDCUmbilicalOn"=w1464:dbl, "BDCDCRegenerationOn"=w1465:dbl, "BDCDCOutput2Requested"=w1466:dbl, "BDCDCOutput1Requested"=w1467:dbl)
                  n523 = Index Array(array=w1462, index #1=w1463, index #2=w1464, index #3=w1465, index #4=w1466, index #5=w1467) -> (element #2=w1461:dbl, element #3=w1460:dbl, element #4=w1459:dbl, element #5=w1458:dbl)  [unwired: 1 out]
                  n524 = Not Equal To 0?(x=w1461) -> (x != 0?=→"Umbilical On":bool)
                  n525 = Not Equal To 0?(x=w1460) -> (x != 0?=→"Regen On":bool)
                  n526 = Not Equal To 0?(x=w1459) -> (x != 0?=→"CH2 Requested":bool)
                  n527 = Not Equal To 0?(x=w1458) -> (x != 0?=→"CH1 Requested":bool)
                }
                frame 913 {
                  n528 = Unbundle By Name(w1483) -> ("VDCDCLV2Setpoint"=w1482:dbl, "VDCDCLV1Setpoint"=w1481:dbl, "VDCDCHVSetpoint"=w1480:dbl, "NDCDCMultiplexer"=w1479:dbl, "IDCDCLV2Limit"=w1478:dbl, "IDCDCHVLimit"=w1477:dbl, "IDCDCLV1Limit"=w1476:dbl)
                  n529 = Index Array(array=w1475, index #1=w1482, index #2=w1481, index #3=w1480, index #4=w1479, index #5=w1478, index #6=w1477, index #7=w1476) -> (element #1=→"CH2 Voltage Setpoint":dbl, element #2=→"CH1 Voltage Setpoint":dbl, element #3=→"HV Voltage Setpoint":dbl, element #5=→"CH2 Current Limit":dbl, element #6=→"HV Current Limit":dbl, element #7=→"CH1 Current Limit":dbl)  [unwired: 1 out]
                }
                frame 914 {
                  n530 = Unbundle By Name(w1533) -> ("BDCDCAuxIsoEnabled"=w1532:dbl, "BDCDCBB1OtpError"=w1531:dbl, "BDCDCBB2OtpError"=w1530:dbl, "BDCDCBB3OtpError"=w1529:dbl, "BDCDCCANError"=w1528:dbl, "BDCDCHVError"=w1527:dbl, "BDCDCHVOcpError"=w1526:dbl, "BDCDCLVOvpInError"=w1525:dbl, "BDCDCLVUvpAlimAuxError"=w1524:dbl, "BDCDCLVUvpInError"=w1501:dbl, "BDCDCOutput1Demanded"=w1523:dbl, "BDCDCOutput1OvpError"=w1522:dbl, "BDCDCOutput1Warning"=w1521:dbl, "BDCDCOutput2Demanded"=w1520:dbl, "BDCDCOutput2OvpError"=w1519:dbl, "BDCDCOutput2Warning"=w1518:dbl, "BDCDCRegenerationDemanded"=w1517:dbl, "BDCDCSR1OtpError"=w1516:dbl, "BDCDCSR2OtpError"=w1515:dbl, "BDCDCUmbilicalDemanded"=w1514:dbl, "BDCDCWakeUp"=w1513:dbl, "NDCDCState"=w1512:dbl)
                  n531 = Index Array(array=w1511, index #1=w1532, index #2=w1531, index #3=w1530, index #4=w1529, index #5=w1528, index #6=w1527, index #7=w1526, index #8=w1525, index #9=w1524, index #10=w1501, index #11=w1523, index #12=w1522, index #13=w1521, index #14=w1520, index #15=w1519, index #16=w1518, index #17=w1517, index #18=w1516, index #19=w1515, index #20=w1514, index #21=w1513, index #22=w1512) -> (element #2=w1510:dbl, element #3=w1509:dbl, element #4=w1508:dbl, element #5=w1507:dbl, element #6=w1506:dbl, element #7=w1505:dbl, element #8=w1504:dbl, element #9=w1503:dbl, element #10=w1502:dbl, element #12=w1500:dbl, element #15=w1499:dbl, element #18=w1498:dbl, element #19=w1497:dbl)  [unwired: 9 out]
                  n532 = Not Equal To 0?(x=w1510) -> (x != 0?=→"BB1OtpError" →"BB1OtpError":bool)
                  n533 = Not Equal To 0?(x=w1509) -> (x != 0?=→"BB2OtpError" →"BB2OtpError":bool)
                  n534 = Not Equal To 0?(x=w1508) -> (x != 0?=→"BB3OtpError" →"BB3OtpError":bool)
                  n535 = Not Equal To 0?(x=w1507) -> (x != 0?=→"CANError" →"CANError":bool)
                  n536 = Not Equal To 0?(x=w1506) -> (x != 0?=→"HVError" →"HVError":bool)
                  n537 = Not Equal To 0?(x=w1505) -> (x != 0?=→"HVOcpError" →"HVOcpError":bool)
                  n538 = Not Equal To 0?(x=w1504) -> (x != 0?=→"LVOvpInError" →"LVOvpInError":bool)
                  n539 = Not Equal To 0?(x=w1503) -> (x != 0?=→"LVUvpAlimAuxError" →"LVUvpAlimAuxError":bool)
                  n540 = Not Equal To 0?(x=w1502) -> (x != 0?=→"LVUvpInError" →"LVUvpInError":bool)
                  n541 = Not Equal To 0?(x=w1500) -> (x != 0?=→"Output1OvpError" →"Output1OvpError":bool)
                  n542 = Not Equal To 0?(x=w1499) -> (x != 0?=→"Output2OvpError" →"Output2OvpError":bool)
                  n543 = Not Equal To 0?(x=w1498) -> (x != 0?=→"CSR1OtpError" →"CSR1OtpError":bool)
                  n544 = Not Equal To 0?(x=w1497) -> (x != 0?=→"CSR2OtpError" →"CSR2OtpError":bool)
                }
                frame 915 {
                  n545 = Unbundle By Name(w1574) -> ("NDCDCChecksum"=w1572:dbl, "NDCDCApplicationId"=w1571:dbl, "Multiplexer"=w1570:dbl, "IDCDCOutput1UnBalance"=w1569:dbl, "IDCDCHVInAverage"=w1568:dbl, "BDCDCFlashSubzoneError"=w1567:dbl, "NDCDCBootloaderId"=w1566:dbl, "TDCDCBB2Measured"=w1565:dbl, "TDCDCBB1Measured"=w1564:dbl, "NDCDCXcpFaults"=w1563:dbl, "NDCDCSerial"=w1562:dbl, "NDCDCRcpWarning"=w1561:dbl, "NDCDCOutputOverload2Count"=w1560:dbl, "NDCDCOutputOverload1Count"=w1559:dbl, "TDCDCBB3Measured"=w1558:dbl, "TDCDCSR2Measured"=w1557:dbl, "TDCDCSR1Measured"=w1556:dbl, "VDCDCHVInAverage"=w1555:dbl, "VDCDCAux5Measured"=w1554:dbl, "VDCDCAux4Measured"=w1553:dbl, "VDCDCAux3Measured"=w1552:dbl, "VDCDCAux2Measured"=w1551:dbl, "VDCDCAux1Measured"=w1550:dbl, "VDCDCLVInMin"=w1549:dbl, "VDCDCLVInMax"=w1548:dbl, "VDCDCLVInAverage"=w1547:dbl)
                  n546 = Index Array(array=w1573, index #1=w1572, index #2=w1571, index #3=w1570, index #4=w1569, index #5=w1568, index #6=w1567, index #7=w1566, index #8=w1565, index #9=w1564, index #10=w1563, index #11=w1562, index #12=w1561, index #13=w1560, index #14=w1559, index #15=w1558, index #16=w1557, index #17=w1556, index #18=w1555, index #19=w1554, index #20=w1553, index #21=w1552, index #22=w1551, index #23=w1550, index #24=w1549, index #25=w1548, index #26=w1547) -> (element #4=→"Current IO Unbalance":dbl, element #5=→"HV Current In":dbl, element #6=w1546:dbl, element #8=→"Temp BB2":dbl, element #9=→"Temp BB1":dbl, element #13=w1541:dbl, element #14=w1540:dbl, element #15=→"Temp BB3":dbl, element #16=→"Temp SR2":dbl, element #17=→"Temp SR1":dbl, element #18=→"HV Voltage In":dbl)  [unwired: 15 out]
                  n547 = Not Equal To 0?(x=w1546) -> (x != 0?=→"FlashSubzoneError" →"FlashSubzoneError":bool)
                  n548 = Add(x=w1541, y=w1540) -> (x+y=→"Output Overload Count":dbl)
                }
                frame 916 {
                  # "mAh2"
                  # "mAh1"
                  # "V2"
                  # "V1"
                  # "s"
                  # "h"
                  # "ms"
                  # "W2"
                  # "W1"
                  # "mWh2"
                  # "mWh1"
                  n549 = Unbundle By Name(w1611) -> ("VDCDCOutput1Max"=w1610:dbl, "VDCDCOutput1Min"=w1609:dbl, "VDCDCOutput1Average"=w1608:dbl, "IDCDCOutput1Min"=w1607:dbl, "IDCDCOutput1Max"=w1606:dbl, "IDCDCOutput1Average"=w1605:dbl, "VDCDCOutput2Average"=w1603:dbl, "IDCDCOutput2Average"=w1602:dbl)
                  n550 = Index Array(array=w1604, index #1=w1610, index #2=w1609, index #3=w1608, index #4=w1607, index #5=w1606, index #6=w1605, index #7=w1603, index #8=w1602) -> (element #1=→"Voltage Out Max 1":dbl, element #2=→"Voltage Out Min 1":dbl, element #3=w1579:dbl, element #4=→"Current Out Min 1":dbl, element #5=→"Current Out Max 1":dbl, element #6=w1598:dbl, element #7=w1580:dbl, element #8=w1597:dbl)
                  n551 = call "timeelapsed.vi"() -> ("validity"=w1575:bool, "dt"=w1587:u32)  [unwired: 2 in]
                  n552 = Divide(x=w1587, y=1000) -> (x/y=w1585:dbl)
                  n553 = Bundle("Data"=w1579, "Data"=w1580) -> (→"Channel voltages":cluster{"Data":dbl, "Data":dbl})  [unwired: 1 in]
                  n554 = Bundle("Data"=w1598, "Data"=w1597) -> (→"Channel currents":cluster{"Data":dbl, "Data":dbl})  [unwired: 1 in]
                  n555 = Multiply(x=w1598, y=w1579) -> (x*y=w1591:dbl)
                  n556 = Multiply(x=w1597, y=w1580) -> (x*y=w1590:dbl)
                  n557 = Divide(x=w1585, y=3600.0) -> (x/y=w1583:dbl)
                  n558 = Multiply(x=w1591, y=w1583) -> (x*y=w1589:dbl)
                  n559 = Multiply(x=w1590, y=w1583) -> (x*y=w1588:dbl)
                  n560 = Divide(x=w1589, y=w1579) -> (x/y=w1582:dbl)
                  n561 = Divide(x=w1588, y=w1580) -> (x/y=w1581:dbl)
                  n562 = Bundle(w1591, w1590) -> (→"Channel powers":cluster{dbl, dbl})  [unwired: 1 in]
                  n563 = Add(x=w1582, y=w1581) -> (x+y=w1576:dbl)
                  n564 = feedback #24(0.0) -> (w1578:dbl)
                  n565 = case shown="True" w1575 {
                    tunnel: w1578 -> [w1612 w1615]
                    tunnel: [w1612 w1613] -> w1577
                    tunnel: w1576 -> [_ w1614]
                    frame False {
                    }
                    frame True {
                      n566 = Add(x=w1615, y=w1614) -> (x+y=w1613:dbl)
                    }
                  }
                  "LV mAh" <- w1577
                  n567 = feedback-in #24(w1577) -> ()
                }
                frame 917 {
                  n568 = Unbundle By Name(w1627) -> ("VDCDCOutput2Min"=w1626:dbl, "VDCDCOutput2Max"=w1625:dbl, "VDCDCOutput2Average"=w1624:dbl, "IDCDCOutput2Min"=w1623:dbl, "IDCDCOutput2Max"=w1622:dbl, "IDCDCOutput2Average"=w1621:dbl)
                  n569 = Index Array(array=w1620, index #1=w1626, index #2=w1625, index #3=w1624, index #4=w1623, index #5=w1622, index #6=w1621) -> (element #1=→"Voltage Out Min 2":dbl, element #2=→"Voltage Out Max 2":dbl, element #4=→"Current Out Min 2":dbl, element #5=→"Current Out Max 2":dbl)  [unwired: 2 out]
                }
                frame 624 {
                  n570 = Unbundle By Name(w1631) -> ("Vectornav_yaw_rate_rear_value"=w1629:dbl)
                  n571 = Index Array(array=w1630, index=w1629) -> (element=→"Yaw Rear Vectornav":dbl)
                }
              }
            }
          }
        }
      }
      frame #2 {
        n572 = Tick Count (ms)() -> (millisecond timer value=w1674:u32)
        n573 = Subtract(x=w1674, y=w1673) -> (x-y=→"Actual Timestep":u32)
        n574 = case shown="True" "Lapdata disp" {
          frame False {
          }
          frame True {
            n575 = local read "Temp Motor FL"() -> (w1693:dbl)
            n576 = local read "Temp Motor FR"() -> (w1692:dbl)
            n577 = local read "Temp Motor RL"() -> (w1691:dbl)
            n578 = local read "Temp Motor RR"() -> (w1690:dbl)
            n579 = local read "Max Temp Calc"() -> (w1679:dbl)
            n580 = local read "Temp inv FL"() -> (w1689:dbl)
            n581 = local read "Temp inv FR"() -> (w1688:dbl)
            n582 = local read "Temp inv RL"() -> (w1687:dbl)
            n583 = local read "Temp inv RR"() -> (w1686:dbl)
            n584 = local read "HV Current"() -> (w1680:dbl)
            n585 = local read "SoC [mAh]"() -> (w1678:dbl)
            n586 = Build Array(w1679, w1678) -> (w1677:dbl[])
            n587 = Build Array(w1689, w1688, w1687, w1686) -> (w1685:dbl[])
            n588 = Build Array(w1693, w1692, w1691, w1690) -> (w1694:dbl[])
            n589 = call "lapdata_new.vi"("Reset"="Reset", "Laptrigger"="Laptrigger", "InverterTemps"=w1685, "MotorTemps"=w1694, "Current"=w1680, "Hv Data"=w1677) -> ("Inverter Temp"=→"Inverter Temp":cluster{i32[], dbl[]}[], "Motor Temp"=→"Motor Temp":cluster{i32[], dbl[]}[], "HV Temps"=w1676:dbl[], "Lap                    Laptime                        SoC                 Current Avg |                             Motor Temperatures                          |                               Inverter Temperatures"=w1682:T6)  [unwired: 2 in]
            "Lap                    Laptime                        SoC                 Current Avg |                             Motor Temperatures                            |                            Inverter Temperatures" <- w1682
            n590 = case shown="True" "Export" {
              tunnel: w1682 -> [_ w1702]
              tunnel: w1676 -> [_ w1697]
              frame False {
              }
              frame True {
                n591 = Current VI's Path() -> (path=w1700:path)
                n592 = Build Path(base path=w1700, name or relative path="..\\..\\Runsheet 2022_template.xlsx" ("relative path")) -> (appended path=w1698:path)
                n593 = Copy(9:TRUE ("overwrite (F)"), 11:w1698) -> (0:w1705:errorcluster, 3:w1703:path)  [unwired: 3 in, 1 out]
                n594 = call <vilib>:"Clear Errors.vi"("error in (no error)"=w1705) -> ()  [unwired: 5 in, 2 out]
                n595 = Path To String(path=w1703) -> (string=w1704:string)
                n596 = call "Runsheet.vi"("HV Temps"=w1697, "Data"=w1702, "Path"=w1704) -> ()  [unwired: 1 in]
              }
            }
          }
        }
      }
    }
  }
  n597 = Equal?(x=u16 4, y="Data source") -> (x = y?=w1:bool)
  n598 = case shown="True" w1 {
    frame False {
    }
    frame True {
      n599 = call-poly "VISA Configure Serial Port"("VISA resource name"="Port", "timeout (10sec)"="timeout ms", "termination char\n(0xA = '\\n' = LF)"="termination char\n(0xA = '\\n' = LF)", "Enable Termination\nChar (T)"="Enable Termination\nChar", "baud rate (9600)"="baud", "data bits (8)"="data bits", "parity (0:none)"="parity", "stop bits (10: 1 bit)"="stop bits", "flow control (0:none)"="flow control") -> ("VISA resource name out"=w1706:refnum<visa-resource-name>, "error out"=w1711:errorcluster)  [unwired: 5 in]
      "serial error" <- w1711
      n600 = call <vilib>:"Clear Errors.vi"("error in (no error)"=w1711) -> ()  [unwired: 5 in, 2 out]
      n601 = while {
        tunnel: "max buffer size" -> [w1750]
        tunnel: w1706 -> [w1748]
        stop <- FALSE stop-if-true
        w1739 = 10 ("y")
        n602 = VISA Read(VISA resource name=w1748, byte count=w1750) -> (read buffer=w1746:string, error out=w1749:errorcluster)  [unwired: 1 in, 2 out]
        "buffer" <- w1746
        n603 = call <vilib>:"Clear Errors.vi"("error in (no error)"=w1749) -> ()  [unwired: 5 in, 2 out]
        n604 = String To Byte Array(string=w1746) -> (unsigned byte array=w1735:u8[])
        n605 = Array Size(array=w1735) -> (size(s)=w1745:i32)
        n606 = while {
          tunnel: w1735 -> [w1764] mode=indexing
          tunnel: w1745 -> [w1763]
          tunnel: [w1760] -> w1742
          tunnel: w1735 -> [w1757]
          i -> [w1760]
          stop <- w1751 stop-if-true
          n607 = Add(x=3, y=w1760) -> (x+y=w1758:i32)
          n608 = Equal?(x=w1763, y=w1760) -> (x = y?=w1762:bool)
          n609 = Equal?(x=w1764, y=u8 126) -> (x = y?=w1753:bool)
          n610 = Index Array(array=w1757, index=w1758) -> (element=w1756:u8)
          n611 = Equal?(x=w1756, y=u8 129) -> (x = y?=w1754:bool)
          n612 = And(x=w1754, y=w1753) -> (x .and. y?=w1752:bool)
          n613 = Or(x=w1752, y=w1762) -> (x .or. y?=w1751:bool)
        }
        n614 = Delete From Array(array=w1735, length=w1742, index=0) -> (array with subset deleted=w1736:u8[])  [unwired: 1 out]
        n615 = Delete From Array(array=w1736, length=8, index=0) -> (deleted portion=w1722:u8[], array with subset deleted=w1737:u8[])
        "deleted portion 2" <- w1722
        n616 = Index Array(array=w1722, index=6) -> (element=w1720:u8)
        n617 = Index Array(array=w1722, index #1=1 ("index"), index #2=2 ("length")) -> (element #1=w1731:u8, element #2=w1728:u8)
        n618 = Multiply(x=w1720, y=i16 -1) -> (x*y=→"RSSI [dBm]" →"RSSI [dBm]":i16)
        n619 = Multiply(x=u8 255, y=w1731) -> (x*y=w1729:u8)
        n620 = Add(x=w1729, y=w1728) -> (x+y=w1726:u8)
        n621 = Subtract(x=w1726, y=u8 5) -> (x-y=w1725:u8)
        "x-y" <- w1725
        n622 = Delete From Array(array=w1737, length=w1725, index=0 ("length")) -> (deleted portion=w1723:u8[])  [unwired: 1 out]
        n623 = Array Size(array=w1723) -> (size(s)=w1741:i32)
        n624 = Divide(x=w1741, y=w1739) -> (x/y=w1740:dbl)
        n625 = Reshape Array(w1723, w1740, w1739) -> (→"serial in 2":u8[][])
      }
    }
  }
  n626 = while {
    stop <- FALSE stop-if-true
    # "HV Temp Alert 1\nHV Volt Alert 2"
    n627 = local read "HV Temp Alert"() -> (w1768:bool)
    n628 = local read "HV Volt Alert"() -> (w1767:bool)
    n629 = Wait Until Next ms Multiple(millisecond multiple=u32 50) -> ()  [unwired: 1 out]
    n630 = Build Array(w1768, w1767) -> (w1766:bool[])
    n631 = Or(x=w1768, y=w1767) -> (x .or. y?=w1769:bool)
    n632 = Boolean Array To Number(Boolean array=w1766) -> (number=w1765:u32)
    n633 = case shown="True" w1769 {
      selector: w1769 -> [_ w1773]
      tunnel: w1765 -> [_ w1772]
      frame False {
      }
      frame True {
        n634 = case shown="1" w1772 {
          tunnel: w1773 -> [w1775 w1777 w1779]
          frame 0, Default {
            n635 = call "alert_new.vi"("Path"=path "alert_sound.wav", "Turn on"=w1775) -> ()  [unwired: 2 in, 1 out]
          }
          frame 1 {
            n636 = call "alert_new.vi"("Path"=path "alert_sound.wav", "Turn on"=w1777) -> ()  [unwired: 2 in, 1 out]
          }
          frame 2 {
            n637 = call "alert_new.vi"("Path"=path "alert_sound.wav", "Turn on"=w1779) -> ()  [unwired: 2 in, 1 out]
          }
        }
      }
    }
  }
